vi "Missing System Controls Installer.vi"() -> ()   [LabVIEW 2009]
uses:
  <vilib>/registry/registry.llb/Registry RtKey.ctl
  <vilib>/registry/registry.llb/Registry SAM.ctl
  <vilib>/Palette API/Palette Menu/Public Type Define/Item.ctl
  <vilib>/registry/registry.llb/Read Registry Value Simple STR.vi
  <vilib>/Palette API/Palette Menu/Public Type Define/Palette type.ctl
  <vilib>/Palette API/Palette Menu/Palette Menu.lvlib
panel:
  in  "Install Button":bool
  in  "Vertical Cancel Button":bool
  in  "Select version(s) to install into:":i32[](listbox)
  # "Missing System \nControls"
  # "This VI will install the Missing System Control palette set into the version of LabVIEW you choose.\n\nAll of the necessary files have been stored in the form of block diagram data for ease of portability.\n\nNote: run this VI at your own risk - it will modify your palettes.  I can't guarantee it won't do something you don't want it to."
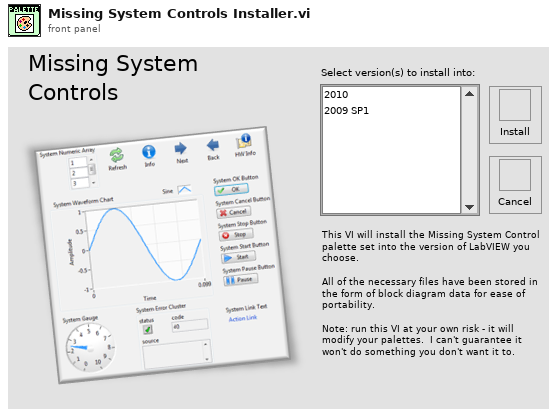
[diagram p1: front panel]
types:
  T1 = typedef "Palette Menu.lvlib/Item.ctl" = cluster{"item path":path, "library path (.lvlib)":path, "use default lvlib palette":bool, "short name":string, "place VI contents":bool, "hide synchronized item":bool, "reserve spot for synch item":bool}
  T2 = typedef "Registry SAM.ctl" = enum32{"KEY_QUERY_VALUE", "KEY_SET_VALUE", "KEY_CREATE_SUB_KEY", "KEY_ENUMERATE_SUB_KEYS", "KEY_NOTIFY", "KEY_CREATE_LINK", "KEY_READ", "KEY_WRITE", "KEY_ALL_ACCESS", "KEY_READ | KEY_WRITE"}
  T3 = typedef "Registry RtKey.ctl" = enum32{"HKEY_CLASSES_ROOT", "HKEY_CURRENT_USER", "HKEY_LOCAL_MACHINE", "HKEY_USERS", "HKEY_PERFORMANCE_DATA", "HKEY_CURRENT_CONFIG", "HKEY_DYN_DATA"}
  T4 = typedef "Registry refnum.ctl" = refnum<k1>
  T5 = cluster{"numSubKeys":i32, "maxSubKeyLen":i32, "maxSubKeyClassLen":i32}
  T6 = typedef "Palette Menu.lvlib/Palette type.ctl" = i32
  T7 = typedef "Palette Menu.lvlib/Palette Data.ctl" = cluster{"display name":string, "view format":T8, "palette width":i16, "items":T9, "256 color icon":picture, "B&W color icon":picture, "help information":T10, "palette description":string, "synchronize information":T11}
  T8 = typedef "Palette Menu.lvlib/View Format.ctl" = u16
  T9 = typedef "Palette Menu.lvlib/Items.ctl" = T1[]
  T10 = typedef "Palette Menu.lvlib/Help Info.ctl" = cluster{"help tag":string, "help file path ":path}
  T11 = typedef "Palette Menu.lvlib/Synchronize Info.ctl" = cluster{"synchronize with directory":bool, "synchronize directory path":path}
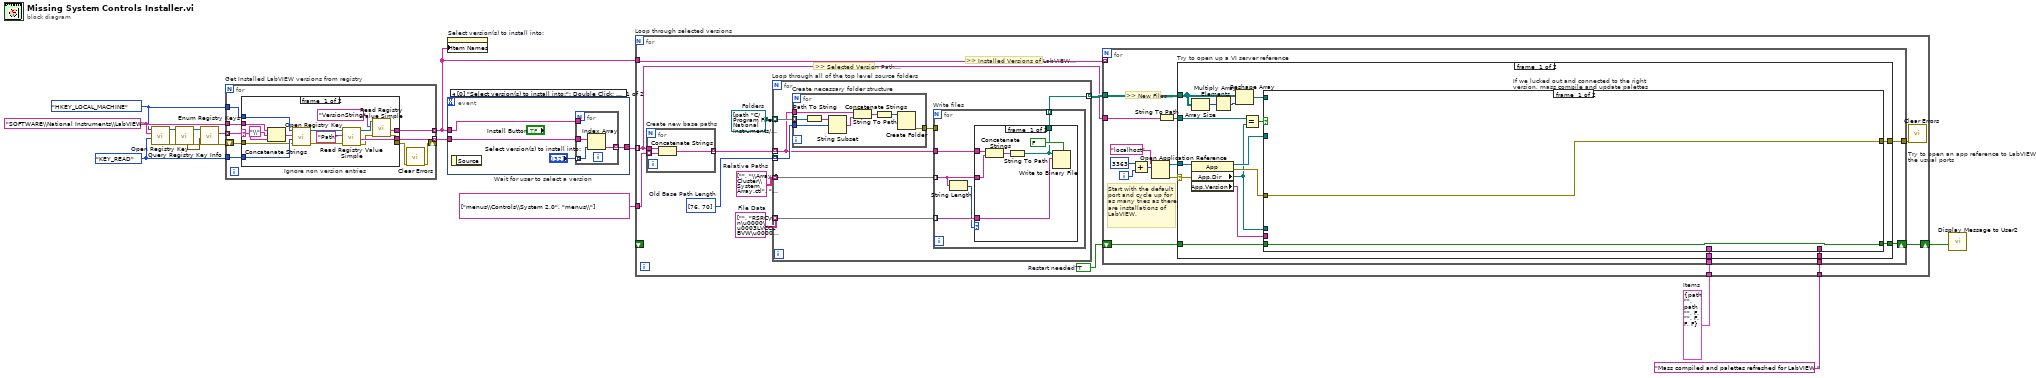
[diagram p0: block diagram]
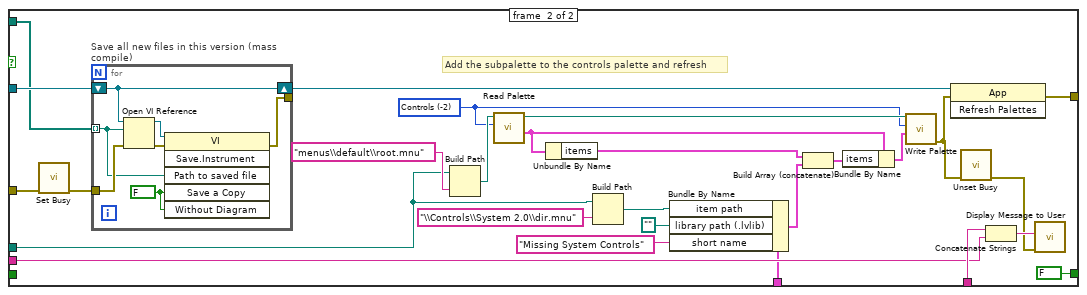
[diagram p2: hidden frame]
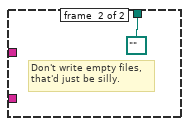
[diagram p4: hidden frame]
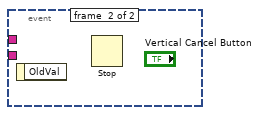
[diagram p5: hidden frame]
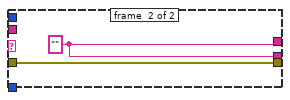
[diagram p6: hidden frame]
diagram:
  w2 = T1 {"item path"=path "", "library path (.lvlib)"=path "", "use default lvlib palette"=FALSE, "short name"="", "place VI contents"=FALSE, "hide synchronized item"=FALSE, "reserve spot for synch item"=FALSE}  # Items
  w11 = Registry_SAM."KEY_READ" ("security access mask (KEY_READ | KEY_WRITE)")
  w12 = Registry_RtKey."HKEY_LOCAL_MACHINE" ("root key (HKEY_LOCAL_MACHINE)")
  w13 = "SOFTWARE\\National Instruments\\LabVIEW" ("subkey")
  n1 = call <vilib>:"Open Registry Key.vi"("security access mask (KEY_READ | KEY_WRITE)"=w11, "subkey"=w13, "root key (HKEY_LOCAL_MACHINE)"=w12) -> ("error out"=w7:errorcluster, "refnum out"=w16:T4)  [unwired: 7 in]
  n2 = call <vilib>:"Query Registry Key Info.vi"("error in (no error)"=w7, "refnum"=w16) -> ("error out"=w6:errorcluster, "refnum out"=w15:T4, "subkey info"=w14:T5)  [unwired: 5 in, 2 out]
  n3 = call <vilib>:"Enum Registry Keys.vi"("error in (no error)"=w6, "subkey info"=w14, "refnum"=w15) -> ("error out"=w5:errorcluster, "subkeys"=w17:string[])  [unwired: 6 in, 1 out]
  n4 = for "Get Installed LabVIEW versions from registry" {
    tunnel: w17 -> [w26] mode=indexing
    tunnel: w13 -> [w25]
    tunnel: w12 -> [w24]
    tunnel: w11 -> [w23]
    tunnel: [w22] -> w8 mode=indexing
    tunnel: [w21] -> w4 mode=indexing
    shift-right: [w18] -> _
    shift-left: w5 -> [w20]
    n5 = case "Ignore non version entries" shown="Default" w26 {
      selector: w26 -> [w32 _]
      tunnel: w25 -> [w42 _]
      tunnel: w24 -> [w40 _]
      tunnel: w23 -> [w39 _]
      tunnel: [w36 w44] -> w22
      tunnel: [w33 w44] -> w21
      tunnel: w20 -> [w30 w43]
      tunnel: [w27 w43] -> w19
      frame #0 {
        n6 = Concatenate Strings(w42, "\\" ("string"), w32) -> (w41:string)
        n7 = call <vilib>:"Open Registry Key.vi"("error in (no error)"=w30, "security access mask (KEY_READ | KEY_WRITE)"=w39, "subkey"=w41, "root key (HKEY_LOCAL_MACHINE)"=w40) -> ("error out"=w29:errorcluster, "refnum out"=w38:T4)  [unwired: 6 in]
        n8 = call-poly <vilib>:"Read Registry Value Simple.vi"("error in (no error)"=w29, "value"="Path" ("subkey"), "refnum"=w38) -> ("error out"=w28:errorcluster, "String/Binary data"=w36:string, "refnum out"=w35:T4)  [unwired: 3 in, 1 out]
        n9 = call-poly <vilib>:"Read Registry Value Simple.vi"("error in (no error)"=w28, "value"="VersionString" ("subkey"), "refnum"=w35) -> ("error out"=w27:errorcluster, "String/Binary data"=w33:string)  [unwired: 3 in, 2 out]
      }
      frame #1 {
        w44 = "" ("String/Binary data")
      }
    }
    n10 = call <vilib>:"Clear Errors.vi"("error in (no error)"=w19) -> ("error out"=w18:errorcluster)  [unwired: 6 in]
  }
  n11 = event "Wait for user to select a version" shown="[0] \"Select version(s) to install into:\": Double Click;  \"Install Button\": Value Change" {
    selector: _ -> [_ _]
    dyn-events: _ -> [_ _]
    timeout: _ -> [_ _]
    tunnel: [w48 _] -> w10
    tunnel: w8 -> [w47 _]
    tunnel: w4 -> [w46 _]
    event #0 {
      n12 = event-data() -> ()  [unwired: 1 in, 1 out]
      n13 = for {
        tunnel: [w51] -> w48 mode=indexing
        tunnel: w47 -> [w50]
        tunnel: w46 -> [_]
        tunnel: "Select version(s) to install into:" -> [w49] mode=indexing
        n14 = Index Array(array=w50, index=w49) -> (element=w51:string)
      }
    }
    event #1 {
      n15 = event-data() -> ()  [unwired: 1 in, 1 out]
      n16 = Stop() -> ()  [unwired: 1 in]
    }
  }
  n17 = property on="Select version(s) to install into:" class="LstBox (strict)"("Item Names"=w4) -> ()  [unwired: 2 in, 2 out]
  n18 = for "Loop through selected versions" {
    tunnel: w10 -> [w57] mode=indexing
    tunnel: string[] ["menus\\Controls\\System 2.0", "menus\\"] -> [w60]
    tunnel: w4 -> [w56]
    tunnel: "Mass compiled and palettes refreshed for LabVIEW " -> [w55]
    tunnel: w2 -> [w54]
    shift-right: [w53] -> w1
    shift-left: _ -> [_]
    w52 = TRUE  # Restart needed?
    w65 = string[][] [["", "\\Array & Cluster\\System Array.ctl", "\\Array & Cluster\\System Cluster.ctl", "\\Array & Cluster\\System Error In.ctl", "\\Array & Cluster\\System Error Out.ctl", "\\Array & Cluster\\System Numeric Array.ctl", "\\Array & Cluster\\System String Array.ctl", "\\Boolean\\System Link Text.ctl", "\\Boolean\\System Buttons\\System Back Button.ctl", "\\Boolean\\System Buttons\\System Cancel Button.ctl", "\\Boolean\\System Buttons\\System Email Button.ctl", "\\Boolean\\System Buttons\\System Info Button.ctl", "\\Boolean\\System Buttons\\System Load Button.ctl", "\\Boolean\\System Buttons\\System Next Button.ctl", "\\Boolean\\System Buttons\\System OK Button.ctl", "\\Boolean\\System Buttons\\System Open Button.ctl", "\\Boolean\\System Buttons\\System Pause Button.ctl", "\\Boolean\\System Buttons\\System Print Button.ctl", "\\Boolean\\System Buttons\\System Refresh Button.ctl", "\\Boolean\\System Buttons\\System Save Button.ctl", "\\Boolean\\System Buttons\\System Save Data Button.ctl", "\\Boolean\\System Buttons\\System Settings Button.ctl", "\\Boolean\\System Buttons\\System Start Button.ctl", "\\Boolean\\System Buttons\\System Stop Button.ctl", "\\Boolean\\Vertical Buttons\\Vertical Add Button.ctl", "\\Boolean\\Vertical Buttons\\Vertical Back Button.ctl", "\\Boolean\\Vertical Buttons\\Vertical Cancel Button.ctl", "\\Boolean\\Vertical Buttons\\Vertical Filter Button.ctl", "\\Boolean\\Vertical Buttons\\Vertical HW Info Button.ctl", "\\Boolean\\Vertical Buttons\\Vertical Info Button.ctl", "\\Boolean\\Vertical Buttons\\Vertical Load Button.ctl", "\\Boolean\\Vertical Buttons\\Vertical Mail Button.ctl", "\\Boolean\\Vertical Buttons\\Vertical Next Button.ctl", "\\Boolean\\Vertical Buttons\\Vertical OK Button.ctl", "\\Boolean\\Vertical Buttons\\Vertical Open Button.ctl", "\\Boolean\\Vertical Buttons\\Vertical Pause Button.ctl", "\\Boolean\\Vertical Buttons\\Vertical Print Button.ctl", "\\Boolean\\Vertical Buttons\\Vertical Record Button.ctl", "\\Boolean\\Vertical Buttons\\Vertical Refresh Button.ctl", "\\Boolean\\Vertical Buttons\\Vertical Remove Button.ctl", "\\Boolean\\Vertical Buttons\\Vertical Save Button.ctl", "\\Boolean\\Vertical Buttons\\Vertical Settings Button.ctl", "\\Boolean\\Vertical Buttons\\Vertical Start Button.ctl", "\\Boolean\\Vertical Buttons\\Vertical Stop Button.ctl", "\\Graphs & Charts\\System Intensity Chart.ctl", "\\Graphs & Charts\\System Waveform Chart.ctl", "\\Graphs & Charts\\System Waveform Graph.ctl", "\\Graphs & Charts\\System XY Graph.ctl", "\\Numeric\\System Dial.ctl", "\\Numeric\\System Gauge.ctl", "\\Numeric\\System Meter.ctl", "\\String & Path\\System String (Transparent).ctl"], ["\\Controls\\System 2.0\\dir.mnu", "\\Controls\\System 2.0\\Array & Cluster\\dir.mnu", "\\Controls\\System 2.0\\Boolean\\dir.mnu", "\\Controls\\System 2.0\\Boolean\\System Buttons\\dir.mnu", "\\Controls\\System 2.0\\Boolean\\Vertical Buttons\\dir.mnu", "\\Controls\\System 2.0\\Graphs & Charts\\dir.mnu", "\\Controls\\System 2.0\\Numeric\\dir.mnu", "\\Controls\\System 2.0\\String & Path\\dir.mnu", "", "", "", "", "", "", "", "", "", "", "", "", "", "", "", "", "", "", "", "", "", "", "", "", "", "", "", "", "", "", "", "", "", "", "", "", "", "", "", "", "", "", "", ""]]  # Relative Paths
    w64 = string[][] [["", "RSRC\r\n\u0000\u0003LVCCLBVW\u0000\u0000'\u0000\u0000\u0003©\u0000\u0000\u0000 \u0000\u0000'd\u0000\u0000\u0000x\t\u0000\u0000\u0000\u0000\u0000\u0000 \u0000\u0000\u0000\u0000\u0000\u0000\u0004\u0000\u0003\u0000<\u0000¼\u0000\u001f@\u0000\u0002\u0000\u0000\u0000\u0000\u0001\u0000\u0001\u0000\u0006ÿÿÿÿ\u0000\u0000\u0000\u0000\u0000\u0000\u0000\u0000\u0000\u0000\u0000\u0000íNñw\u000e)rD.ÆRHÞÌ\u0000\u0000\u0000\n\u0000\u0000\u0000\u0010\u0000\u0000\u0000\u00007Nk½=¢©HÉÝ½#×YÔ\u001dÙ\u0000²\u0004é\tìøB~\u0000\u0000@\u0000\u0000\u0000\u0000\u0000\u0000\u0000\u0000\u0010\u0000\u0000\u0000\u0000\u0000\u0000\u0000\u0000\u0000\u0000\u0000\u0000\u0000\u0000\u0000\u0000\u0000\u0000\u0000 \u0000\u0001LVCC\u0010System Array.ctl\u0000\u0000\u0000\u0000\u0000\u0000\u0000\u0000\u0003\u0000\u0000\u0000\u0002\u0000\u0001\u0000\u0000\u0000\u0000\u0000\u0014\u0000\b\u0000\u0002\u0010\u0000\u0010\u0001 \u0000\u0010\u0000\u0000\u0004\u0010\u00000\u0000\u0010\u0000\u0000\u0000\u0000F\u0000\u0000\u0001,xc`À\u0004ÿ\u0000H12007\u0000i6tñÿPE+Å\u0000Ù\\lv\u0010a/#\u000e\u001an\u0004\u0003\u0003Ó\u0013 Í\u0002Á i¦\u000f@ü\u0003¡\u0013Á\u0000³> [\u0000\u0000\u0000\u0000\u0000 \u0000\u0001VIDS\u0010System Array.ctl\u0000\u0000\u0000\u0000\u0000\u0000\u0000\u0000\u0003\u0000\u0000\u0000x\u0000\u0000\u0000´xsd``È4¶0«`@äüT\u0010½\u0000_3ÄÇEEFÇ\u001e\u0010Ú£Â\u0011\u001c\u0018\u0014\u0016¾\u0011()Ü]Ê°C\u000b(Óé¦±C\tL;ìp\u0004Ó.¡/@æõ¦¨°À´e\u0000ù\u0007æú\u000f\u0004 yF\u0006f\u0006px$·8û»¸\"qÁn\u0002\u00004A'Y\u0000\u0000\u0000\r\t\u0001\u0011\u0000\u0000\u00059.0.1\u0000\u0000\u0000\u0000\u0000\u0000\u0000\u0000\u0000\u0000\u0000\u0000\u0000\u0000\u0000\u0000\u0000\u0000\u0000\u001f÷ÿÿ\u0010\u0014\u0000\u0000\u0011\u0014Fx\u0010\u0014É\u0010\u0011\u0014B0\u0011\u0014D\b\u0011\u0014ïp\u0010\u0014\u0000\u0000\u001fô\u0000\u0000\u0010\u0017ÿÿ\u0011\u0010\u0000\u0000\u0010\u0010\u0000\u0000\u0011\u0010\u0000\u0000\u0011\u0010\u0000\u0000\u0013\u0010\u0000\u0000\u0010\u0010\u0000\u0000\u001fð\u0000\u0000\u0010\u0010\u0000\u0000\u0012\u0010\u0000\u0000\u0012\u0010\u0000\u0000\u0012\u0000\u0000...", "RSRC\r\n\u0000\u0003LVCCLBVW\u0000\u00007\f\u0000\u0000\u0003«\u0000\u0000\u0000 \u0000\u00006ì\u0000\u0000\u0000x\t\u0000\u0000\u0000\u0000\u0000\u0000 \u0000\u0000\u0000\u0000\u0000\u0000\u0004\u0000\u0003\u0000<\u0000¼\u0000\u001f@\u0000\u0002\u0000\u0000\u0000\u0000\u0001\u0000\u0001\u0000\u0006ÿÿÿÿ\u0000\u0000\u0000\u0000\u0000\u0000\u0000\u0000\u0000\u0000\u0000\u0000\u0006D\u0007ÿÅLí\u0003rÈ\rÞ\u0000\u0000\u0000\n\u0000\u0000\u0000\u0010\u0000\u0000\u0000\u0000ÿ\n.íüN\u0013\u001aõÇä?Ô\u001dÙ\u0000²\u0004é\tìøB~\u0000\u0000@\u0000\u0000\u0000\u0000\u0000\u0000\u0000\u0000\u0010\u0000\u0000\u0000\u0000\u0000\u0000\u0000\u0000\u0000\u0000\u0000\u0000\u0000\u0000\u0000\u0000\u0000\u0000\u0000\"\u0000\u0001LVCC\u0012System Cluster.ctl\u0000\u0000\u0000\u0000\u0000\u0000\u0000\u0000\u0003\u0000\u0000\u0000\u0000\u0000\u0002\u0000\u0001\u0000\u0000\u0000\u0000\u0000\u0010\u0000\u0006\u0000\u0002\u0010\u0000\u0010\u0001\u0010\u0000\u0010\u00040\u0000\u0010\u0000\u0000\u0000\u0000<\u0000\u0000\u0001\u0010xc`À\u0004ÿ\u0000H1200¸,èâÿ¡\u0000V\u0001²¹Øì Î^F \u001a¦/\fP\u000f@\u00003*\u0017\bØ°è\u0004\u0000Úç\u001dó\u0000\u0000\u0000\"\u0000\u0001VIDS\u0012System Cluster.ctl\u0000\u0000\u0000\u0000\u0000\u0000\u0000\u0000\u0003\u0000\u0000\u0000\u0000\u0000x\u0000\u0000\u0000´xsd``È4¶0«`@äüT\u0010½\u0000_3ÄÇEEFÇ\u001e\u0010Ú£Â\u0011\u001c\u0018\u0014\u0016¾\u0011()Ü]Ê°C\u000b(Óé¦±C\tL;ìp\u0004Ó.¡/@æõ¦¨°À´e\u0000ù\u0007æú\u000f\u0004 yF\u0006f\u0006px$·8û»¸\"qÁn\u0002\u00004A'Y\u0000\u0000\u0000\u000b\t\u0000$\u0000\u0000\u00039.0\u0000\u0000\u0000\u0000\u0000\u0000\u0000\u0000\u0000\u0000\u0000\u0000\u0000\u0000\u0000\u0000\u0000\u0000\u0000\u0000\u0000?ÿÿþ \u0000\u0000\u0002 \u0000\u0000\u0002 \u0000\u0000\u0002#ÿâ\"\u0000\"\"\u0000\"#ÿâ \u0000\u0000\u0002 \u0000\u0000\u0002 ?ð\u0002  \u0010\u0002  \u0010\u0002 ?ð\u0002 \u0000\u0000\u0002 \u0000\u0000\u0002 \u0000\u0000\u0002 \u0000â!ðâ!ðâ!ðâ!ð\u0000\u0002 \u0000\u0000\u0002...", "RSRC\r\n\u0000\u0003LVCCLBVW\u0000\u0000p\u0000\u0000\u0003à\u0000\u0000\u0000 \u0000\u0000P\u0000\u0000\u0000x\t\u0000\u0000\u0000\u0000\u0000\u0000 \u0000\u0000\u0000\u0000\u0000\u0000\u0004\u0000\u0003\u0000<\u0000¼\u0000\u001f@\u0000\u0002\u0000\u0000\u0000\u0000\u0001\u0000\u0001\u0000\u0006ÿÿÿÿ\u0000\u0000\u0000\u0000\u0000\u0000\u0000\u0000\u0000\u0000\u0000\u0000~ýë¥\u0007\u000bNW\u0007í÷\u001cÜÞ\u0000\u0000\u0000\n\u0000\u0000\u0000\u0010\u0000\u0000\u0000\u0000S\u0017×ûE¶Ö¯tµ.RqÔ\u001dÙ\u0000²\u0004é\tìøB~\u0000\u0000@\u0000\u0000\u0000\u0000\u0000\u0000\u0000\u0000\u0010\u0000\u0000\u0000\u0000\u0000\u0000\u0000\u0000\u0000\u0000\u0000\u0000\u0000\u0000\u0000\u0000\u0000\u0000\u0000\"\u0000\u0001LVCC\u0013System Error In.ctl\u0000\u0000\u0000\u0000\u0000\u0000\u0000\u0003\u0000\u0000\u0000\u0000\u0000\u0002\u0000\u0001\u0000\u0000\u0000\u0000\u0000\u0014\u0000\b\u0000\u0002\u0010\u0000\u0010\u0001\u0010\u0000\u0000\u0004\u0010\u00000\u0000\u0000\b\u0010\u0000\u0000\u0000\u0000@\u0000\u0000\u0001\u0019xc`À\u0004ÿ\u0000H12007\u0000iVtñÿPE+Å\u0000Ù\\lvj/P1Ó\u0005 Í\fÄ\u0010!¦;@ü\u000eY\u0011\u000f\u0016\u0000ê &\u0000\u0000\u0000\"\u0000\u0001VIDS\u0013System Error In.ctl\u0000\u0000\u0000\u0000\u0000\u0000\u0000\u0003\u0000\u0000\u0000\u0000\u0000ê\u0000\u0000\u0001pxûÄÀÀila¦ÉÈ\u0000\u0007Éù)© :\u0006(ö!>.*2:öðÐî\u001c\u0015àÀ °ðî\u0012\u0015î\u001a\u0015óNp00@D]9:]ÿt»òtºþè.ýÓ]û\u001f\u001bÿ>y\u001b;@f°î\u0000Y\næ1ºþÒPµÝöÝfÿPTZï`ªdAVùßü¿Ù\u000bÞ\u0014\u0015\u000e[\u0010\u0003E\u0017+\u0007vôÉÃ\u0013ÂÃ^Dÿÿÿ\u001f¤\u0014?J\u0019vh\u0001\u0015wºiìP\u0002Ó\u000e;>iP\r,0mÛ|\u0013&\u0006\u0006I ñ\u0007\u0018d\u000bÐäÿ u\fÌ@Q\u0000)\u0010ÀÙßÅ\u0015\u000f\nO\u0000ø@cC\u0000\u0000\u0000\u0000\u0000\u000b...", "RSRC\r\n\u0000\u0003LVCCLBVW\u0000\u0000Ô\u0000\u0000\u0003á\u0000\u0000\u0000 \u0000\u0000´\u0000\u0000\u0000x\t\u0000\u0000\u0000\u0000\u0000\u0000 \u0000\u0000\u0000\u0000\u0000\u0000\u0004\u0000\u0003\u0000<\u0000¼\u0000\u001f@\u0000\u0002\u0000\u0000\u0000\u0000\u0001\u0000\u0001\u0000\u0006ÿÿÿÿ\u0000\u0000\u0000\u0000\u0000\u0000\u0000\u0000\u0000\u0000\u0000\u0000³>Í¶\u0010KÙ@Ì\u0001\u0017\u001d\u0000\u0000\u0000\u0000\n\u0000\u0000\u0000\u0010\u0000\u0000\u0000\u0000:\u0007ðvÝ<éF°YÖ~ÂÈÔ\u001dÙ\u0000²\u0004é\tìøB~\u0000\u0000@\u0000\u0000\u0000\u0000\u0000\u0000\u0000\u0000\u0010\u0000\u0000\u0000\u0000\u0000\u0000\u0000\u0000\u0000\u0000\u0000\u0000\u0000\u0000\u0000\u0000\u0000\u0000\u0000$\u0000\u0001LVCC\u0014System Error Out.ctl\u0000\u0000\u0000\u0000\u0000\u0000\u0000\u0000\u0003\u0000\u0000\u0000\u0002\u0000\u0001\u0000\u0000\u0000\u0000\u0000\u0014\u0000\b\u0000\u0002\u0010\u0000\u0010\u0001\u0010\u0000\u0000\u0004\u0010\u00000\u0000\u0000\b\u0010\u0000\u0000\u0000\u0000B\u0000\u0000\u0001\u0019xc`À\u0004ÿ\u0000H12007\u0000iVtñÿPE+Å\u0000Ù\\lvj/P1Ó\u0005 Í\fÄ`?10Ý\u0001âwÈx°h\u0004\u0000\u0014 '\u0000\u0000\u0000\u0000\u0000$\u0000\u0001VIDS\u0014System Error Out.ctl\u0000\u0000\u0000\u0000\u0000\u0000\u0000\u0000\u0003\u0000\u0000\u0000ê\u0000\u0000\u0001pxûÄÀÀila¦ÉÈ\u0000\u0007Éù)© :\u0006(ö!>.*2:öðÐî\u001c\u0015àÀ °ðî\u0012\u0015î\u001a\u0015óNp00@D]9:]ÿt»òtºþè.ýÓ]û\u001f\u001bÿ>y\u001b;@f°î\u0000Y\næ1ºþÒPµÝöÝfÿPTZï`ªdAVùßü¿Ù\u000bÞ\u0014\u0015\u000e[\u0010\u0003E\u0017+\u0007vôÉÃ\u0013ÂÃ^Dÿÿÿ\u001f¤\u0014?J\u0019vh\u0001\u0015wºiìP\u0002Ó\u000e;>iP\r,0mÛ|\u0013&\u0006\u0006I ñ\u0007\u0018d\u000bÐäÿ u\fÌ@Q\u0000)\u0010ÀÙßÅ\u0015\u000f\nO\u0000ø@cC\u0000\u0000...", "RSRC\r\n\u0000\u0003LVCCLBVW\u0000\u0000I\u0000\u0000\u0003±\u0000\u0000\u0000 \u0000\u0000I`\u0000\u0000\u0000x\t\u0000\u0000\u0000\u0000\u0000\u0000 \u0000\u0000\u0000\u0000\u0000\u0000\u0004\u0000\u0003\u0000<\u0000¼\u0000\u001f@\u0000\u0002\u0000\u0000\u0000\u0000\u0001\u0000\u0001\u0000\u0006ÿÿÿÿ\u0000\u0000\u0000\u0000\u0000\u0000\u0000\u0000\u0000\u0000\u0000\u0000ÑµÎ§íy\u0019Lªc},Ó:+T\u0000\u0000\u0000\n\u0000\u0000\u0000\u0010\u0000\u0000\u0000\u0000\"¡à,\u001b&K¥-\u000fcÝsÔ\u001dÙ\u0000²\u0004é\tìøB~\u0000\u0000@\u0000\u0000\u0000\u0000\u0000\u0000\u0000\u0000\u0010\u0000\u0000\u0000\u0000\u0000\u0000\u0000\u0000\u0000\u0000\u0000\u0000\u0000\u0000\u0000\u0000\u0000\u0000\u0000(\u0000\u0001LVCC\u0018System Numeric Array.ctl\u0000\u0000\u0000\u0000\u0000\u0000\u0000\u0000\u0003\u0000\u0000\u0000\u0002\u0000\u0001\u0000\u0000\u0000\u0000\u0000\"\u0000\u000f\u0000\u0002\u0010\u0000\u0010\u0001 \u0000\u0010\u0000\u0000\u0004\u0010\u00000\u0000\u0000\b\u0010\u0000\u0010\b\u0010\u0000\u0010\u0000\u0010\u0000\u0010\u0000\u0010\u0000\u0000\u0000\u0000\u0000\u0000H\u0000\u0000\u00014xc`À\u0004ÿ\u0000H12007\u0000i6tñÿPE+Å\u0000Ù\\lv\u0010a/#\u000e\u001aÃ(\u0006\u0006¦'@\u0005é\u0003\u0010ÿÊs\u0000\u00199±h\u0004\u0000 b\u0000\u0000\u0000(\u0000\u0001VIDS\u0018System Numeric Array.ctl\u0000\u0000\u0000\u0000\u0000\u0000\u0000\u0000\u0003\u0000\u0000\u0001\u000b\u0000\u0000\u0001Ìx\u000bcd`È4¶0ë\u0005Ò0\n¢w\u0000Å^3ÄÇEEFÇ\u001e\u0010Ú£Â\u0011\u001c\u0018\u0014\u0016Þ]¢¢Ò]£¢ÑÍf\u000bRV*}¼õ\u00043Dë>\u0010q¼õ\u0000ûZ´¡óXó1nÎ¹ ÁÎ¹ Ýì`%ò@ÙãÍÇ²Ö`ÙZ6*M°ª×\\\bºÁâ/ËÌ\tT\u0005wÙî²ß<yïfÀý\u0007ó\"ªÙ\f\u000f´¼}Í±\u0003d%ÿ\u0003Uú¥ºÍÇ8sx7ÿf¨¿Ü¼\u0017ìOP¸0°UAJYÁXÂªa\u0016P¦ÓMc...", "RSRC\r\n\u0000\u0003LVCCLBVW\u0000\u0000B\b\u0000\u0000\u0003°\u0000\u0000\u0000 \u0000\u0000Aè\u0000\u0000\u0000x\t\u0000\u0000\u0000\u0000\u0000\u0000 \u0000\u0000\u0000\u0000\u0000\u0000\u0004\u0000\u0003\u0000<\u0000¼\u0000\u001f@\u0000\u0002\u0000\u0000\u0000\u0000\u0001\u0000\u0001\u0000\u0006ÿÿÿÿ\u0000\u0000\u0000\u0000\u0000\u0000\u0000\u0000\u0000\u0000\u0000\u0000üi\u001e¶\u0003\rQB\u0004va\u0010Éá\u0000\u0000\u0000\n\u0000\u0000\u0000\u0010\u0000\u0000\u0000\u0000àÉ½þ^P{KÒz;ù\u0012__Ô\u001dÙ\u0000²\u0004é\tìøB~\u0000\u0000@\u0000\u0000\u0000\u0000\u0000\u0000\u0000\u0000\u0010\u0000\u0000\u0000\u0000\u0000\u0000\u0000\u0000\u0000\u0000\u0000\u0000\u0000\u0000\u0000\u0000\u0000\u0000\u0000&\u0000\u0001LVCC\u0017System String Array.ctl\u0000\u0000\u0000\u0000\u0000\u0000\u0000\u0003\u0000\u0000\u0000\u0000\u0000\u0002\u0000\u0001\u0000\u0000\u0000\u0000\u0000\u0016\u0000\t\u0000\u0002\u0010\u0000\u0010\u0001 \u0000\u0010\u0000\u0000\u0004\u0010\u00000\u0000\u0000\b\u0010\u0000\u0000\u0000\u0000\u0000\u0000H\u0000\u0000\u00010xc`À\u0004ÿ\u0000H12007\u0000i6tñÿPE+Å\u0000Ù\\lv\u0010a/#\u000e\u001aÅ\u0018\u0006\u0006¦'@\u0005é\u0003\u0010ÿÊ\u0003ÅX\u0018ù°h\u0004\u0000%· c\u0000\u0000\u0000&\u0000\u0001VIDS\u0017System String Array.ctl\u0000\u0000\u0000\u0000\u0000\u0000\u0000\u0003\u0000\u0000\u0000\u0000\u0001\u0015\u0000\u0000\u0001àxKbd`È4¶0\t¤a 9?%\u0015D\u0001½f=<!´;G#80(,¼»DE¥»FEã%\u001fPÁ\t\u0011\u0006\u0006¨+G7-H_©èq×/ Æ>\u0010qÜõ\u000fzÍßÍÐy¬ù\u0018K·EgíÎÚ/Ý®<Põ%b@©ÃÍRÖµjòµ_^³Cuv×þyY\u0003¤'Ð\u0002ü7þoö\u0002dKo\n\u0007Ø5;@!QÂº\u0003ì\u0013u \u000eóoþÏP¥¹ö\u000b,_Ê\n\u0016\u0001\u0007ÒÉÃ\u0013ÂÃ^¼þ÷ÿ?È0,áVÊ°C\u000b¨¸ÓMc\u0012v...", "RSRC\r\n\u0000\u0003LVCCLBVW\u0000\u0000Q\u0018\u0000\u0000\u0003­\u0000\u0000\u0000 \u0000\u0000Pø\u0000\u0000\u0000x\t\u0000\u0000\u0000\u0000\u0000\u0000 \u0000\u0000\u0000\u0000\u0000\u0000\u0004\u0000\u0003\u0000<\u0000¼\u0000\u001f@\u0000\u0002\u0000\u0000\u0000\u0000\u0001\u0000\u0001\u0000\u0006ÿÿÿÿ\u0000\u0000\u0000\u0000\u0000\u0000\u0000\u0000\u0000\u0000\u0000\u0000íè´C÷%C¸ÑÝX\u0011<l\u001a\u0000\u0000\u0000\n\u0000\u0000\u0000\u0010\u0000\u0000\u0000\u0000\u001a\u0013ºNÎ{àH¨W\u0012Æs¡{óÔ\u001dÙ\u0000²\u0004é\tìøB~\u0000\u0000@\u0000\u0000\u0000\u0000\u0000\u0000\u0000\u0000\u0010\u0000\u0000\u0000\u0000\u0000\u0000\u0000\u0000\u0000\u0000\u0000\u0000\u0000\u0000\u0000\u0000\u0000\u0000\u0000$\u0000\u0001LVCC\u0014System Link Text.ctl\u0000\u0000\u0000\u0000\u0000\u0000\u0000\u0000\u0003\u0000\u0000\u0000\u0002\u0000\u0001\u0000\u0000\u0000\u0000\u0000\u0014\u0000\b\u0000\u0002\u0010\u0000\u0010\u0001\u0010\u0000\u0010\u0004\u0010\u00000\u0000\u0010\b\u0010\u0000\u0000\u0000\u0000A\u0000\u0000\u0001\u0011xc`À\u0004ÿ\u0000H12007\u0000iVtñÿPE+Å\u0000Ù\\lv\u0010i/#P\u0011Ó\u0007 \u0001ì\u0011\u0010fú\u0003ÄÿPTaÑ\t\u0000´Ò e\u0000\u0000\u0000\u0000\u0000\u0000$\u0000\u0001VIDS\u0014System Link Text.ctl\u0000\u0000\u0000\u0000\u0000\u0000\u0000\u0000\u0003\u0000\u0000\u0000\u0000\u0000\u0000Ôxg``È4¶0Æ\u0000Éù)© ú\u0000\u0010¿f=<!´;G#80(,¼»DE¥»FE\u001f\u001bÿ>y\u001b;\u0018\nKXwô²yX42ìÐ\u0002ÊtºiìP\u0002Ó\u000e;âÁ´Kè\u000bÎÞ\u0014\u0015\u0016¶6 ÿ Ð\u001cQÿ\u0000$ÏÈÀÌËPÊPË\fý]\\ù 7\u0003\u0000Â\u000308\u0000\u0000\u0000\u0000\u0000\u0000\r\t\u0001\u0011\u0000\u0000\u00059.0.1\u0000\u0000\u0000\u0000\u0000\u0000\u0000\u0000\u0000\u0000\u0000\u0000\u0000\u0000\u0000\u0000\u0000\u0000\u0000\u0000\u0000\u0000\u0000\u0000\u0000\u0000\u0000\u0000\u0000\u0000\u0000\u0000\u0000\u0000\u0000\u0000\u0000\u0000\u0000\u0000@\u0000\u0000À\b\u0000\u0000 \b\u0000\u0001!Þ\u0001#\b\u0001\u0012\b\u0003ò\b\u0002\u0013\b...", "RSRC\r\n\u0000\u0003LVCCLBVW\u0000\u00002¨\u0000\u0000\u0003Ï\u0000\u0000\u0000 \u0000\u00002\u0000\u0000\u0000x\t\u0000\u0000\u0000\u0000\u0000\u0000 \u0000\u0000\u0000\u0000\u0000\u0000\u0004\u0000\u0003\u0000<\u0000¼\u0000\u001f@\u0000\u0002\u0000\u0000\u0000\u0000\u0001\u0000\u0001\u0000\u0006ÿÿÿÿ\u0000\u0000\u0000\u0000\u0000\u0000\u0000\u0000\u0000\u0000\u0000\u0000ñM|\u0011è(I·\u001b\u001a'«ýÑ\u0000\u0000\u0000\n\u0000\u0000\u0000\u0010\u0000\u0000\u0000\u0000yL_FÈ\nm@´\u001a\u0012Fv)SÔ\u001dÙ\u0000²\u0004é\tìøB~\u0000\u0000@\u0000\u0000\u0000\u0000\u0000\u0000\u0000\u0000\u0010\u0000\u0000\u0000\u0000\u0000\u0000\u0000\u0000\u0000\u0000\u0000\u0000\u0000\u0000\u0000\u0000\u0000\u0000\u0000&\u0000\u0001LVCC\u0016System Back Button.ctl\u0000\u0000\u0000\u0000\u0000\u0000\u0000\u0000\u0003\u0000\u0000\u0000\u0000\u0000\u0002\u0000\u0001\u0000\u0000\u0000\u0000\u0000\u0014\u0000\b\u0000\u0002\u0010\u0000\u0010\u0001\u0010\u0000\u0010\u0004\u0010\u00000\u0000\u0010\b\u0010\u0000\u0000\u0000\u0000A\u0000\u0000\u0001\u0011xc`À\u0004ÿ\u0000H12007\u0000iVtñÿPE+Å\u0000Ù\\lv\u0010i/#P\u0011Ó\u0007 \u0001ì\u0011\u0010fú\u0003ÄÿPTaÑ\t\u0000´Ò e\u0000\u0000\u0000\u0000\u0000\u0000&\u0000\u0001VIDS\u0016System Back Button.ctl\u0000\u0000\u0000\u0000\u0000\u0000\u0000\u0000\u0003\u0000\u0000\u0000\u0000\u0000\u0000\u0000\u0000Ôxg``È4¶0Æ\u0000Éù)© ú\u0000\u0010¿f=<!´;G#80(,¼»DE¥»FE\u001f\u001bÿ>y\u001b;\u0018\nKXwô²yX42ìÐ\u0002ÊtºiìP\u0002Ó\u000e;âÁ´Kè\u000bÎÞ\u0014\u0015\u0016¶6 ÿ Ð\u001cQÿ\u0000$ÏÈÀÌËPÊPË\fý]\\ù 7\u0003\u0000Â\u000308\u0000\u0000\u0000\u0000\u0000\u0000\r\t\u0001\u0011\u0000\u0000\u00059.0.1\u0000\u0000\u0000\u0000\u0000\u0000\u0000\u0000\u0000\u0000\u0000\u0000\u0000\u0000\u0000\u000fÿÿÿ\u0000\u0000\u0000\u0000 \u0000\u0000\u0000 \u0000\u0000 \u0001\u0000 \u0006\u0000 \fþ\u0000 \u001b\u0002\u0000 7ú\u0000 ú\u0000 ?þ\u0000 \u001fþ\u0000...", "RSRC\r\n\u0000\u0003LVCCLBVW\u0000\u0000. \u0000\u0000\u0003Ñ\u0000\u0000\u0000 \u0000\u0000.\u0000\u0000\u0000x\t\u0000\u0000\u0000\u0000\u0000\u0000 \u0000\u0000\u0000\u0000\u0000\u0000\u0004\u0000\u0003\u0000<\u0000¼\u0000\u001f@\u0000\u0002\u0000\u0000\u0000\u0000\u0001\u0000\u0001\u0000\u0006ÿÿÿÿ\u0000\u0000\u0000\u0000\u0000\u0000\u0000\u0000\u0000\u0000\u0000\u0000z\u001a3ëÊsI­Ïkov\u0000\u0000\u0000\n\u0000\u0000\u0000\u0010\u0000\u0000\u0000\u0000\u001dÊ·«4J¸'EtXXZÔ\u001dÙ\u0000²\u0004é\tìøB~\u0000\u0000@\u0000\u0000\u0000\u0000\u0000\u0000\u0000\u0000\u0010\u0000\u0000\u0000\u0000\u0000\u0000\u0000\u0000\u0000\u0000\u0000\u0000\u0000\u0000\u0000\u0000\u0000\u0000\u0000(\u0000\u0001LVCC\u0018System Cancel Button.ctl\u0000\u0000\u0000\u0000\u0000\u0000\u0000\u0000\u0003\u0000\u0000\u0000\u0002\u0000\u0001\u0000\u0000\u0000\u0000\u0000\u0014\u0000\b\u0000\u0002\u0010\u0000\u0010\u0001\u0010\u0000\u0010\u0004\u0010\u00000\u0000\u0010\b\u0010\u0000\u0000\u0000\u0000A\u0000\u0000\u0001\u0011xc`À\u0004ÿ\u0000H12007\u0000iVtñÿPE+Å\u0000Ù\\lv\u0010i/#P\u0011Ó\u0007 \u0001ì\u0011\u0010fú\u0003ÄÿPTaÑ\t\u0000´Ò e\u0000\u0000\u0000\u0000\u0000\u0000(\u0000\u0001VIDS\u0018System Cancel Button.ctl\u0000\u0000\u0000\u0000\u0000\u0000\u0000\u0000\u0003\u0000\u0000\u0000\u0000\u0000\u0000Ôxg``È4¶0Æ\u0000Éù)© ú\u0000\u0010¿f=<!´;G#80(,¼»DE¥»FE\u001f\u001bÿ>y\u001b;\u0018\nKXwô²yX42ìÐ\u0002ÊtºiìP\u0002Ó\u000e;âÁ´Kè\u000bÎÞ\u0014\u0015\u0016¶6 ÿ Ð\u001cQÿ\u0000$ÏÈÀÌËPÊPË\fý]\\ù 7\u0003\u0000Â\u000308\u0000\u0000\u0000\u0000\u0000\u0000\r\t\u0001\u0011\u0000\u0000\u00059.0.1\u0000\u0000\u0000\u0000\u0000\u0000\u0000\u0000\u0000\u0000\u0000\u0000\u0000\u0000\u0000\u000fÿÿÿ\u0000\u0000\u0000\u0000 \u0000\u0000\u0000 \u0000\u0000\u0000 \u0000\u0000\u0000 $$\u0000 \"D\u0000 \u0011\u0001 \b\u0010\u0002 \u0004 \u0002 \f0\u0002 \u0018\u0018\u0002...", "RSRC\r\n\u0000\u0003LVCCLBVW\u0000\u0000,h\u0000\u0000\u0003Ð\u0000\u0000\u0000 \u0000\u0000,H\u0000\u0000\u0000x\t\u0000\u0000\u0000\u0000\u0000\u0000 \u0000\u0000\u0000\u0000\u0000\u0000\u0004\u0000\u0003\u0000<\u0000¼\u0000\u001f@\u0000\u0002\u0000\u0000\u0000\u0000\u0001\u0000\u0001\u0000\u0006ÿÿÿÿ\u0000\u0000\u0000\u0000\u0000\u0000\u0000\u0000\u0000\u0000\u0000\u0000Éø|\u001fqá\u0019L©\rË2\u0016úo\u0000\u0000\u0000\n\u0000\u0000\u0000\u0010\u0000\u0000\u0000\u0000·ì@FOq7C¡\u001f°Ô\u001dÙ\u0000²\u0004é\tìøB~\u0000\u0000@\u0000\u0000\u0000\u0000\u0000\u0000\u0000\u0000\u0010\u0000\u0000\u0000\u0000\u0000\u0000\u0000\u0000\u0000\u0000\u0000\u0000\u0000\u0000\u0000\u0000\u0000\u0000\u0000&\u0000\u0001LVCC\u0017System Email Button.ctl\u0000\u0000\u0000\u0000\u0000\u0000\u0000\u0003\u0000\u0000\u0000\u0000\u0000\u0002\u0000\u0001\u0000\u0000\u0000\u0000\u0000\u0014\u0000\b\u0000\u0002\u0010\u0000\u0010\u0001\u0010\u0000\u0010\u0004\u0010\u00000\u0000\u0010\b\u0010\u0000\u0000\u0000\u0000A\u0000\u0000\u0001\u0011xc`À\u0004ÿ\u0000H12007\u0000iVtñÿPE+Å\u0000Ù\\lv\u0010i/#P\u0011Ó\u0007 \u0001ì\u0011\u0010fú\u0003ÄÿPTaÑ\t\u0000´Ò e\u0000\u0000\u0000\u0000\u0000\u0000&\u0000\u0001VIDS\u0017System Email Button.ctl\u0000\u0000\u0000\u0000\u0000\u0000\u0000\u0003\u0000\u0000\u0000\u0000\u0000\u0000\u0000\u0000Ôxg``È4¶0Æ\u0000Éù)© ú\u0000\u0010¿f=<!´;G#80(,¼»DE¥»FE\u001f\u001bÿ>y\u001b;\u0018\nKXwô²yX42ìÐ\u0002ÊtºiìP\u0002Ó\u000e;âÁ´Kè\u000bÎÞ\u0014\u0015\u0016¶6 ÿ Ð\u001cQÿ\u0000$ÏÈÀÌËPÊPË\fý]\\ù 7\u0003\u0000Â\u000308\u0000\u0000\u0000\u0000\u0000\u0000\r\t\u0001\u0011\u0000\u0000\u00059.0.1\u0000\u0000\u0000\u0000\u0000\u0000\u0000\u0000\u0000\u0000\u0000\u0000\u0000\u0000\u0000\u000fÿÿÿ\u0000\u0000\u0000\u0000 \u0000\u0000\u0000 \u0000\u0000\u0000 \u0000\u0000 \u0000\u0001\u0000 \u0000\u0001\u0000 \u0000\u0001\u0000 \u0000\u0001\u0000 \u0011\u0000 \t\u0000 Å\u0000...", "RSRC\r\n\u0000\u0003LVCCLBVW\u0000\u0000+Ì\u0000\u0000\u0003Ï\u0000\u0000\u0000 \u0000\u0000+¬\u0000\u0000\u0000x\t\u0000\u0000\u0000\u0000\u0000\u0000 \u0000\u0000\u0000\u0000\u0000\u0000\u0004\u0000\u0003\u0000<\u0000¼\u0000\u001f@\u0000\u0002\u0000\u0000\u0000\u0000\u0001\u0000\u0001\u0000\u0006ÿÿÿÿ\u0000\u0000\u0000\u0000\u0000\u0000\u0000\u0000\u0000\u0000\u0000\u0000ør·MÙþ@´²ç)×ÜY\u0000\u0000\u0000\n\u0000\u0000\u0000\u0010\u0000\u0000\u0000\u0000Hð[dÙE¶yÊy¢½Ô\u001dÙ\u0000²\u0004é\tìøB~\u0000\u0000@\u0000\u0000\u0000\u0000\u0000\u0000\u0000\u0000\u0010\u0000\u0000\u0000\u0000\u0000\u0000\u0000\u0000\u0000\u0000\u0000\u0000\u0000\u0000\u0000\u0000\u0000\u0000\u0000&\u0000\u0001LVCC\u0016System Info Button.ctl\u0000\u0000\u0000\u0000\u0000\u0000\u0000\u0000\u0003\u0000\u0000\u0000\u0000\u0000\u0002\u0000\u0001\u0000\u0000\u0000\u0000\u0000\u0014\u0000\b\u0000\u0002\u0010\u0000\u0010\u0001\u0010\u0000\u0010\u0004\u0010\u00000\u0000\u0010\b\u0010\u0000\u0000\u0000\u0000A\u0000\u0000\u0001\u0011xc`À\u0004ÿ\u0000H12007\u0000iVtñÿPE+Å\u0000Ù\\lv\u0010i/#P\u0011Ó\u0007 \u0001ì\u0011\u0010fú\u0003ÄÿPTaÑ\t\u0000´Ò e\u0000\u0000\u0000\u0000\u0000\u0000&\u0000\u0001VIDS\u0016System Info Button.ctl\u0000\u0000\u0000\u0000\u0000\u0000\u0000\u0000\u0003\u0000\u0000\u0000\u0000\u0000\u0000\u0000\u0000Ôxg``È4¶0Æ\u0000Éù)© ú\u0000\u0010¿f=<!´;G#80(,¼»DE¥»FE\u001f\u001bÿ>y\u001b;\u0018\nKXwô²yX42ìÐ\u0002ÊtºiìP\u0002Ó\u000e;âÁ´Kè\u000bÎÞ\u0014\u0015\u0016¶6 ÿ Ð\u001cQÿ\u0000$ÏÈÀÌËPÊPË\fý]\\ù 7\u0003\u0000Â\u000308\u0000\u0000\u0000\u0000\u0000\u0000\r\t\u0001\u0011\u0000\u0000\u00059.0.1\u0000\u0000\u0000\u0000\u0000\u0000\u0000\u0000\u0000\u0000\u0000\u0000\u0000\u0000\u0000\u000fÿÿÿ\u0000\u0000\u0000\u0000 \u0000\u0000\u0000 \u0003À\u0000 \b\u0010\u0000 \u0010\b\u0000  \u0004\u0000 2D\u0000 þ\u0000 |~\u0000 ~~\u0000 ~~\u0000...", "RSRC\r\n\u0000\u0003LVCCLBVW\u0000\u00008Ô\u0000\u0000\u0003Ï\u0000\u0000\u0000 \u0000\u00008´\u0000\u0000\u0000x\t\u0000\u0000\u0000\u0000\u0000\u0000 \u0000\u0000\u0000\u0000\u0000\u0000\u0004\u0000\u0003\u0000<\u0000¼\u0000\u001f@\u0000\u0002\u0000\u0000\u0000\u0000\u0001\u0000\u0001\u0000\u0006ÿÿÿÿ\u0000\u0000\u0000\u0000\u0000\u0000\u0000\u0000\u0000\u0000\u0000\u0000õæî¯ÄÔºMÚ\u0003\u001e\u001fY.á\u0000\u0000\u0000\n\u0000\u0000\u0000\u0010\u0000\u0000\u0000\u0000<dºômÂH\u0011|Ø-P\t*Ô\u001dÙ\u0000²\u0004é\tìøB~\u0000\u0000@\u0000\u0000\u0000\u0000\u0000\u0000\u0000\u0000\u0010\u0000\u0000\u0000\u0000\u0000\u0000\u0000\u0000\u0000\u0000\u0000\u0000\u0000\u0000\u0000\u0000\u0000\u0000\u0000&\u0000\u0001LVCC\u0016System Load Button.ctl\u0000\u0000\u0000\u0000\u0000\u0000\u0000\u0000\u0003\u0000\u0000\u0000\u0000\u0000\u0002\u0000\u0001\u0000\u0000\u0000\u0000\u0000\u0014\u0000\b\u0000\u0002\u0010\u0000\u0010\u0001\u0010\u0000\u0010\u0004\u0010\u00000\u0000\u0010\b\u0010\u0000\u0000\u0000\u0000A\u0000\u0000\u0001\u0011xc`À\u0004ÿ\u0000H12007\u0000iVtñÿPE+Å\u0000Ù\\lv\u0010i/#P\u0011Ó\u0007 \u0001ì\u0011\u0010fú\u0003ÄÿPTaÑ\t\u0000´Ò e\u0000\u0000\u0000\u0000\u0000\u0000&\u0000\u0001VIDS\u0016System Load Button.ctl\u0000\u0000\u0000\u0000\u0000\u0000\u0000\u0000\u0003\u0000\u0000\u0000\u0000\u0000\u0000\u0000\u0000Ôxg``È4¶0Æ\u0000Éù)© ú\u0000\u0010¿f=<!´;G#80(,¼»DE¥»FE\u001f\u001bÿ>y\u001b;\u0018\nKXwô²yX42ìÐ\u0002ÊtºiìP\u0002Ó\u000e;âÁ´Kè\u000bÎÞ\u0014\u0015\u0016¶6 ÿ Ð\u001cQÿ\u0000$ÏÈÀÌËPÊPË\fý]\\ù 7\u0003\u0000Â\u000308\u0000\u0000\u0000\u0000\u0000\u0000\r\t\u0001\u0011\u0000\u0000\u00059.0.1\u0000\u0000\u0000\u0000\u0000\u0000\u0000\u0000\u0000\u0000\u0000\u0000\u0000\u0000\u0000\u000fÿÿÿ\u0000\u0000\u0000\u0000 \u0000\u0000\u0000 \u0000\u0000\u0000 \u0000\u0000\u0000 \u0000\u0000\u0000 \u0004\u0000\u0000 \u0004\u0000\u0000 \u0004\u0000\u0000 \u0004\u0000\u0000 8\u0012\u0000  \u0002\u0000...", "RSRC\r\n\u0000\u0003LVCCLBVW\u0000\u0000+x\u0000\u0000\u0003Ï\u0000\u0000\u0000 \u0000\u0000+X\u0000\u0000\u0000x\t\u0000\u0000\u0000\u0000\u0000\u0000 \u0000\u0000\u0000\u0000\u0000\u0000\u0004\u0000\u0003\u0000<\u0000¼\u0000\u001f@\u0000\u0002\u0000\u0000\u0000\u0000\u0001\u0000\u0001\u0000\u0006ÿÿÿÿ\u0000\u0000\u0000\u0000\u0000\u0000\u0000\u0000\u0000\u0000\u0000\u0000=âúÑð0Aá\u0007übRÚ\u0000\u0000\u0000\n\u0000\u0000\u0000\u0010\u0000\u0000\u0000\u0000b\u0005\u000bß\nwL6ÙØD?Ô\u001dÙ\u0000²\u0004é\tìøB~\u0000\u0000@\u0000\u0000\u0000\u0000\u0000\u0000\u0000\u0000\u0010\u0000\u0000\u0000\u0000\u0000\u0000\u0000\u0000\u0000\u0000\u0000\u0000\u0000\u0000\u0000\u0000\u0000\u0000\u0000&\u0000\u0001LVCC\u0016System Next Button.ctl\u0000\u0000\u0000\u0000\u0000\u0000\u0000\u0000\u0003\u0000\u0000\u0000\u0000\u0000\u0002\u0000\u0001\u0000\u0000\u0000\u0000\u0000\u0014\u0000\b\u0000\u0002\u0010\u0000\u0010\u0001\u0010\u0000\u0010\u0004\u0010\u00000\u0000\u0010\b\u0010\u0000\u0000\u0000\u0000A\u0000\u0000\u0001\u0011xc`À\u0004ÿ\u0000H12007\u0000iVtñÿPE+Å\u0000Ù\\lv\u0010i/#P\u0011Ó\u0007 \u0001ì\u0011\u0010fú\u0003ÄÿPTaÑ\t\u0000´Ò e\u0000\u0000\u0000\u0000\u0000\u0000&\u0000\u0001VIDS\u0016System Next Button.ctl\u0000\u0000\u0000\u0000\u0000\u0000\u0000\u0000\u0003\u0000\u0000\u0000\u0000\u0000\u0000\u0000\u0000Ôxg``È4¶0Æ\u0000Éù)© ú\u0000\u0010¿f=<!´;G#80(,¼»DE¥»FE\u001f\u001bÿ>y\u001b;\u0018\nKXwô²yX42ìÐ\u0002ÊtºiìP\u0002Ó\u000e;âÁ´Kè\u000bÎÞ\u0014\u0015\u0016¶6 ÿ Ð\u001cQÿ\u0000$ÏÈÀÌËPÊPË\fý]\\ù 7\u0003\u0000Â\u000308\u0000\u0000\u0000\u0000\u0000\u0000\r\t\u0001\u0011\u0000\u0000\u00059.0.1\u0000\u0000\u0000\u0000\u0000\u0000\u0000\u0000\u0000\u0000\u0000\u0000\u0000\u0000\u0000\u000fÿÿÿ\u0000\u0000\u0000\u0000 \u0000\u0000\u0000 \u0001\u0000\u0000 \u0001À\u0000 \u0001`\u0000 0\u0000 @Ø\u0000 _ì\u0000 _þ\u0000 ü\u0000 ø\u0000...", "RSRC\r\n\u0000\u0003LVCCLBVW\u0000\u00000\u0018\u0000\u0000\u0003Í\u0000\u0000\u0000 \u0000\u0000/ø\u0000\u0000\u0000x\t\u0000\u0000\u0000\u0000\u0000\u0000 \u0000\u0000\u0000\u0000\u0000\u0000\u0004\u0000\u0003\u0000<\u0000¼\u0000\u001f@\u0000\u0002\u0000\u0000\u0000\u0000\u0001\u0000\u0001\u0000\u0006ÿÿÿÿ\u0000\u0000\u0000\u0000\u0000\u0000\u0000\u0000\u0000\u0000\u0000\u0000\u000e#5»ã}L\"ÒÿÊ\u0000\u0000\u0000\n\u0000\u0000\u0000\u0010\u0000\u0000\u0000\u0000®\u001e\nÜ\u0006ºÔN¥Â]»ÎuÏóÔ\u001dÙ\u0000²\u0004é\tìøB~\u0000\u0000@\u0000\u0000\u0000\u0000\u0000\u0000\u0000\u0000\u0010\u0000\u0000\u0000\u0000\u0000\u0000\u0000\u0000\u0000\u0000\u0000\u0000\u0000\u0000\u0000\u0000\u0000\u0000\u0000$\u0000\u0001LVCC\u0014System OK Button.ctl\u0000\u0000\u0000\u0000\u0000\u0000\u0000\u0000\u0003\u0000\u0000\u0000\u0002\u0000\u0001\u0000\u0000\u0000\u0000\u0000\u0014\u0000\b\u0000\u0002\u0010\u0000\u0010\u0001\u0010\u0000\u0010\u0004\u0010\u00000\u0000\u0010\b\u0010\u0000\u0000\u0000\u0000A\u0000\u0000\u0001\u0011xc`À\u0004ÿ\u0000H12007\u0000iVtñÿPE+Å\u0000Ù\\lv\u0010i/#P\u0011Ó\u0007 \u0001ì\u0011\u0010fú\u0003ÄÿPTaÑ\t\u0000´Ò e\u0000\u0000\u0000\u0000\u0000\u0000$\u0000\u0001VIDS\u0014System OK Button.ctl\u0000\u0000\u0000\u0000\u0000\u0000\u0000\u0000\u0003\u0000\u0000\u0000\u0000\u0000\u0000Ôxg``È4¶0Æ\u0000Éù)© ú\u0000\u0010¿f=<!´;G#80(,¼»DE¥»FE\u001f\u001bÿ>y\u001b;\u0018\nKXwô²yX42ìÐ\u0002ÊtºiìP\u0002Ó\u000e;âÁ´Kè\u000bÎÞ\u0014\u0015\u0016¶6 ÿ Ð\u001cQÿ\u0000$ÏÈÀÌËPÊPË\fý]\\ù 7\u0003\u0000Â\u000308\u0000\u0000\u0000\u0000\u0000\u0000\r\t\u0001\u0011\u0000\u0000\u00059.0.1\u0000\u0000\u0000\u0000\u0000\u0000\u0000\u0000\u0000\u0000\u0000\u0000\u0000\u0000\u0000\u000fÿÿÿ\u0000\u0000\u0000\u0000 \u0000\u0000\u0000 \u0000\u0000\u0000 \u0000\u0000\u0000 \u0000\u0000\u0000 \u0000\u000e\u0000 \u0000\u000e\u0000 \u0000\u001c\u0000 \u00008\u0000 \u00000\u0000   \u0000 \u0010\u0000\u0000 \u0000\u0000\u0000...", "RSRC\r\n\u0000\u0003LVCCLBVW\u0000\u00005\u0000\u0000\u0003Ï\u0000\u0000\u0000 \u0000\u00005l\u0000\u0000\u0000x\t\u0000\u0000\u0000\u0000\u0000\u0000 \u0000\u0000\u0000\u0000\u0000\u0000\u0004\u0000\u0003\u0000<\u0000¼\u0000\u001f@\u0000\u0002\u0000\u0000\u0000\u0000\u0001\u0000\u0001\u0000\u0006ÿÿÿÿ\u0000\u0000\u0000\u0000\u0000\u0000\u0000\u0000\u0000\u0000\u0000\u0000¬\u0018\u0004$.@®ÃÈ\u0011\u000b_\fÒ\u0000\u0000\u0000\n\u0000\u0000\u0000\u0010\u0000\u0000\u0000\u0000)óá0C»¦ãKÔ\u001dÙ\u0000²\u0004é\tìøB~\u0000\u0000@\u0000\u0000\u0000\u0000\u0000\u0000\u0000\u0000\u0010\u0000\u0000\u0000\u0000\u0000\u0000\u0000\u0000\u0000\u0000\u0000\u0000\u0000\u0000\u0000\u0000\u0000\u0000\u0000&\u0000\u0001LVCC\u0016System Open Button.ctl\u0000\u0000\u0000\u0000\u0000\u0000\u0000\u0000\u0003\u0000\u0000\u0000\u0000\u0000\u0002\u0000\u0001\u0000\u0000\u0000\u0000\u0000\u0014\u0000\b\u0000\u0002\u0010\u0000\u0010\u0001\u0010\u0000\u0010\u0004\u0010\u00000\u0000\u0010\b\u0010\u0000\u0000\u0000\u0000A\u0000\u0000\u0001\u0011xc`À\u0004ÿ\u0000H12007\u0000iVtñÿPE+Å\u0000Ù\\lv\u0010i/#P\u0011Ó\u0007 \u0001ì\u0011\u0010fú\u0003ÄÿPTaÑ\t\u0000´Ò e\u0000\u0000\u0000\u0000\u0000\u0000&\u0000\u0001VIDS\u0016System Open Button.ctl\u0000\u0000\u0000\u0000\u0000\u0000\u0000\u0000\u0003\u0000\u0000\u0000\u0000\u0000\u0000\u0000\u0000Ôxg``È4¶0Æ\u0000Éù)© ú\u0000\u0010¿f=<!´;G#80(,¼»DE¥»FE\u001f\u001bÿ>y\u001b;\u0018\nKXwô²yX42ìÐ\u0002ÊtºiìP\u0002Ó\u000e;âÁ´Kè\u000bÎÞ\u0014\u0015\u0016¶6 ÿ Ð\u001cQÿ\u0000$ÏÈÀÌËPÊPË\fý]\\ù 7\u0003\u0000Â\u000308\u0000\u0000\u0000\u0000\u0000\u0000\r\t\u0001\u0011\u0000\u0000\u00059.0.1\u0000\u0000\u0000\u0000\u0000\u0000\u0000\u0000\u0000\u0000\u0000\u0000\u0000\u0000\u0000\u000fÿÿÿ\u0000\u0000\u0000\u0000 \u0000\u0000\u0000 \u0000\u0000\u0000 \u0000\u0000\u0000 \u0000\u0000\u0000 \u0000\u0000\u0000 \u0000\u0000\u0000 \u0000\u0000\u0000 \u0000\u0000\u0000 \u0000\u0000\u0000 \u0000\u0000\u0000...", "RSRC\r\n\u0000\u0003LVCCLBVW\u0000\u0000($\u0000\u0000\u0003Ð\u0000\u0000\u0000 \u0000\u0000(\u0004\u0000\u0000\u0000x\t\u0000\u0000\u0000\u0000\u0000\u0000 \u0000\u0000\u0000\u0000\u0000\u0000\u0004\u0000\u0003\u0000<\u0000¼\u0000\u001f@\u0000\u0002\u0000\u0000\u0000\u0000\u0001\u0000\u0001\u0000\u0006ÿÿÿÿ\u0000\u0000\u0000\u0000\u0000\u0000\u0000\u0000\u0000\u0000\u0000\u0000|-oÑYTJ ásúX¤h\u0001\u0000\u0000\u0000\n\u0000\u0000\u0000\u0010\u0000\u0000\u0000\u0000H\u0015ªá4óTN¯Rá¨÷¯b4Ô\u001dÙ\u0000²\u0004é\tìøB~\u0000\u0000@\u0000\u0000\u0000\u0000\u0000\u0000\u0000\u0000\u0010\u0000\u0000\u0000\u0000\u0000\u0000\u0000\u0000\u0000\u0000\u0000\u0000\u0000\u0000\u0000\u0000\u0000\u0000\u0000&\u0000\u0001LVCC\u0017System Pause Button.ctl\u0000\u0000\u0000\u0000\u0000\u0000\u0000\u0003\u0000\u0000\u0000\u0000\u0000\u0002\u0000\u0001\u0000\u0000\u0000\u0000\u0000\u0014\u0000\b\u0000\u0002\u0010\u0000\u0010\u0001\u0010\u0000\u0010\u0004\u0010\u00000\u0000\u0010\b\u0010\u0000\u0000\u0000\u0000A\u0000\u0000\u0001\u0011xc`À\u0004ÿ\u0000H12007\u0000iVtñÿPE+Å\u0000Ù\\lv\u0010i/#P\u0011Ó\u0007 \u0001ì\u0011\u0010fú\u0003ÄÿPTaÑ\t\u0000´Ò e\u0000\u0000\u0000\u0000\u0000\u0000&\u0000\u0001VIDS\u0017System Pause Button.ctl\u0000\u0000\u0000\u0000\u0000\u0000\u0000\u0003\u0000\u0000\u0000\u0000\u0000\u0000\u0000\u0000Ôxg``È4¶0Æ\u0000Éù)© ú\u0000\u0010¿f=<!´;G#80(,¼»DE¥»FE\u001f\u001bÿ>y\u001b;\u0018\nKXwô²yX42ìÐ\u0002ÊtºiìP\u0002Ó\u000e;âÁ´Kè\u000bÎÞ\u0014\u0015\u0016¶6 ÿ Ð\u001cQÿ\u0000$ÏÈÀÌËPÊPË\fý]\\ù 7\u0003\u0000Â\u000308\u0000\u0000\u0000\u0000\u0000\u0000\r\t\u0001\u0011\u0000\u0000\u00059.0.1\u0000\u0000\u0000\u0000\u0000\u0000\u0000\u0000\u0000\u0000\u0000\u0000\u0000\u0000\u0000\u0000\u0000\u0000\u0000\u0007ÿÿÿ\u0000\u0000\u0000\u0000\u0010~\u000f\u0010B\u0010\u0010B\u0010\u0010B\u0010\u0010B\u0018\u0010F\u0018\u0010V\u001a\u0010F\u0018\u0010F\u0018...", "RSRC\r\n\u0000\u0003LVCCLBVW\u0000\u0000,\u0000\u0000\u0003Ð\u0000\u0000\u0000 \u0000\u0000,x\u0000\u0000\u0000x\t\u0000\u0000\u0000\u0000\u0000\u0000 \u0000\u0000\u0000\u0000\u0000\u0000\u0004\u0000\u0003\u0000<\u0000¼\u0000\u001f@\u0000\u0002\u0000\u0000\u0000\u0000\u0001\u0000\u0001\u0000\u0006ÿÿÿÿ\u0000\u0000\u0000\u0000\u0000\u0000\u0000\u0000\u0000\u0000\u0000\u0000ë¼M\u0003ÓgK³U\u0017¹\u000e0Ì{\u0000\u0000\u0000\n\u0000\u0000\u0000\u0010\u0000\u0000\u0000\u0000\u0004\u0005jÇV\u0005FE¸ÇTñºäÔ\u001dÙ\u0000²\u0004é\tìøB~\u0000\u0000@\u0000\u0000\u0000\u0000\u0000\u0000\u0000\u0000\u0010\u0000\u0000\u0000\u0000\u0000\u0000\u0000\u0000\u0000\u0000\u0000\u0000\u0000\u0000\u0000\u0000\u0000\u0000\u0000&\u0000\u0001LVCC\u0017System Print Button.ctl\u0000\u0000\u0000\u0000\u0000\u0000\u0000\u0003\u0000\u0000\u0000\u0000\u0000\u0002\u0000\u0001\u0000\u0000\u0000\u0000\u0000\u0014\u0000\b\u0000\u0002\u0010\u0000\u0010\u0001\u0010\u0000\u0010\u0004\u0010\u00000\u0000\u0010\b\u0010\u0000\u0000\u0000\u0000A\u0000\u0000\u0001\u0011xc`À\u0004ÿ\u0000H12007\u0000iVtñÿPE+Å\u0000Ù\\lv\u0010i/#P\u0011Ó\u0007 \u0001ì\u0011\u0010fú\u0003ÄÿPTaÑ\t\u0000´Ò e\u0000\u0000\u0000\u0000\u0000\u0000&\u0000\u0001VIDS\u0017System Print Button.ctl\u0000\u0000\u0000\u0000\u0000\u0000\u0000\u0003\u0000\u0000\u0000\u0000\u0000\u0000\u0000\u0000Ôxg``È4¶0Æ\u0000Éù)© ú\u0000\u0010¿f=<!´;G#80(,¼»DE¥»FE\u001f\u001bÿ>y\u001b;\u0018\nKXwô²yX42ìÐ\u0002ÊtºiìP\u0002Ó\u000e;âÁ´Kè\u000bÎÞ\u0014\u0015\u0016¶6 ÿ Ð\u001cQÿ\u0000$ÏÈÀÌËPÊPË\fý]\\ù 7\u0003\u0000Â\u000308\u0000\u0000\u0000\u0000\u0000\u0000\r\t\u0001\u0011\u0000\u0000\u00059.0.1\u0000\u0000\u0000\u0000\u0000\u0000\u0000\u0000\u0000\u0000\u0000\u0000\u0000\u0000\u0000\u000fÿÿÿ\u0000\u0000\u0000\u0000 \u0000\u0000\u0000 \u0000\u0000\u0000 \u0000\u0000\u0000 \u0000\u0000\u0000 \u0000\u0000\u0000 \u0010\u0000\u0000 \u0000\u0000\u0000 \u0010\b\u0000 \u0010\b\u0000 ù\u0000...", "RSRC\r\n\u0000\u0003LVCCLBVW\u0000\u00007Ü\u0000\u0000\u0003Ò\u0000\u0000\u0000 \u0000\u00007¼\u0000\u0000\u0000x\t\u0000\u0000\u0000\u0000\u0000\u0000 \u0000\u0000\u0000\u0000\u0000\u0000\u0004\u0000\u0003\u0000<\u0000¼\u0000\u001f@\u0000\u0002\u0000\u0000\u0000\u0000\u0001\u0000\u0001\u0000\u0006ÿÿÿÿ\u0000\u0000\u0000\u0000\u0000\u0000\u0000\u0000\u0000\u0000\u0000\u0000.&®ä¡¸ÅH« ±×Çí×\u0000\u0000\u0000\n\u0000\u0000\u0000\u0010\u0000\u0000\u0000\u00002\bR»EBº?$jZÑ 'Ô\u001dÙ\u0000²\u0004é\tìøB~\u0000\u0000@\u0000\u0000\u0000\u0000\u0000\u0000\u0000\u0000\u0010\u0000\u0000\u0000\u0000\u0000\u0000\u0000\u0000\u0000\u0000\u0000\u0000\u0000\u0000\u0000\u0000\u0000\u0000\u0000(\u0000\u0001LVCC\u0019System Refresh Button.ctl\u0000\u0000\u0000\u0000\u0000\u0000\u0000\u0003\u0000\u0000\u0000\u0002\u0000\u0001\u0000\u0000\u0000\u0000\u0000\u0014\u0000\b\u0000\u0002\u0010\u0000\u0010\u0001\u0010\u0000\u0010\u0004\u0010\u00000\u0000\u0010\b\u0010\u0000\u0000\u0000\u0000A\u0000\u0000\u0001\u0011xc`À\u0004ÿ\u0000H12007\u0000iVtñÿPE+Å\u0000Ù\\lv\u0010i/#P\u0011Ó\u0007 \u0001ì\u0011\u0010fú\u0003ÄÿPTaÑ\t\u0000´Ò e\u0000\u0000\u0000\u0000\u0000\u0000(\u0000\u0001VIDS\u0019System Refresh Button.ctl\u0000\u0000\u0000\u0000\u0000\u0000\u0000\u0003\u0000\u0000\u0000\u0000\u0000\u0000Ôxg``È4¶0Æ\u0000Éù)© ú\u0000\u0010¿f=<!´;G#80(,¼»DE¥»FE\u001f\u001bÿ>y\u001b;\u0018\nKXwô²yX42ìÐ\u0002ÊtºiìP\u0002Ó\u000e;âÁ´Kè\u000bÎÞ\u0014\u0015\u0016¶6 ÿ Ð\u001cQÿ\u0000$ÏÈÀÌËPÊPË\fý]\\ù 7\u0003\u0000Â\u000308\u0000\u0000\u0000\u0000\u0000\u0000\r\t\u0001\u0011\u0000\u0000\u00059.0.1\u0000\u0000\u0000\u0000\u0000\u0000\u0000\u0000\u0000\u0000\u0000\u0000\u0000\u0000\u0000\u000fÿÿÿ\u0000\u0000\u0000\u0000 \u0000\u0000\u0000 \u0000\u0000\u0000 \u0003\u0000 \u0000\u0010\u0000 \u0000\u0010\u000f \u0003à\b \b@\b p\u0000\b \u0000\u000f\u000f \u0000\u0011\t...", "RSRC\r\n\u0000\u0003LVCCLBVW\u0000\u00003¤\u0000\u0000\u0003Ï\u0000\u0000\u0000 \u0000\u00003\u0000\u0000\u0000x\t\u0000\u0000\u0000\u0000\u0000\u0000 \u0000\u0000\u0000\u0000\u0000\u0000\u0004\u0000\u0003\u0000<\u0000¼\u0000\u001f@\u0000\u0002\u0000\u0000\u0000\u0000\u0001\u0000\u0001\u0000\u0006ÿÿÿÿ\u0000\u0000\u0000\u0000\u0000\u0000\u0000\u0000\u0000\u0000\u0000\u0000\u001e%\bVà3Jë²\u0001÷bÕ°\u0000\u0000\u0000\n\u0000\u0000\u0000\u0010\u0000\u0000\u0000\u0000.í#\u0003qK\"¤Ï\u001dtzÔ\u001dÙ\u0000²\u0004é\tìøB~\u0000\u0000@\u0000\u0000\u0000\u0000\u0000\u0000\u0000\u0000\u0010\u0000\u0000\u0000\u0000\u0000\u0000\u0000\u0000\u0000\u0000\u0000\u0000\u0000\u0000\u0000\u0000\u0000\u0000\u0000&\u0000\u0001LVCC\u0016System Save Button.ctl\u0000\u0000\u0000\u0000\u0000\u0000\u0000\u0000\u0003\u0000\u0000\u0000\u0000\u0000\u0002\u0000\u0001\u0000\u0000\u0000\u0000\u0000\u0014\u0000\b\u0000\u0002\u0010\u0000\u0010\u0001\u0010\u0000\u0010\u0004\u0010\u00000\u0000\u0010\b\u0010\u0000\u0000\u0000\u0000A\u0000\u0000\u0001\u0011xc`À\u0004ÿ\u0000H12007\u0000iVtñÿPE+Å\u0000Ù\\lv\u0010i/#P\u0011Ó\u0007 \u0001ì\u0011\u0010fú\u0003ÄÿPTaÑ\t\u0000´Ò e\u0000\u0000\u0000\u0000\u0000\u0000&\u0000\u0001VIDS\u0016System Save Button.ctl\u0000\u0000\u0000\u0000\u0000\u0000\u0000\u0000\u0003\u0000\u0000\u0000\u0000\u0000\u0000\u0000\u0000Ôxg``È4¶0Æ\u0000Éù)© ú\u0000\u0010¿f=<!´;G#80(,¼»DE¥»FE\u001f\u001bÿ>y\u001b;\u0018\nKXwô²yX42ìÐ\u0002ÊtºiìP\u0002Ó\u000e;âÁ´Kè\u000bÎÞ\u0014\u0015\u0016¶6 ÿ Ð\u001cQÿ\u0000$ÏÈÀÌËPÊPË\fý]\\ù 7\u0003\u0000Â\u000308\u0000\u0000\u0000\u0000\u0000\u0000\r\t\u0001\u0011\u0000\u0000\u00059.0.1\u0000\u0000\u0000\u0000\u0000\u0000\u0000\u0000\u0000\u0000\u0000\u0000\u0000\u0000\u0000\u000fÿÿÿ\u0000\u0000\u0000\u0000 \u0000\u0000\u0000 `\u0006\u0000 `\u0006\u0000 `\u0006\u0000 `\u0006\u0000 `\u0006\u0000 `\u0006\u0000 `\u0006\u0000 þ\u0000 þ\u0000...", "RSRC\r\n\u0000\u0003LVCCLBVW\u0000\u00008\u0000\u0000\u0003Ô\u0000\u0000\u0000 \u0000\u00008p\u0000\u0000\u0000x\t\u0000\u0000\u0000\u0000\u0000\u0000 \u0000\u0000\u0000\u0000\u0000\u0000\u0004\u0000\u0003\u0000<\u0000¼\u0000\u001f@\u0000\u0002\u0000\u0000\u0000\u0000\u0001\u0000\u0001\u0000\u0006ÿÿÿÿ\u0000\u0000\u0000\u0000\u0000\u0000\u0000\u0000\u0000\u0000\u0000\u0000Û¢ÐôXÐéDÑß_pº\u0000\u0000\u0000\n\u0000\u0000\u0000\u0010\u0000\u0000\u0000\u0000ýæ;ÙÜoH|TvÚÌB½Ô\u001dÙ\u0000²\u0004é\tìøB~\u0000\u0000@\u0000\u0000\u0000\u0000\u0000\u0000\u0000\u0000\u0010\u0000\u0000\u0000\u0000\u0000\u0000\u0000\u0000\u0000\u0000\u0000\u0000\u0000\u0000\u0000\u0000\u0000\u0000\u0000*\u0000\u0001LVCC\u001bSystem Save Data Button.ctl\u0000\u0000\u0000\u0000\u0000\u0000\u0000\u0003\u0000\u0000\u0000\u0000\u0000\u0002\u0000\u0001\u0000\u0000\u0000\u0000\u0000\u0014\u0000\b\u0000\u0002\u0010\u0000\u0010\u0001\u0010\u0000\u0010\u0004\u0010\u00000\u0000\u0010\b\u0010\u0000\u0000\u0000\u0000A\u0000\u0000\u0001\u0011xc`À\u0004ÿ\u0000H12007\u0000iVtñÿPE+Å\u0000Ù\\lv\u0010i/#P\u0011Ó\u0007 \u0001ì\u0011\u0010fú\u0003ÄÿPTaÑ\t\u0000´Ò e\u0000\u0000\u0000\u0000\u0000\u0000*\u0000\u0001VIDS\u001bSystem Save Data Button.ctl\u0000\u0000\u0000\u0000\u0000\u0000\u0000\u0003\u0000\u0000\u0000\u0000\u0000\u0000\u0000\u0000Ôxg``È4¶0Æ\u0000Éù)© ú\u0000\u0010¿f=<!´;G#80(,¼»DE¥»FE\u001f\u001bÿ>y\u001b;\u0018\nKXwô²yX42ìÐ\u0002ÊtºiìP\u0002Ó\u000e;âÁ´Kè\u000bÎÞ\u0014\u0015\u0016¶6 ÿ Ð\u001cQÿ\u0000$ÏÈÀÌËPÊPË\fý]\\ù 7\u0003\u0000Â\u000308\u0000\u0000\u0000\u0000\u0000\u0000\r\t\u0001\u0011\u0000\u0000\u00059.0.1\u0000\u0000\u0000\u0000\u0000\u0000\u0000\u0000\u0000\u0000\u0000\u0000\u0000\u0000\u0000\u000fÿÿÿ\u0000\u0000\u0000\u0000 \u0000\u0000\u0000 \u0000\u0000\u0000 \u0000\u0000\u0000 \u0000\u0000\u0000 \u0000\u0000\u0000 \u0000\u0000\u0000 \u0000\u0000\u0000 \u0000\u0000\u0000...", "RSRC\r\n\u0000\u0003LVCCLBVW\u0000\u00007<\u0000\u0000\u0003Ó\u0000\u0000\u0000 \u0000\u00007\u001c\u0000\u0000\u0000x\t\u0000\u0000\u0000\u0000\u0000\u0000 \u0000\u0000\u0000\u0000\u0000\u0000\u0004\u0000\u0003\u0000<\u0000¼\u0000\u001f@\u0000\u0002\u0000\u0000\u0000\u0000\u0001\u0000\u0001\u0000\u0006ÿÿÿÿ\u0000\u0000\u0000\u0000\u0000\u0000\u0000\u0000\u0000\u0000\u0000\u0000¹r¢ÝaK¡{f@~\u001c¿\u0000\u0000\u0000\n\u0000\u0000\u0000\u0010\u0000\u0000\u0000\u0000cë/Ôä\bÄC¾·A-ïU»ÜÔ\u001dÙ\u0000²\u0004é\tìøB~\u0000\u0000@\u0000\u0000\u0000\u0000\u0000\u0000\u0000\u0000\u0010\u0000\u0000\u0000\u0000\u0000\u0000\u0000\u0000\u0000\u0000\u0000\u0000\u0000\u0000\u0000\u0000\u0000\u0000\u0000*\u0000\u0001LVCC\u001aSystem Settings Button.ctl\u0000\u0000\u0000\u0000\u0000\u0000\u0000\u0000\u0003\u0000\u0000\u0000\u0000\u0000\u0002\u0000\u0001\u0000\u0000\u0000\u0000\u0000\u0014\u0000\b\u0000\u0002\u0010\u0000\u0010\u0001\u0010\u0000\u0010\u0004\u0010\u00000\u0000\u0010\b\u0010\u0000\u0000\u0000\u0000A\u0000\u0000\u0001\u0011xc`À\u0004ÿ\u0000H12007\u0000iVtñÿPE+Å\u0000Ù\\lv\u0010i/#P\u0011Ó\u0007 \u0001ì\u0011\u0010fú\u0003ÄÿPTaÑ\t\u0000´Ò e\u0000\u0000\u0000\u0000\u0000\u0000*\u0000\u0001VIDS\u001aSystem Settings Button.ctl\u0000\u0000\u0000\u0000\u0000\u0000\u0000\u0000\u0003\u0000\u0000\u0000\u0000\u0000\u0000\u0000\u0000Ôxg``È4¶0Æ\u0000Éù)© ú\u0000\u0010¿f=<!´;G#80(,¼»DE¥»FE\u001f\u001bÿ>y\u001b;\u0018\nKXwô²yX42ìÐ\u0002ÊtºiìP\u0002Ó\u000e;âÁ´Kè\u000bÎÞ\u0014\u0015\u0016¶6 ÿ Ð\u001cQÿ\u0000$ÏÈÀÌËPÊPË\fý]\\ù 7\u0003\u0000Â\u000308\u0000\u0000\u0000\u0000\u0000\u0000\r\t\u0001\u0011\u0000\u0000\u00059.0.1\u0000\u0000\u0000\u0000\u0000\u0000\u0000\u0000\u0000\u0000\u0000\u0000\u0000\u0000\u0000\u000fÿÿÿ\u0000\u0000\u0000\u0000 \u0000\u0000\u0000 \u0000\u0000\u0000 \u0000\u0000\u0000 \u0000\u0000\u0000 \u0000\u0000\u000e @\u0000\u0010 \u0000\u0000\u0010 \u0000@\u0018...", "RSRC\r\n\u0000\u0003LVCCLBVW\u0000\u00004H\u0000\u0000\u0003Ð\u0000\u0000\u0000 \u0000\u00004(\u0000\u0000\u0000x\t\u0000\u0000\u0000\u0000\u0000\u0000 \u0000\u0000\u0000\u0000\u0000\u0000\u0004\u0000\u0003\u0000<\u0000¼\u0000\u001f@\u0000\u0002\u0000\u0000\u0000\u0000\u0001\u0000\u0001\u0000\u0006ÿÿÿÿ\u0000\u0000\u0000\u0000\u0000\u0000\u0000\u0000\u0000\u0000\u0000\u0000«¹pFÔIß|ã\u001a´\u0000\u0000\u0000\n\u0000\u0000\u0000\u0010\u0000\u0000\u0000\u0000x¶Ný\u0015F¹>}ÏÐ\u000bÔ\u001dÙ\u0000²\u0004é\tìøB~\u0000\u0000@\u0000\u0000\u0000\u0000\u0000\u0000\u0000\u0000\u0010\u0000\u0000\u0000\u0000\u0000\u0000\u0000\u0000\u0000\u0000\u0000\u0000\u0000\u0000\u0000\u0000\u0000\u0000\u0000&\u0000\u0001LVCC\u0017System Start Button.ctl\u0000\u0000\u0000\u0000\u0000\u0000\u0000\u0003\u0000\u0000\u0000\u0000\u0000\u0002\u0000\u0001\u0000\u0000\u0000\u0000\u0000\u0014\u0000\b\u0000\u0002\u0010\u0000\u0010\u0001\u0010\u0000\u0010\u0004\u0010\u00000\u0000\u0010\b\u0010\u0000\u0000\u0000\u0000A\u0000\u0000\u0001\u0011xc`À\u0004ÿ\u0000H12007\u0000iVtñÿPE+Å\u0000Ù\\lv\u0010i/#P\u0011Ó\u0007 \u0001ì\u0011\u0010fú\u0003ÄÿPTaÑ\t\u0000´Ò e\u0000\u0000\u0000\u0000\u0000\u0000&\u0000\u0001VIDS\u0017System Start Button.ctl\u0000\u0000\u0000\u0000\u0000\u0000\u0000\u0003\u0000\u0000\u0000\u0000\u0000\u0000\u0000\u0000Ôxg``È4¶0Æ\u0000Éù)© ú\u0000\u0010¿f=<!´;G#80(,¼»DE¥»FE\u001f\u001bÿ>y\u001b;\u0018\nKXwô²yX42ìÐ\u0002ÊtºiìP\u0002Ó\u000e;âÁ´Kè\u000bÎÞ\u0014\u0015\u0016¶6 ÿ Ð\u001cQÿ\u0000$ÏÈÀÌËPÊPË\fý]\\ù 7\u0003\u0000Â\u000308\u0000\u0000\u0000\u0000\u0000\u0000\r\t\u0001\u0011\u0000\u0000\u00059.0.1\u0000\u0000\u0000\u0000\u0000\u0000\u0000\u0000\u0000\u0000\u0000\u0000\u0000\u0000\u0000\u000fÿÿÿ\u0000\u0000\u0000\u0000 À\u0000\u0000 \u0000\u0000 \u0000\u0000 \u0000\u0000 À\u0000 0\u0000 \f\u0000 ¿ç\u0000 ¿ç\u0000 \u001c\u0000...", "RSRC\r\n\u0000\u0003LVCCLBVW\u0000\u00000\u001c\u0000\u0000\u0003Ï\u0000\u0000\u0000 \u0000\u0000/ü\u0000\u0000\u0000x\t\u0000\u0000\u0000\u0000\u0000\u0000 \u0000\u0000\u0000\u0000\u0000\u0000\u0004\u0000\u0003\u0000<\u0000¼\u0000\u001f@\u0000\u0002\u0000\u0000\u0000\u0000\u0001\u0000\u0001\u0000\u0006ÿÿÿÿ\u0000\u0000\u0000\u0000\u0000\u0000\u0000\u0000\u0000\u0000\u0000\u00000×\u0006aáJ° 5Y «\u0000\u0000\u0000\n\u0000\u0000\u0000\u0010\u0000\u0000\u0000\u0000ÐÏ×;¶æ\u0018E\u0015ý\u001añ\r:|Ô\u001dÙ\u0000²\u0004é\tìøB~\u0000\u0000@\u0000\u0000\u0000\u0000\u0000\u0000\u0000\u0000\u0010\u0000\u0000\u0000\u0000\u0000\u0000\u0000\u0000\u0000\u0000\u0000\u0000\u0000\u0000\u0000\u0000\u0000\u0000\u0000&\u0000\u0001LVCC\u0016System Stop Button.ctl\u0000\u0000\u0000\u0000\u0000\u0000\u0000\u0000\u0003\u0000\u0000\u0000\u0000\u0000\u0002\u0000\u0001\u0000\u0000\u0000\u0000\u0000\u0014\u0000\b\u0000\u0002\u0010\u0000\u0010\u0001\u0010\u0000\u0010\u0004\u0010\u00000\u0000\u0010\b\u0010\u0000\u0000\u0000\u0000A\u0000\u0000\u0001\u0011xc`À\u0004ÿ\u0000H12007\u0000iVtñÿPE+Å\u0000Ù\\lv\u0010i/#P\u0011Ó\u0007 \u0001ì\u0011\u0010fú\u0003ÄÿPTaÑ\t\u0000´Ò e\u0000\u0000\u0000\u0000\u0000\u0000&\u0000\u0001VIDS\u0016System Stop Button.ctl\u0000\u0000\u0000\u0000\u0000\u0000\u0000\u0000\u0003\u0000\u0000\u0000\u0000\u0000\u0000\u0000\u0000Ôxg``È4¶0Æ\u0000Éù)© ú\u0000\u0010¿f=<!´;G#80(,¼»DE¥»FE\u001f\u001bÿ>y\u001b;\u0018\nKXwô²yX42ìÐ\u0002ÊtºiìP\u0002Ó\u000e;âÁ´Kè\u000bÎÞ\u0014\u0015\u0016¶6 ÿ Ð\u001cQÿ\u0000$ÏÈÀÌËPÊPË\fý]\\ù 7\u0003\u0000Â\u000308\u0000\u0000\u0000\u0000\u0000\u0000\r\t\u0001\u0011\u0000\u0000\u00059.0.1\u0000\u0000\u0000\u0000\u0000\u0000\u0000\u0000\u0000\u0000\u0000\u0000\u0000\u0000\u0000\u000fÿÿÿ\u0000\u0000\u0000\u0000 \u0000\u0000\u0000 \u0006 \u0000 \b\u0010\u0000 \u0010\b\u0000  \u0004\u0000 @\u0002\u0000 @\u0002\u0000 @\u0002\u0000 x>\u0000 x\u001e\u0000...", "RSRC\r\n\u0000\u0003LVCCLBVW\u0000\u0000Nä\u0000\u0000\u0003ä\u0000\u0000\u0000 \u0000\u0000NÄ\u0000\u0000\u0000x\t\u0000\u0000\u0000\u0000\u0000\u0000 \u0000\u0000\u0000\u0000\u0000\u0000\u0004\u0000\u0003\u0000<\u0000¼\u0000\u001f@\u0000\u0002\u0000\u0000\u0000\u0000\u0001\u0000\u0001\u0000\u0006ÿÿÿÿ\u0000\u0000\u0000\u0000\u0000\u0000\u0000\u0000\u0000\u0000\u0000\u00001\r\u001aÅÍQ\u000bC¥ÅÓ^9\u0000\u0000\u0000\n\u0000\u0000\u0000\u0010\u0000\u0000\u0000\u0000é°DªrÚG£. xíMNÔ\u001dÙ\u0000²\u0004é\tìøB~\u0000\u0000@\u0000\u0000\u0000\u0000\u0000\u0000\u0000\u0000\u0010\u0000\u0000\u0000\u0000\u0000\u0000\u0000\u0000\u0000\u0000\u0000\u0000\u0000\u0000\u0000\u0000\u0000\u0000\u0000&\u0000\u0001LVCC\u0017Vertical Add Button.ctl\u0000\u0000\u0000\u0000\u0000\u0000\u0000\u0003\u0000\u0000\u0000\u0000\u0000\u0002\u0000\u0001\u0000\u0000\u0000\u0000\u0000\u0014\u0000\b\u0000\u0002\u0010\u0000\u0010\u0001\u0010\u0000\u0010\u0004\u0010\u00000\u0000\u0010\b\u0010\u0000\u0000\u0000\u0000A\u0000\u0000\u0001\u0011xc`À\u0004ÿ\u0000H12007\u0000iVtñÿPE+Å\u0000Ù\\lv\u0010i/#P\u0011Ó\u0007 \u0001ì\u0011\u0010fú\u0003ÄÿPTaÑ\t\u0000´Ò e\u0000\u0000\u0000\u0000\u0000\u0000&\u0000\u0001VIDS\u0017Vertical Add Button.ctl\u0000\u0000\u0000\u0000\u0000\u0000\u0000\u0003\u0000\u0000\u0000\u0000\u0000\u0000\u0000\u0000Ôxg``È4¶0Æ\u0000Éù)© ú\u0000\u0010¿f=<!´;G#80(,¼»DE¥»FE\u001f\u001bÿ>y\u001b;\u0018\nKXwô²yX42ìÐ\u0002ÊtºiìP\u0002Ó\u000e;âÁ´Kè\u000bÎÞ\u0014\u0015\u0016¶6 ÿ Ð\u001cQÿ\u0000$ÏÈÀÌËPÊPË\fý]\\ù 7\u0003\u0000Â\u000308\u0000\u0000\u0000\u0000\u0000\u0000\r\t\u0001\u0011\u0000\u0000\u00059.0.1\u0000\u0000\u0000\u0000\u0000\u0000\u0000\u0000\u0000\u0000\u0000\u0000\u0000\u0000\u0000\u0000\u0000\u0000\u0000\u0000\u0007à\u0000\u0000\b\u0010\u0000\u0000\b\u0010\u0000\u0000\b\u0010\u0000\u0000\b\u0010\u0000\u0000\b\u0010\u0000\u0000\b\u0010\u0000\u0000\b\u0010\u0000\u0000\b\u0010\u0000\u001fø\u001fø\u0010\u0000\u0000\b...", "RSRC\r\n\u0000\u0003LVCCLBVW\u0000\u00001X\u0000\u0000\u0003å\u0000\u0000\u0000 \u0000\u000018\u0000\u0000\u0000x\t\u0000\u0000\u0000\u0000\u0000\u0000 \u0000\u0000\u0000\u0000\u0000\u0000\u0004\u0000\u0003\u0000<\u0000¼\u0000\u001f@\u0000\u0002\u0000\u0000\u0000\u0000\u0001\u0000\u0001\u0000\u0006ÿÿÿÿ\u0000\u0000\u0000\u0000\u0000\u0000\u0000\u0000\u0000\u0000\u0000\u0000©»(´\u0012\u000eB²\\d\u0014À¾\u0000\u0000\u0000\n\u0000\u0000\u0000\u0010\u0000\u0000\u0000\u0000òuÞBEPÔ ç\u001ag=Ô\u001dÙ\u0000²\u0004é\tìøB~\u0000\u0000@\u0000\u0000\u0000\u0000\u0000\u0000\u0000\u0000\u0010\u0000\u0000\u0000\u0000\u0000\u0000\u0000\u0000\u0000\u0000\u0000\u0000\u0000\u0000\u0000\u0000\u0000\u0000\u0000(\u0000\u0001LVCC\u0018Vertical Back Button.ctl\u0000\u0000\u0000\u0000\u0000\u0000\u0000\u0000\u0003\u0000\u0000\u0000\u0002\u0000\u0001\u0000\u0000\u0000\u0000\u0000\u0014\u0000\b\u0000\u0002\u0010\u0000\u0010\u0001\u0010\u0000\u0010\u0004\u0010\u00000\u0000\u0010\b\u0010\u0000\u0000\u0000\u0000A\u0000\u0000\u0001\u0011xc`À\u0004ÿ\u0000H12007\u0000iVtñÿPE+Å\u0000Ù\\lv\u0010i/#P\u0011Ó\u0007 \u0001ì\u0011\u0010fú\u0003ÄÿPTaÑ\t\u0000´Ò e\u0000\u0000\u0000\u0000\u0000\u0000(\u0000\u0001VIDS\u0018Vertical Back Button.ctl\u0000\u0000\u0000\u0000\u0000\u0000\u0000\u0000\u0003\u0000\u0000\u0000\u0000\u0000\u0000Ôxg``È4¶0Æ\u0000Éù)© ú\u0000\u0010¿f=<!´;G#80(,¼»DE¥»FE\u001f\u001bÿ>y\u001b;\u0018\nKXwô²yX42ìÐ\u0002ÊtºiìP\u0002Ó\u000e;âÁ´Kè\u000bÎÞ\u0014\u0015\u0016¶6 ÿ Ð\u001cQÿ\u0000$ÏÈÀÌËPÊPË\fý]\\ù 7\u0003\u0000Â\u000308\u0000\u0000\u0000\u0000\u0000\u0000\r\t\u0001\u0011\u0000\u0000\u00059.0.1\u0000\u0000\u0000\u0000\u0000\u0000\u0000\u0000\u0000\u0000\u0000\u0000\u0000\u0000\u0000\u0000\u0000\u0000\u0000\u0000\u0001\u0000\u0000\u0000\u0003\u0000\u0000\u0000\u0005\u0000\u0000\u0000\t\u0000\u0000\u0000\u0011\u0000\u0000\u0000-\u0000\u0000\u0000]ÿà\u0000¼\u0000 \u0003ÿ \u0006ÿÿ \rÿÿ ...", "RSRC\r\n\u0000\u0003LVCCLBVW\u0000\u0000G\u001c\u0000\u0000\u0003ç\u0000\u0000\u0000 \u0000\u0000Fü\u0000\u0000\u0000x\t\u0000\u0000\u0000\u0000\u0000\u0000 \u0000\u0000\u0000\u0000\u0000\u0000\u0004\u0000\u0003\u0000<\u0000¼\u0000\u001f@\u0000\u0002\u0000\u0000\u0000\u0000\u0001\u0000\u0001\u0000\u0006ÿÿÿÿ\u0000\u0000\u0000\u0000\u0000\u0000\u0000\u0000\u0000\u0000\u0000\u0000¹\u0016$µZM£t;ï\u001c*v\u0000\u0000\u0000\n\u0000\u0000\u0000\u0010\u0000\u0000\u0000\u0000ä4\u000e¢?\u0006E¸aq«\u0014B\u0006Ô\u001dÙ\u0000²\u0004é\tìøB~\u0000\u0000@\u0000\u0000\u0000\u0000\u0000\u0000\u0000\u0000\u0010\u0000\u0000\u0000\u0000\u0000\u0000\u0000\u0000\u0000\u0000\u0000\u0000\u0000\u0000\u0000\u0000\u0000\u0000\u0000*\u0000\u0001LVCC\u001aVertical Cancel Button.ctl\u0000\u0000\u0000\u0000\u0000\u0000\u0000\u0000\u0003\u0000\u0000\u0000\u0000\u0000\u0002\u0000\u0001\u0000\u0000\u0000\u0000\u0000\u0014\u0000\b\u0000\u0002\u0010\u0000\u0010\u0001\u0010\u0000\u0010\u0004\u0010\u00000\u0000\u0010\b\u0010\u0000\u0000\u0000\u0000A\u0000\u0000\u0001\u0011xc`À\u0004ÿ\u0000H12007\u0000iVtñÿPE+Å\u0000Ù\\lv\u0010i/#P\u0011Ó\u0007 \u0001ì\u0011\u0010fú\u0003ÄÿPTaÑ\t\u0000´Ò e\u0000\u0000\u0000\u0000\u0000\u0000*\u0000\u0001VIDS\u001aVertical Cancel Button.ctl\u0000\u0000\u0000\u0000\u0000\u0000\u0000\u0000\u0003\u0000\u0000\u0000\u0000\u0000\u0000\u0000\u0000Ôxg``È4¶0Æ\u0000Éù)© ú\u0000\u0010¿f=<!´;G#80(,¼»DE¥»FE\u001f\u001bÿ>y\u001b;\u0018\nKXwô²yX42ìÐ\u0002ÊtºiìP\u0002Ó\u000e;âÁ´Kè\u000bÎÞ\u0014\u0015\u0016¶6 ÿ Ð\u001cQÿ\u0000$ÏÈÀÌËPÊPË\fý]\\ù 7\u0003\u0000Â\u000308\u0000\u0000\u0000\u0000\u0000\u0000\r\t\u0001\u0011\u0000\u0000\u00059.0.1\u0000\u0000\u0000\u0000\u0000\u0000\u0000\u0000\u0000\u0000\u0000\u0000\u0000\u0000\u0000\u0000\u0000\u0000\u0000\u0000H\u0000H\u0000Ì\u0000Ì\u0001\u0001\u0003\u0003\u0003\u0003\u0006\u0001\u0001\büÌü\u0006ÿký\u0003Ïÿ\u0001ÿÏþ...", "RSRC\r\n\u0000\u0003LVCCLBVW\u0000\u00005\\\u0000\u0000\u0003ç\u0000\u0000\u0000 \u0000\u00005<\u0000\u0000\u0000x\t\u0000\u0000\u0000\u0000\u0000\u0000 \u0000\u0000\u0000\u0000\u0000\u0000\u0004\u0000\u0003\u0000<\u0000¼\u0000\u001f@\u0000\u0002\u0000\u0000\u0000\u0000\u0001\u0000\u0001\u0000\u0006ÿÿÿÿ\u0000\u0000\u0000\u0000\u0000\u0000\u0000\u0000\u0000\u0000\u0000\u0000`F7£b³ÉKü©Tog\rÅ\u0000\u0000\u0000\n\u0000\u0000\u0000\u0010\u0000\u0000\u0000\u0000ÀæÃ B\u001aI½^£y\u001b$sÔ\u001dÙ\u0000²\u0004é\tìøB~\u0000\u0000@\u0000\u0000\u0000\u0000\u0000\u0000\u0000\u0000\u0010\u0000\u0000\u0000\u0000\u0000\u0000\u0000\u0000\u0000\u0000\u0000\u0000\u0000\u0000\u0000\u0000\u0000\u0000\u0000*\u0000\u0001LVCC\u001aVertical Filter Button.ctl\u0000\u0000\u0000\u0000\u0000\u0000\u0000\u0000\u0003\u0000\u0000\u0000\u0000\u0000\u0002\u0000\u0001\u0000\u0000\u0000\u0000\u0000\u0014\u0000\b\u0000\u0002\u0010\u0000\u0010\u0001\u0010\u0000\u0010\u0004\u0010\u00000\u0000\u0010\b\u0010\u0000\u0000\u0000\u0000A\u0000\u0000\u0001\u0011xc`À\u0004ÿ\u0000H12007\u0000iVtñÿPE+Å\u0000Ù\\lv\u0010i/#P\u0011Ó\u0007 \u0001ì\u0011\u0010fú\u0003ÄÿPTaÑ\t\u0000´Ò e\u0000\u0000\u0000\u0000\u0000\u0000*\u0000\u0001VIDS\u001aVertical Filter Button.ctl\u0000\u0000\u0000\u0000\u0000\u0000\u0000\u0000\u0003\u0000\u0000\u0000\u0000\u0000\u0000\u0000\u0000Ôxg``È4¶0Æ\u0000Éù)© ú\u0000\u0010¿f=<!´;G#80(,¼»DE¥»FE\u001f\u001bÿ>y\u001b;\u0018\nKXwô²yX42ìÐ\u0002ÊtºiìP\u0002Ó\u000e;âÁ´Kè\u000bÎÞ\u0014\u0015\u0016¶6 ÿ Ð\u001cQÿ\u0000$ÏÈÀÌËPÊPË\fý]\\ù 7\u0003\u0000Â\u000308\u0000\u0000\u0000\u0000\u0000\u0000\r\t\u0001\u0011\u0000\u0000\u00059.0.1\u0000\u0000\u0000\u0000\u0000\u0000\u0000\u0000\u0000\u0000\u0000\u0000\u0000\u0000\u0000\u0000\u0000\u0000\u0000\u0000\u0000\u0000\u0000\u0000\u0000\u0000\u0000\u0001\u0000\u00008\u0000\u0000\u0000\u0000\u0000\u0000\u0000\u001a\u0000\u0000\u0000<\u0002\u0000\u0000<\u0001\u0000\u00008\u0001\u0000\u0000x...", "RSRC\r\n\u0000\u0003LVCCLBVW\u0000\u00008Ð\u0000\u0000\u0003è\u0000\u0000\u0000 \u0000\u00008°\u0000\u0000\u0000x\t\u0000\u0000\u0000\u0000\u0000\u0000 \u0000\u0000\u0000\u0000\u0000\u0000\u0004\u0000\u0003\u0000<\u0000¼\u0000\u001f@\u0000\u0002\u0000\u0000\u0000\u0000\u0001\u0000\u0001\u0000\u0006ÿÿÿÿ\u0000\u0000\u0000\u0000\u0000\u0000\u0000\u0000\u0000\u0000\u0000\u0000\u001crÇd.²F´úÐL>\n\u001fr\u0000\u0000\u0000\n\u0000\u0000\u0000\u0010\u0000\u0000\u0000\u0000F->Ô7^CWIq¼àrÔ\u001dÙ\u0000²\u0004é\tìøB~\u0000\u0000@\u0000\u0000\u0000\u0000\u0000\u0000\u0000\u0000\u0010\u0000\u0000\u0000\u0000\u0000\u0000\u0000\u0000\u0000\u0000\u0000\u0000\u0000\u0000\u0000\u0000\u0000\u0000\u0000*\u0000\u0001LVCC\u001bVertical HW Info Button.ctl\u0000\u0000\u0000\u0000\u0000\u0000\u0000\u0003\u0000\u0000\u0000\u0000\u0000\u0002\u0000\u0001\u0000\u0000\u0000\u0000\u0000\u0014\u0000\b\u0000\u0002\u0010\u0000\u0010\u0001\u0010\u0000\u0010\u0004\u0010\u00000\u0000\u0010\b\u0010\u0000\u0000\u0000\u0000A\u0000\u0000\u0001\u0011xc`À\u0004ÿ\u0000H12007\u0000iVtñÿPE+Å\u0000Ù\\lv\u0010i/#P\u0011Ó\u0007 \u0001ì\u0011\u0010fú\u0003ÄÿPTaÑ\t\u0000´Ò e\u0000\u0000\u0000\u0000\u0000\u0000*\u0000\u0001VIDS\u001bVertical HW Info Button.ctl\u0000\u0000\u0000\u0000\u0000\u0000\u0000\u0003\u0000\u0000\u0000\u0000\u0000\u0000\u0000\u0000Ôxg``È4¶0Æ\u0000Éù)© ú\u0000\u0010¿f=<!´;G#80(,¼»DE¥»FE\u001f\u001bÿ>y\u001b;\u0018\nKXwô²yX42ìÐ\u0002ÊtºiìP\u0002Ó\u000e;âÁ´Kè\u000bÎÞ\u0014\u0015\u0016¶6 ÿ Ð\u001cQÿ\u0000$ÏÈÀÌËPÊPË\fý]\\ù 7\u0003\u0000Â\u000308\u0000\u0000\u0000\u0000\u0000\u0000\r\t\u0001\u0011\u0000\u0000\u00059.0.1\u0000\u0000\u0000\u0000\u0000\u0000\u0000\u0000\u0000\u000f\u0000\u0000\u0000 \u0000\u0000\u0018\u0000\u0001\u0000\f\u0000\u0000\u0000\u0004\u0000\u0002\u0000¶\u0000\u0000÷þ\u0000\u0005ðÿ\u0000\u0007øÿ@\u0007øÿ@\u000føÿ\u0004\u0007øÿ...", "RSRC\r\n\u0000\u0003LVCCLBVW\u0000\u0000Eä\u0000\u0000\u0003å\u0000\u0000\u0000 \u0000\u0000EÄ\u0000\u0000\u0000x\t\u0000\u0000\u0000\u0000\u0000\u0000 \u0000\u0000\u0000\u0000\u0000\u0000\u0004\u0000\u0003\u0000<\u0000¼\u0000\u001f@\u0000\u0002\u0000\u0000\u0000\u0000\u0001\u0000\u0001\u0000\u0006ÿÿÿÿ\u0000\u0000\u0000\u0000\u0000\u0000\u0000\u0000\u0000\u0000\u0000\u0000`ô3íy ÞD²ºT$Ù\u0004\u0000\u0000\u0000\n\u0000\u0000\u0000\u0010\u0000\u0000\u0000\u0000äx\u001d*4\u001bÀI¥q\u0002ÕYÔ\u001dÙ\u0000²\u0004é\tìøB~\u0000\u0000@\u0000\u0000\u0000\u0000\u0000\u0000\u0000\u0000\u0010\u0000\u0000\u0000\u0000\u0000\u0000\u0000\u0000\u0000\u0000\u0000\u0000\u0000\u0000\u0000\u0000\u0000\u0000\u0000(\u0000\u0001LVCC\u0018Vertical Info Button.ctl\u0000\u0000\u0000\u0000\u0000\u0000\u0000\u0000\u0003\u0000\u0000\u0000\u0002\u0000\u0001\u0000\u0000\u0000\u0000\u0000\u0014\u0000\b\u0000\u0002\u0010\u0000\u0010\u0001\u0010\u0000\u0010\u0004\u0010\u00000\u0000\u0010\b\u0010\u0000\u0000\u0000\u0000A\u0000\u0000\u0001\u0011xc`À\u0004ÿ\u0000H12007\u0000iVtñÿPE+Å\u0000Ù\\lv\u0010i/#P\u0011Ó\u0007 \u0001ì\u0011\u0010fú\u0003ÄÿPTaÑ\t\u0000´Ò e\u0000\u0000\u0000\u0000\u0000\u0000(\u0000\u0001VIDS\u0018Vertical Info Button.ctl\u0000\u0000\u0000\u0000\u0000\u0000\u0000\u0000\u0003\u0000\u0000\u0000\u0000\u0000\u0000Ôxg``È4¶0Æ\u0000Éù)© ú\u0000\u0010¿f=<!´;G#80(,¼»DE¥»FE\u001f\u001bÿ>y\u001b;\u0018\nKXwô²yX42ìÐ\u0002ÊtºiìP\u0002Ó\u000e;âÁ´Kè\u000bÎÞ\u0014\u0015\u0016¶6 ÿ Ð\u001cQÿ\u0000$ÏÈÀÌËPÊPË\fý]\\ù 7\u0003\u0000Â\u000308\u0000\u0000\u0000\u0000\u0000\u0000\r\t\u0001\u0011\u0000\u0000\u00059.0.1\u0000\u0000\u0000\u0000\u0000\u0000\u0000\u0000\u0000\u0000\u0000\u0000\u0000\u0000\u0000\u0000\u0007à\u0000\u0000?ü\u0000\u0000à\u0007\u0000\u0001À\u0001\u0003\u0000\u0000À\u0006\u0000\u0000`\f\u0000\u0000 \f\u0000\u00000\u0018\u0000\u0000\u0018\u001fü?\u0018\u001fÿÿø\u001fÿÿø...", "RSRC\r\n\u0000\u0003LVCCLBVW\u0000\u0000;¸\u0000\u0000\u0003å\u0000\u0000\u0000 \u0000\u0000;\u0000\u0000\u0000x\t\u0000\u0000\u0000\u0000\u0000\u0000 \u0000\u0000\u0000\u0000\u0000\u0000\u0004\u0000\u0003\u0000<\u0000¼\u0000\u001f@\u0000\u0002\u0000\u0000\u0000\u0000\u0001\u0000\u0001\u0000\u0006ÿÿÿÿ\u0000\u0000\u0000\u0000\u0000\u0000\u0000\u0000\u0000\u0000\u0000\u0000E¶ì\u0013<W\bJI³Hª¢@\u0000\u0000\u0000\n\u0000\u0000\u0000\u0010\u0000\u0000\u0000\u0000W\t5m¬\u0019IÇ\u001cBC|*dÔ\u001dÙ\u0000²\u0004é\tìøB~\u0000\u0000@\u0000\u0000\u0000\u0000\u0000\u0000\u0000\u0000\u0010\u0000\u0000\u0000\u0000\u0000\u0000\u0000\u0000\u0000\u0000\u0000\u0000\u0000\u0000\u0000\u0000\u0000\u0000\u0000(\u0000\u0001LVCC\u0018Vertical Load Button.ctl\u0000\u0000\u0000\u0000\u0000\u0000\u0000\u0000\u0003\u0000\u0000\u0000\u0002\u0000\u0001\u0000\u0000\u0000\u0000\u0000\u0014\u0000\b\u0000\u0002\u0010\u0000\u0010\u0001\u0010\u0000\u0010\u0004\u0010\u00000\u0000\u0010\b\u0010\u0000\u0000\u0000\u0000A\u0000\u0000\u0001\u0011xc`À\u0004ÿ\u0000H12007\u0000iVtñÿPE+Å\u0000Ù\\lv\u0010i/#P\u0011Ó\u0007 \u0001ì\u0011\u0010fú\u0003ÄÿPTaÑ\t\u0000´Ò e\u0000\u0000\u0000\u0000\u0000\u0000(\u0000\u0001VIDS\u0018Vertical Load Button.ctl\u0000\u0000\u0000\u0000\u0000\u0000\u0000\u0000\u0003\u0000\u0000\u0000\u0000\u0000\u0000Ôxg``È4¶0Æ\u0000Éù)© ú\u0000\u0010¿f=<!´;G#80(,¼»DE¥»FE\u001f\u001bÿ>y\u001b;\u0018\nKXwô²yX42ìÐ\u0002ÊtºiìP\u0002Ó\u000e;âÁ´Kè\u000bÎÞ\u0014\u0015\u0016¶6 ÿ Ð\u001cQÿ\u0000$ÏÈÀÌËPÊPË\fý]\\ù 7\u0003\u0000Â\u000308\u0000\u0000\u0000\u0000\u0000\u0000\r\t\u0001\u0011\u0000\u0000\u00059.0.1\u0000\u0000\u0000\u0000\u0000\u0000\u0000\u0000\u0000\u0000\u0000\u0000\u0000\u0000\u0000\u0000\u0000\u0000\u0000\u0000\u0000 \u0000\u0000\u0000 \u0000\u0000\u0000 \u0000\u0000\u0000 \u0000\u0000\u0000 \u0000\u0000\u0000 \u0000\u0000@ \u0000\u0000@ \u0000\u0000@ \u0000\u0000@ \u0000\u0000@ \u0000...", "RSRC\r\n\u0000\u0003LVCCLBVW\u0000\u000074\u0000\u0000\u0003å\u0000\u0000\u0000 \u0000\u00007\u0014\u0000\u0000\u0000x\t\u0000\u0000\u0000\u0000\u0000\u0000 \u0000\u0000\u0000\u0000\u0000\u0000\u0004\u0000\u0003\u0000<\u0000¼\u0000\u001f@\u0000\u0002\u0000\u0000\u0000\u0000\u0001\u0000\u0001\u0000\u0006ÿÿÿÿ\u0000\u0000\u0000\u0000\u0000\u0000\u0000\u0000\u0000\u0000\u0000\u0000üÍ úå@¶ÆB^LTO\u0000\u0000\u0000\n\u0000\u0000\u0000\u0010\u0000\u0000\u0000\u0000ø®j\u0001\u001aDAö§ÒmÔ\u001dÙ\u0000²\u0004é\tìøB~\u0000\u0000@\u0000\u0000\u0000\u0000\u0000\u0000\u0000\u0000\u0010\u0000\u0000\u0000\u0000\u0000\u0000\u0000\u0000\u0000\u0000\u0000\u0000\u0000\u0000\u0000\u0000\u0000\u0000\u0000(\u0000\u0001LVCC\u0018Vertical Mail Button.ctl\u0000\u0000\u0000\u0000\u0000\u0000\u0000\u0000\u0003\u0000\u0000\u0000\u0002\u0000\u0001\u0000\u0000\u0000\u0000\u0000\u0014\u0000\b\u0000\u0002\u0010\u0000\u0010\u0001\u0010\u0000\u0010\u0004\u0010\u00000\u0000\u0010\b\u0010\u0000\u0000\u0000\u0000A\u0000\u0000\u0001\u0011xc`À\u0004ÿ\u0000H12007\u0000iVtñÿPE+Å\u0000Ù\\lv\u0010i/#P\u0011Ó\u0007 \u0001ì\u0011\u0010fú\u0003ÄÿPTaÑ\t\u0000´Ò e\u0000\u0000\u0000\u0000\u0000\u0000(\u0000\u0001VIDS\u0018Vertical Mail Button.ctl\u0000\u0000\u0000\u0000\u0000\u0000\u0000\u0000\u0003\u0000\u0000\u0000\u0000\u0000\u0000Ôxg``È4¶0Æ\u0000Éù)© ú\u0000\u0010¿f=<!´;G#80(,¼»DE¥»FE\u001f\u001bÿ>y\u001b;\u0018\nKXwô²yX42ìÐ\u0002ÊtºiìP\u0002Ó\u000e;âÁ´Kè\u000bÎÞ\u0014\u0015\u0016¶6 ÿ Ð\u001cQÿ\u0000$ÏÈÀÌËPÊPË\fý]\\ù 7\u0003\u0000Â\u000308\u0000\u0000\u0000\u0000\u0000\u0000\r\t\u0001\u0011\u0000\u0000\u00059.0.1\u0000\u0000\u0000\u0000\u0000\u0000\u0000\u0000\u0000\u0000\u0000\u0000\u0000\u0000\u0000\u0000\u0000\u0000\u0000\u0000\u0000\u0000\u0000\u0000\u0000\u0000\u0000\u0000\u0000\u0000\u0000\u0000\u0000\u0000\u0000\u0000\u0000\u0000\u0000\u0000\u0000\u0000\u0000\u0000\u0000\u0000\u0000\u0000\u0000\u0000\u0000\u0000\u0000\u0000\u0000\u0000\u0000\u0000\u0000\u0000\u0000\u0000\u0000...", "RSRC\r\n\u0000\u0003LVCCLBVW\u0000\u00005ì\u0000\u0000\u0003å\u0000\u0000\u0000 \u0000\u00005Ì\u0000\u0000\u0000x\t\u0000\u0000\u0000\u0000\u0000\u0000 \u0000\u0000\u0000\u0000\u0000\u0000\u0004\u0000\u0003\u0000<\u0000¼\u0000\u001f@\u0000\u0002\u0000\u0000\u0000\u0000\u0001\u0000\u0001\u0000\u0006ÿÿÿÿ\u0000\u0000\u0000\u0000\u0000\u0000\u0000\u0000\u0000\u0000\u0000\u0000ÄD&äwþLO¢4jUë[\u0016h\u0000\u0000\u0000\n\u0000\u0000\u0000\u0010\u0000\u0000\u0000\u0000úâ£\u0011ímÉI³¶]C¶ñ­SÔ\u001dÙ\u0000²\u0004é\tìøB~\u0000\u0000@\u0000\u0000\u0000\u0000\u0000\u0000\u0000\u0000\u0010\u0000\u0000\u0000\u0000\u0000\u0000\u0000\u0000\u0000\u0000\u0000\u0000\u0000\u0000\u0000\u0000\u0000\u0000\u0000(\u0000\u0001LVCC\u0018Vertical Next Button.ctl\u0000\u0000\u0000\u0000\u0000\u0000\u0000\u0000\u0003\u0000\u0000\u0000\u0002\u0000\u0001\u0000\u0000\u0000\u0000\u0000\u0014\u0000\b\u0000\u0002\u0010\u0000\u0010\u0001\u0010\u0000\u0010\u0004\u0010\u00000\u0000\u0010\b\u0010\u0000\u0000\u0000\u0000A\u0000\u0000\u0001\u0011xc`À\u0004ÿ\u0000H12007\u0000iVtñÿPE+Å\u0000Ù\\lv\u0010i/#P\u0011Ó\u0007 \u0001ì\u0011\u0010fú\u0003ÄÿPTaÑ\t\u0000´Ò e\u0000\u0000\u0000\u0000\u0000\u0000(\u0000\u0001VIDS\u0018Vertical Next Button.ctl\u0000\u0000\u0000\u0000\u0000\u0000\u0000\u0000\u0003\u0000\u0000\u0000\u0000\u0000\u0000Ôxg``È4¶0Æ\u0000Éù)© ú\u0000\u0010¿f=<!´;G#80(,¼»DE¥»FE\u001f\u001bÿ>y\u001b;\u0018\nKXwô²yX42ìÐ\u0002ÊtºiìP\u0002Ó\u000e;âÁ´Kè\u000bÎÞ\u0014\u0015\u0016¶6 ÿ Ð\u001cQÿ\u0000$ÏÈÀÌËPÊPË\fý]\\ù 7\u0003\u0000Â\u000308\u0000\u0000\u0000\u0000\u0000\u0000\r\t\u0001\u0011\u0000\u0000\u00059.0.1\u0000\u0000\u0000\u0000\u0000\u0000\u0000\u0000\u0000\u0000\u0000\u0000\b\u0000\u0000\u0000\f\u0000\u0000\u0000\n\u0000\u0000\u0000\t\u0000\u0000\u0000\n\u0000\u0000\u000b@\u0000û \u0000@\u0003Ð\u0000_ÿè\u0000_ÿö\u0000_ÿÿ\u0000_ÿÿ_ÿÿÀ...", "RSRC\r\n\u0000\u0003LVCCLBVW\u0000\u00002P\u0000\u0000\u0003ã\u0000\u0000\u0000 \u0000\u000020\u0000\u0000\u0000x\t\u0000\u0000\u0000\u0000\u0000\u0000 \u0000\u0000\u0000\u0000\u0000\u0000\u0004\u0000\u0003\u0000<\u0000¼\u0000\u001f@\u0000\u0002\u0000\u0000\u0000\u0000\u0001\u0000\u0001\u0000\u0006ÿÿÿÿ\u0000\u0000\u0000\u0000\u0000\u0000\u0000\u0000\u0000\u0000\u0000\u0000cï¨ÍúÎ@·¨¥Î01C¹\u0000\u0000\u0000\n\u0000\u0000\u0000\u0010\u0000\u0000\u0000\u0000wñ^±\u000eøENÊÉ¥\u001f_ÁÔ\u001dÙ\u0000²\u0004é\tìøB~\u0000\u0000@\u0000\u0000\u0000\u0000\u0000\u0000\u0000\u0000\u0010\u0000\u0000\u0000\u0000\u0000\u0000\u0000\u0000\u0000\u0000\u0000\u0000\u0000\u0000\u0000\u0000\u0000\u0000\u0000&\u0000\u0001LVCC\u0016Vertical OK Button.ctl\u0000\u0000\u0000\u0000\u0000\u0000\u0000\u0000\u0003\u0000\u0000\u0000\u0000\u0000\u0002\u0000\u0001\u0000\u0000\u0000\u0000\u0000\u0014\u0000\b\u0000\u0002\u0010\u0000\u0010\u0001\u0010\u0000\u0010\u0004\u0010\u00000\u0000\u0010\b\u0010\u0000\u0000\u0000\u0000A\u0000\u0000\u0001\u0011xc`À\u0004ÿ\u0000H12007\u0000iVtñÿPE+Å\u0000Ù\\lv\u0010i/#P\u0011Ó\u0007 \u0001ì\u0011\u0010fú\u0003ÄÿPTaÑ\t\u0000´Ò e\u0000\u0000\u0000\u0000\u0000\u0000&\u0000\u0001VIDS\u0016Vertical OK Button.ctl\u0000\u0000\u0000\u0000\u0000\u0000\u0000\u0000\u0003\u0000\u0000\u0000\u0000\u0000\u0000\u0000\u0000Ôxg``È4¶0Æ\u0000Éù)© ú\u0000\u0010¿f=<!´;G#80(,¼»DE¥»FE\u001f\u001bÿ>y\u001b;\u0018\nKXwô²yX42ìÐ\u0002ÊtºiìP\u0002Ó\u000e;âÁ´Kè\u000bÎÞ\u0014\u0015\u0016¶6 ÿ Ð\u001cQÿ\u0000$ÏÈÀÌËPÊPË\fý]\\ù 7\u0003\u0000Â\u000308\u0000\u0000\u0000\u0000\u0000\u0000\r\t\u0001\u0011\u0000\u0000\u00059.0.1\u0000\u0000\u0000\u0000\u0000\u0000\u0000\u0000\u0000\u0000\u0000\u0000\u0000\u0000\u0000\u0000\u0000\u0000\u0000\u0000\u0000\u0001\u0000\u0000\u0000\u0002@\u0000\u0000\u0004`\u0000\u0000\b0\u0000\u0000\u0010\u0010\u0004\u0000  \t\u0000@@\u00180A\u0001 \"\u0003\u0000\u0018\u0014\u0006\u0000...", "RSRC\r\n\u0000\u0003LVCCLBVW\u0000\u00002\b\u0000\u0000\u0003å\u0000\u0000\u0000 \u0000\u00001è\u0000\u0000\u0000x\t\u0000\u0000\u0000\u0000\u0000\u0000 \u0000\u0000\u0000\u0000\u0000\u0000\u0004\u0000\u0003\u0000<\u0000¼\u0000\u001f@\u0000\u0002\u0000\u0000\u0000\u0000\u0001\u0000\u0001\u0000\u0006ÿÿÿÿ\u0000\u0000\u0000\u0000\u0000\u0000\u0000\u0000\u0000\u0000\u0000\u0000\u0016f\bWâ\u000eèLG?ý¸\u000e\u00037\u0000\u0000\u0000\n\u0000\u0000\u0000\u0010\u0000\u0000\u0000\u0000uæ\u001dß\u001b\u000b8GU\fÙ8xJÔ\u001dÙ\u0000²\u0004é\tìøB~\u0000\u0000@\u0000\u0000\u0000\u0000\u0000\u0000\u0000\u0000\u0010\u0000\u0000\u0000\u0000\u0000\u0000\u0000\u0000\u0000\u0000\u0000\u0000\u0000\u0000\u0000\u0000\u0000\u0000\u0000(\u0000\u0001LVCC\u0018Vertical Open Button.ctl\u0000\u0000\u0000\u0000\u0000\u0000\u0000\u0000\u0003\u0000\u0000\u0000\u0002\u0000\u0001\u0000\u0000\u0000\u0000\u0000\u0014\u0000\b\u0000\u0002\u0010\u0000\u0010\u0001\u0010\u0000\u0010\u0004\u0010\u00000\u0000\u0010\b\u0010\u0000\u0000\u0000\u0000A\u0000\u0000\u0001\u0011xc`À\u0004ÿ\u0000H12007\u0000iVtñÿPE+Å\u0000Ù\\lv\u0010i/#P\u0011Ó\u0007 \u0001ì\u0011\u0010fú\u0003ÄÿPTaÑ\t\u0000´Ò e\u0000\u0000\u0000\u0000\u0000\u0000(\u0000\u0001VIDS\u0018Vertical Open Button.ctl\u0000\u0000\u0000\u0000\u0000\u0000\u0000\u0000\u0003\u0000\u0000\u0000\u0000\u0000\u0000Ôxg``È4¶0Æ\u0000Éù)© ú\u0000\u0010¿f=<!´;G#80(,¼»DE¥»FE\u001f\u001bÿ>y\u001b;\u0018\nKXwô²yX42ìÐ\u0002ÊtºiìP\u0002Ó\u000e;âÁ´Kè\u000bÎÞ\u0014\u0015\u0016¶6 ÿ Ð\u001cQÿ\u0000$ÏÈÀÌËPÊPË\fý]\\ù 7\u0003\u0000Â\u000308\u0000\u0000\u0000\u0000\u0000\u0000\r\t\u0001\u0011\u0000\u0000\u00059.0.1\u0000\u0000\u0000\u0000\u0000\u0000\u0000\u0000\u0000\u0000\u0000\u0000\u0000\u0000\u0000\u0000\u001fþ\u0000\u0000\u0010\u0000\u0000\u0010\u0000@\u0000\u0010\u0000\u0000\u0007ð\u0000\u0000\u0000\u0010\u0000\u0000\u0000\u0010\u0000\b\b\u0010\u0000\b\b\u0010\u0000\b\b\u0010\u0000\b\b\u0010\u0000\b\bÿÿþ...", "RSRC\r\n\u0000\u0003LVCCLBVW\u0000\u0000@ô\u0000\u0000\u0003æ\u0000\u0000\u0000 \u0000\u0000@Ô\u0000\u0000\u0000x\t\u0000\u0000\u0000\u0000\u0000\u0000 \u0000\u0000\u0000\u0000\u0000\u0000\u0004\u0000\u0003\u0000<\u0000¼\u0000\u001f@\u0000\u0002\u0000\u0000\u0000\u0000\u0001\u0000\u0001\u0000\u0006ÿÿÿÿ\u0000\u0000\u0000\u0000\u0000\u0000\u0000\u0000\u0000\u0000\u0000\u0000·ÄTopØAÅ'\u001b-Óõ\u0000\u0000\u0000\n\u0000\u0000\u0000\u0010\u0000\u0000\u0000\u0000g¡±v´ÛD«M^Ór¸µÔ\u001dÙ\u0000²\u0004é\tìøB~\u0000\u0000@\u0000\u0000\u0000\u0000\u0000\u0000\u0000\u0000\u0010\u0000\u0000\u0000\u0000\u0000\u0000\u0000\u0000\u0000\u0000\u0000\u0000\u0000\u0000\u0000\u0000\u0000\u0000\u0000(\u0000\u0001LVCC\u0019Vertical Pause Button.ctl\u0000\u0000\u0000\u0000\u0000\u0000\u0000\u0003\u0000\u0000\u0000\u0002\u0000\u0001\u0000\u0000\u0000\u0000\u0000\u0014\u0000\b\u0000\u0002\u0010\u0000\u0010\u0001\u0010\u0000\u0010\u0004\u0010\u00000\u0000\u0010\b\u0010\u0000\u0000\u0000\u0000A\u0000\u0000\u0001\u0011xc`À\u0004ÿ\u0000H12007\u0000iVtñÿPE+Å\u0000Ù\\lv\u0010i/#P\u0011Ó\u0007 \u0001ì\u0011\u0010fú\u0003ÄÿPTaÑ\t\u0000´Ò e\u0000\u0000\u0000\u0000\u0000\u0000(\u0000\u0001VIDS\u0019Vertical Pause Button.ctl\u0000\u0000\u0000\u0000\u0000\u0000\u0000\u0003\u0000\u0000\u0000\u0000\u0000\u0000Ôxg``È4¶0Æ\u0000Éù)© ú\u0000\u0010¿f=<!´;G#80(,¼»DE¥»FE\u001f\u001bÿ>y\u001b;\u0018\nKXwô²yX42ìÐ\u0002ÊtºiìP\u0002Ó\u000e;âÁ´Kè\u000bÎÞ\u0014\u0015\u0016¶6 ÿ Ð\u001cQÿ\u0000$ÏÈÀÌËPÊPË\fý]\\ù 7\u0003\u0000Â\u000308\u0000\u0000\u0000\u0000\u0000\u0000\r\t\u0001\u0011\u0000\u0000\u00059.0.1\u0000\u0000\u0000\u0000\u0000\u0000\u0000\u0000\u0000\u0000\u0000\u0000\u0000\u0000\u0000\u001fà\u0007ü00\f\u0004 \u0010\f\u0004 \u0010\f\u0004 \u0010\f\u0004 0\f\u0004 0\f\u000400\f\u000400\f\f00\f\f00\f\f7°\rì...", "RSRC\r\n\u0000\u0003LVCCLBVW\u0000\u0000<´\u0000\u0000\u0003æ\u0000\u0000\u0000 \u0000\u0000<\u0000\u0000\u0000x\t\u0000\u0000\u0000\u0000\u0000\u0000 \u0000\u0000\u0000\u0000\u0000\u0000\u0004\u0000\u0003\u0000<\u0000¼\u0000\u001f@\u0000\u0002\u0000\u0000\u0000\u0000\u0001\u0000\u0001\u0000\u0006ÿÿÿÿ\u0000\u0000\u0000\u0000\u0000\u0000\u0000\u0000\u0000\u0000\u0000\u0000GS\u0012à\\ÆBAS\u000b\u0018\nøåR\u0000\u0000\u0000\n\u0000\u0000\u0000\u0010\u0000\u0000\u0000\u0000=iæ\u001a÷bL³p\u0004ö#µÔ\u001dÙ\u0000²\u0004é\tìøB~\u0000\u0000@\u0000\u0000\u0000\u0000\u0000\u0000\u0000\u0000\u0010\u0000\u0000\u0000\u0000\u0000\u0000\u0000\u0000\u0000\u0000\u0000\u0000\u0000\u0000\u0000\u0000\u0000\u0000\u0000(\u0000\u0001LVCC\u0019Vertical Print Button.ctl\u0000\u0000\u0000\u0000\u0000\u0000\u0000\u0003\u0000\u0000\u0000\u0002\u0000\u0001\u0000\u0000\u0000\u0000\u0000\u0014\u0000\b\u0000\u0002\u0010\u0000\u0010\u0001\u0010\u0000\u0010\u0004\u0010\u00000\u0000\u0010\b\u0010\u0000\u0000\u0000\u0000A\u0000\u0000\u0001\u0011xc`À\u0004ÿ\u0000H12007\u0000iVtñÿPE+Å\u0000Ù\\lv\u0010i/#P\u0011Ó\u0007 \u0001ì\u0011\u0010fú\u0003ÄÿPTaÑ\t\u0000´Ò e\u0000\u0000\u0000\u0000\u0000\u0000(\u0000\u0001VIDS\u0019Vertical Print Button.ctl\u0000\u0000\u0000\u0000\u0000\u0000\u0000\u0003\u0000\u0000\u0000\u0000\u0000\u0000Ôxg``È4¶0Æ\u0000Éù)© ú\u0000\u0010¿f=<!´;G#80(,¼»DE¥»FE\u001f\u001bÿ>y\u001b;\u0018\nKXwô²yX42ìÐ\u0002ÊtºiìP\u0002Ó\u000e;âÁ´Kè\u000bÎÞ\u0014\u0015\u0016¶6 ÿ Ð\u001cQÿ\u0000$ÏÈÀÌËPÊPË\fý]\\ù 7\u0003\u0000Â\u000308\u0000\u0000\u0000\u0000\u0000\u0000\r\t\u0001\u0011\u0000\u0000\u00059.0.1\u0000\u0000\u0000\u0000\u0000\u0000\u0000\u0000\u0000\u0000\u0000\u0000\u0000\u0000\u0000\u0000\u0000\u0000\u0000\u0000\u0000\u0000\u0000\u0000\u0000\u0000\u0000\u0000\u0000\u0000\u0000\u0000\u0000\u0000\u0000\u0000\u0000\u0000\u0000\u0000\u0000\u0000\u0000\u0000\u0000\u0000\u0000\u0000\u0000\u0000\u0000\u0000\u0000\u0000\u0000\u0000\u0000\u0000\u0000\u0000\u0000\u0000\u0000...", "RSRC\r\n\u0000\u0003LVCCLBVW\u0000\u0000T\u0000\u0000\u0003ç\u0000\u0000\u0000 \u0000\u0000T`\u0000\u0000\u0000x\t\u0000\u0000\u0000\u0000\u0000\u0000 \u0000\u0000\u0000\u0000\u0000\u0000\u0004\u0000\u0003\u0000<\u0000¼\u0000\u001f@\u0000\u0002\u0000\u0000\u0000\u0000\u0001\u0000\u0001\u0000\u0006ÿÿÿÿ\u0000\u0000\u0000\u0000\u0000\u0000\u0000\u0000\u0000\u0000\u0000\u0000î\u001b·\"J\"O¼\u0010ÒS\u0003vô\u0000\u0000\u0000\n\u0000\u0000\u0000\u0010\u0000\u0000\u0000\u0000\n\u00186ú%×ÄB´LÉá\u001cþa*Ô\u001dÙ\u0000²\u0004é\tìøB~\u0000\u0000@\u0000\u0000\u0000\u0000\u0000\u0000\u0000\u0000\u0010\u0000\u0000\u0000\u0000\u0000\u0000\u0000\u0000\u0000\u0000\u0000\u0000\u0000\u0000\u0000\u0000\u0000\u0000\u0000*\u0000\u0001LVCC\u001aVertical Record Button.ctl\u0000\u0000\u0000\u0000\u0000\u0000\u0000\u0000\u0003\u0000\u0000\u0000\u0000\u0000\u0002\u0000\u0001\u0000\u0000\u0000\u0000\u0000\u0014\u0000\b\u0000\u0002\u0010\u0000\u0010\u0001\u0010\u0000\u0010\u0004\u0010\u00000\u0000\u0010\b\u0010\u0000\u0000\u0000\u0000A\u0000\u0000\u0001\u0011xc`À\u0004ÿ\u0000H12007\u0000iVtñÿPE+Å\u0000Ù\\lv\u0010i/#P\u0011Ó\u0007 \u0001ì\u0011\u0010fú\u0003ÄÿPTaÑ\t\u0000´Ò e\u0000\u0000\u0000\u0000\u0000\u0000*\u0000\u0001VIDS\u001aVertical Record Button.ctl\u0000\u0000\u0000\u0000\u0000\u0000\u0000\u0000\u0003\u0000\u0000\u0000\u0000\u0000\u0000\u0000\u0000Ôxg``È4¶0Æ\u0000Éù)© ú\u0000\u0010¿f=<!´;G#80(,¼»DE¥»FE\u001f\u001bÿ>y\u001b;\u0018\nKXwô²yX42ìÐ\u0002ÊtºiìP\u0002Ó\u000e;âÁ´Kè\u000bÎÞ\u0014\u0015\u0016¶6 ÿ Ð\u001cQÿ\u0000$ÏÈÀÌËPÊPË\fý]\\ù 7\u0003\u0000Â\u000308\u0000\u0000\u0000\u0000\u0000\u0000\r\t\u0001\u0011\u0000\u0000\u00059.0.1\u0000\u0000\u0000\u0000\u0000\u0000\u0000\u0000\u0000\u0000\u0000\u0000\u0000\u0000\u0000\u0000\u0000\u0000\u0000\u0000\u0000\u0000\u0000\u0000\u0000\u0000\u0000\u0000\u0000\u0000\u0000\u0000\u0000\u0000\u0000\u0000\u0003À\u0000\u0000\b\u0010\u0000\u0000 \u0004\u0000\u0000@\u0002\u0000\u0000\u0000\u0000\u0000...", "RSRC\r\n\u0000\u0003LVCCLBVW\u0000\u0000?è\u0000\u0000\u0003è\u0000\u0000\u0000 \u0000\u0000?È\u0000\u0000\u0000x\t\u0000\u0000\u0000\u0000\u0000\u0000 \u0000\u0000\u0000\u0000\u0000\u0000\u0004\u0000\u0003\u0000<\u0000¼\u0000\u001f@\u0000\u0002\u0000\u0000\u0000\u0000\u0001\u0000\u0001\u0000\u0006ÿÿÿÿ\u0000\u0000\u0000\u0000\u0000\u0000\u0000\u0000\u0000\u0000\u0000\u0000|@\"ð`\u0015ìLªÒ~}ÑE2æ\u0000\u0000\u0000\n\u0000\u0000\u0000\u0010\u0000\u0000\u0000\u0000\u0018ÏCÝW\u0000kK¯õ\u0002¨tðºÔ\u001dÙ\u0000²\u0004é\tìøB~\u0000\u0000@\u0000\u0000\u0000\u0000\u0000\u0000\u0000\u0000\u0010\u0000\u0000\u0000\u0000\u0000\u0000\u0000\u0000\u0000\u0000\u0000\u0000\u0000\u0000\u0000\u0000\u0000\u0000\u0000*\u0000\u0001LVCC\u001bVertical Refresh Button.ctl\u0000\u0000\u0000\u0000\u0000\u0000\u0000\u0003\u0000\u0000\u0000\u0000\u0000\u0002\u0000\u0001\u0000\u0000\u0000\u0000\u0000\u0014\u0000\b\u0000\u0002\u0010\u0000\u0010\u0001\u0010\u0000\u0010\u0004\u0010\u00000\u0000\u0010\b\u0010\u0000\u0000\u0000\u0000A\u0000\u0000\u0001\u0011xc`À\u0004ÿ\u0000H12007\u0000iVtñÿPE+Å\u0000Ù\\lv\u0010i/#P\u0011Ó\u0007 \u0001ì\u0011\u0010fú\u0003ÄÿPTaÑ\t\u0000´Ò e\u0000\u0000\u0000\u0000\u0000\u0000*\u0000\u0001VIDS\u001bVertical Refresh Button.ctl\u0000\u0000\u0000\u0000\u0000\u0000\u0000\u0003\u0000\u0000\u0000\u0000\u0000\u0000\u0000\u0000Ôxg``È4¶0Æ\u0000Éù)© ú\u0000\u0010¿f=<!´;G#80(,¼»DE¥»FE\u001f\u001bÿ>y\u001b;\u0018\nKXwô²yX42ìÐ\u0002ÊtºiìP\u0002Ó\u000e;âÁ´Kè\u000bÎÞ\u0014\u0015\u0016¶6 ÿ Ð\u001cQÿ\u0000$ÏÈÀÌËPÊPË\fý]\\ù 7\u0003\u0000Â\u000308\u0000\u0000\u0000\u0000\u0000\u0000\r\t\u0001\u0011\u0000\u0000\u00059.0.1\u0000\u0000\u0000\u0000\u0000\u0000\u0000\u0000\u0000\u0000\u0000\u0000\u0000\u0000\u0000\u0000\u0000p\u0000\u0000\u0000x\u0000\u0000\u0000D\u0000\u0000\u0000C\u0000\u0000ÿÁ\u0003\u0000\u0000À\f\u0000\u0000@\u0018\u0000\u0000`\u0010\u0000\u0000@\"\u0000\u0000...", "RSRC\r\n\u0000\u0003LVCCLBVW\u0000\u00006X\u0000\u0000\u0003ç\u0000\u0000\u0000 \u0000\u000068\u0000\u0000\u0000x\t\u0000\u0000\u0000\u0000\u0000\u0000 \u0000\u0000\u0000\u0000\u0000\u0000\u0004\u0000\u0003\u0000<\u0000¼\u0000\u001f@\u0000\u0002\u0000\u0000\u0000\u0000\u0001\u0000\u0001\u0000\u0006ÿÿÿÿ\u0000\u0000\u0000\u0000\u0000\u0000\u0000\u0000\u0000\u0000\u0000\u0000\u0014_Ñ !P'H\u0010Ó\u0001ZÃÒ\u0000\u0000\u0000\n\u0000\u0000\u0000\u0010\u0000\u0000\u0000\u0000ú5À2_í GKMýÜ¿Ô\u001dÙ\u0000²\u0004é\tìøB~\u0000\u0000@\u0000\u0000\u0000\u0000\u0000\u0000\u0000\u0000\u0010\u0000\u0000\u0000\u0000\u0000\u0000\u0000\u0000\u0000\u0000\u0000\u0000\u0000\u0000\u0000\u0000\u0000\u0000\u0000*\u0000\u0001LVCC\u001aVertical Remove Button.ctl\u0000\u0000\u0000\u0000\u0000\u0000\u0000\u0000\u0003\u0000\u0000\u0000\u0000\u0000\u0002\u0000\u0001\u0000\u0000\u0000\u0000\u0000\u0014\u0000\b\u0000\u0002\u0010\u0000\u0010\u0001\u0010\u0000\u0010\u0004\u0010\u00000\u0000\u0010\b\u0010\u0000\u0000\u0000\u0000A\u0000\u0000\u0001\u0011xc`À\u0004ÿ\u0000H12007\u0000iVtñÿPE+Å\u0000Ù\\lv\u0010i/#P\u0011Ó\u0007 \u0001ì\u0011\u0010fú\u0003ÄÿPTaÑ\t\u0000´Ò e\u0000\u0000\u0000\u0000\u0000\u0000*\u0000\u0001VIDS\u001aVertical Remove Button.ctl\u0000\u0000\u0000\u0000\u0000\u0000\u0000\u0000\u0003\u0000\u0000\u0000\u0000\u0000\u0000\u0000\u0000Ôxg``È4¶0Æ\u0000Éù)© ú\u0000\u0010¿f=<!´;G#80(,¼»DE¥»FE\u001f\u001bÿ>y\u001b;\u0018\nKXwô²yX42ìÐ\u0002ÊtºiìP\u0002Ó\u000e;âÁ´Kè\u000bÎÞ\u0014\u0015\u0016¶6 ÿ Ð\u001cQÿ\u0000$ÏÈÀÌËPÊPË\fý]\\ù 7\u0003\u0000Â\u000308\u0000\u0000\u0000\u0000\u0000\u0000\r\t\u0001\u0011\u0000\u0000\u00059.0.1\u0000\u0000\u0000\u0000\u0000\u0000\u0000\u0000\u0000\u0000\u0000\u0000\u0000\u0000\u0000\u0000\u0000\u0000\u0000\u0000\u0000\u0000\u0000\u0000\u0000\u0000\u0000\u0000\u0000\u0000\u0000?ÿÿð \u0000\u0000\u0010 \u0000\u0000\u0010 \u0000\u0000\u0010.\u0000\u0000Ð/ÿÿÐ...", "RSRC\r\n\u0000\u0003LVCCLBVW\u0000\u0000D\u0000\u0000\u0003å\u0000\u0000\u0000 \u0000\u0000Dh\u0000\u0000\u0000x\t\u0000\u0000\u0000\u0000\u0000\u0000 \u0000\u0000\u0000\u0000\u0000\u0000\u0004\u0000\u0003\u0000<\u0000¼\u0000\u001f@\u0000\u0002\u0000\u0000\u0000\u0000\u0001\u0000\u0001\u0000\u0006ÿÿÿÿ\u0000\u0000\u0000\u0000\u0000\u0000\u0000\u0000\u0000\u0000\u0000\u0000\u0007Þ¯ß¢éÀ@¢r#¾$c\u0000\u0000\u0000\n\u0000\u0000\u0000\u0010\u0000\u0000\u0000\u0000Ç ¼ßT\u0003@yq\\m¦´\u000bÔ\u001dÙ\u0000²\u0004é\tìøB~\u0000\u0000@\u0000\u0000\u0000\u0000\u0000\u0000\u0000\u0000\u0010\u0000\u0000\u0000\u0000\u0000\u0000\u0000\u0000\u0000\u0000\u0000\u0000\u0000\u0000\u0000\u0000\u0000\u0000\u0000(\u0000\u0001LVCC\u0018Vertical Save Button.ctl\u0000\u0000\u0000\u0000\u0000\u0000\u0000\u0000\u0003\u0000\u0000\u0000\u0002\u0000\u0001\u0000\u0000\u0000\u0000\u0000\u0014\u0000\b\u0000\u0002\u0010\u0000\u0010\u0001\u0010\u0000\u0010\u0004\u0010\u00000\u0000\u0010\b\u0010\u0000\u0000\u0000\u0000A\u0000\u0000\u0001\u0011xc`À\u0004ÿ\u0000H12007\u0000iVtñÿPE+Å\u0000Ù\\lv\u0010i/#P\u0011Ó\u0007 \u0001ì\u0011\u0010fú\u0003ÄÿPTaÑ\t\u0000´Ò e\u0000\u0000\u0000\u0000\u0000\u0000(\u0000\u0001VIDS\u0018Vertical Save Button.ctl\u0000\u0000\u0000\u0000\u0000\u0000\u0000\u0000\u0003\u0000\u0000\u0000\u0000\u0000\u0000Ôxg``È4¶0Æ\u0000Éù)© ú\u0000\u0010¿f=<!´;G#80(,¼»DE¥»FE\u001f\u001bÿ>y\u001b;\u0018\nKXwô²yX42ìÐ\u0002ÊtºiìP\u0002Ó\u000e;âÁ´Kè\u000bÎÞ\u0014\u0015\u0016¶6 ÿ Ð\u001cQÿ\u0000$ÏÈÀÌËPÊPË\fý]\\ù 7\u0003\u0000Â\u000308\u0000\u0000\u0000\u0000\u0000\u0000\r\t\u0001\u0011\u0000\u0000\u00059.0.1\u0000\u0000\u0000\u0000\u0000\u0000\u0000\u0000\u0000\u0000\u0000\u0000\u0000\u0000\u0000\u001c\u0000\u00008<\u0000\u0000<<\u0000\u0000<<\u0000\u0000<<\u0000\u0000<<\u0000\u0000<<\u0000\u0000<<\u0000\u0000<<\u0000\u0000<<\u0000\u0000<<\u0000\u0000<<\u0000\u0000<...", "RSRC\r\n\u0000\u0003LVCCLBVW\u0000\u0000B@\u0000\u0000\u0003é\u0000\u0000\u0000 \u0000\u0000B \u0000\u0000\u0000x\t\u0000\u0000\u0000\u0000\u0000\u0000 \u0000\u0000\u0000\u0000\u0000\u0000\u0004\u0000\u0003\u0000<\u0000¼\u0000\u001f@\u0000\u0002\u0000\u0000\u0000\u0000\u0001\u0000\u0001\u0000\u0006ÿÿÿÿ\u0000\u0000\u0000\u0000\u0000\u0000\u0000\u0000\u0000\u0000\u0000\u0000Öxâ®p;NÏbU\t4¯¹\u0000\u0000\u0000\n\u0000\u0000\u0000\u0010\u0000\u0000\u0000\u0000îÅ\tFÁJ¾SÓ\n\u0007qkÔ\u001dÙ\u0000²\u0004é\tìøB~\u0000\u0000@\u0000\u0000\u0000\u0000\u0000\u0000\u0000\u0000\u0010\u0000\u0000\u0000\u0000\u0000\u0000\u0000\u0000\u0000\u0000\u0000\u0000\u0000\u0000\u0000\u0000\u0000\u0000\u0000,\u0000\u0001LVCC\u001cVertical Settings Button.ctl\u0000\u0000\u0000\u0000\u0000\u0000\u0000\u0000\u0003\u0000\u0000\u0000\u0002\u0000\u0001\u0000\u0000\u0000\u0000\u0000\u0014\u0000\b\u0000\u0002\u0010\u0000\u0010\u0001\u0010\u0000\u0010\u0004\u0010\u00000\u0000\u0010\b\u0010\u0000\u0000\u0000\u0000A\u0000\u0000\u0001\u0011xc`À\u0004ÿ\u0000H12007\u0000iVtñÿPE+Å\u0000Ù\\lv\u0010i/#P\u0011Ó\u0007 \u0001ì\u0011\u0010fú\u0003ÄÿPTaÑ\t\u0000´Ò e\u0000\u0000\u0000\u0000\u0000\u0000,\u0000\u0001VIDS\u001cVertical Settings Button.ctl\u0000\u0000\u0000\u0000\u0000\u0000\u0000\u0000\u0003\u0000\u0000\u0000\u0000\u0000\u0000Ôxg``È4¶0Æ\u0000Éù)© ú\u0000\u0010¿f=<!´;G#80(,¼»DE¥»FE\u001f\u001bÿ>y\u001b;\u0018\nKXwô²yX42ìÐ\u0002ÊtºiìP\u0002Ó\u000e;âÁ´Kè\u000bÎÞ\u0014\u0015\u0016¶6 ÿ Ð\u001cQÿ\u0000$ÏÈÀÌËPÊPË\fý]\\ù 7\u0003\u0000Â\u000308\u0000\u0000\u0000\u0000\u0000\u0000\r\t\u0001\u0011\u0000\u0000\u00059.0.1\u0000\u0000\u0000\u0000\u0000\u0000\u0000\u0000\u0000\u0000\u0000\u0000\u0000\u0000\u0000\u0000\u0000\u0000\u0000\u0000\u0000\u0000\u0000\u0000\u0000\u0000\u0000\u0000\u0000\u0000\u0002\u0000\u0000\u0000\u0003\u0000\u0000\u0000\u0002\u0000\u0004\u0000\b\u001f\u0004\u0000\u0000!\u0000\u0018\u0000\u0000...", "RSRC\r\n\u0000\u0003LVCCLBVW\u0000\u00008Ì\u0000\u0000\u0003æ\u0000\u0000\u0000 \u0000\u00008¬\u0000\u0000\u0000x\t\u0000\u0000\u0000\u0000\u0000\u0000 \u0000\u0000\u0000\u0000\u0000\u0000\u0004\u0000\u0003\u0000<\u0000¼\u0000\u001f@\u0000\u0002\u0000\u0000\u0000\u0000\u0001\u0000\u0001\u0000\u0006ÿÿÿÿ\u0000\u0000\u0000\u0000\u0000\u0000\u0000\u0000\u0000\u0000\u0000\u0000ðíÆéA§\u001cþ\u001aÈKì\u0000\u0000\u0000\n\u0000\u0000\u0000\u0010\u0000\u0000\u0000\u0000@'hÍ³ä\rIYÃ|P]\rÔ\u001dÙ\u0000²\u0004é\tìøB~\u0000\u0000@\u0000\u0000\u0000\u0000\u0000\u0000\u0000\u0000\u0010\u0000\u0000\u0000\u0000\u0000\u0000\u0000\u0000\u0000\u0000\u0000\u0000\u0000\u0000\u0000\u0000\u0000\u0000\u0000(\u0000\u0001LVCC\u0019Vertical Start Button.ctl\u0000\u0000\u0000\u0000\u0000\u0000\u0000\u0003\u0000\u0000\u0000\u0002\u0000\u0001\u0000\u0000\u0000\u0000\u0000\u0014\u0000\b\u0000\u0002\u0010\u0000\u0010\u0001\u0010\u0000\u0010\u0004\u0010\u00000\u0000\u0010\b\u0010\u0000\u0000\u0000\u0000A\u0000\u0000\u0001\u0011xc`À\u0004ÿ\u0000H12007\u0000iVtñÿPE+Å\u0000Ù\\lv\u0010i/#P\u0011Ó\u0007 \u0001ì\u0011\u0010fú\u0003ÄÿPTaÑ\t\u0000´Ò e\u0000\u0000\u0000\u0000\u0000\u0000(\u0000\u0001VIDS\u0019Vertical Start Button.ctl\u0000\u0000\u0000\u0000\u0000\u0000\u0000\u0003\u0000\u0000\u0000\u0000\u0000\u0000Ôxg``È4¶0Æ\u0000Éù)© ú\u0000\u0010¿f=<!´;G#80(,¼»DE¥»FE\u001f\u001bÿ>y\u001b;\u0018\nKXwô²yX42ìÐ\u0002ÊtºiìP\u0002Ó\u000e;âÁ´Kè\u000bÎÞ\u0014\u0015\u0016¶6 ÿ Ð\u001cQÿ\u0000$ÏÈÀÌËPÊPË\fý]\\ù 7\u0003\u0000Â\u000308\u0000\u0000\u0000\u0000\u0000\u0000\r\t\u0001\u0011\u0000\u0000\u00059.0.1\u0000\u0000\u0000\u0000\u0000\u0000\u0000\u0000\u0000\u0000\u0000\u0010\u0000\u0000\u0000<\u0000\u0000\u0000'\u0000\u0000\u0000!\u0000\u0000 `\u0000\u0000 8\u0000\u0000 \u000e\u0000\u0000 \u0003\u0000\u0000 \u0000À\u0000 \u0000p\u0000 \u0000\u0018\u00000\u0000\u000e\u00000\u0000\u0003...", "RSRC\r\n\u0000\u0003LVCCLBVW\u0000\u00004T\u0000\u0000\u0003å\u0000\u0000\u0000 \u0000\u000044\u0000\u0000\u0000x\t\u0000\u0000\u0000\u0000\u0000\u0000 \u0000\u0000\u0000\u0000\u0000\u0000\u0004\u0000\u0003\u0000<\u0000¼\u0000\u001f@\u0000\u0002\u0000\u0000\u0000\u0000\u0001\u0000\u0001\u0000\u0006ÿÿÿÿ\u0000\u0000\u0000\u0000\u0000\u0000\u0000\u0000\u0000\u0000\u0000\u0000ÑÑ¼ÏÏGKù\u0005¥Á4Æ\u0000\u0000\u0000\n\u0000\u0000\u0000\u0010\u0000\u0000\u0000\u0000ô ÁJï@hÈä¸(½ÅÔ\u001dÙ\u0000²\u0004é\tìøB~\u0000\u0000@\u0000\u0000\u0000\u0000\u0000\u0000\u0000\u0000\u0010\u0000\u0000\u0000\u0000\u0000\u0000\u0000\u0000\u0000\u0000\u0000\u0000\u0000\u0000\u0000\u0000\u0000\u0000\u0000(\u0000\u0001LVCC\u0018Vertical Stop Button.ctl\u0000\u0000\u0000\u0000\u0000\u0000\u0000\u0000\u0003\u0000\u0000\u0000\u0002\u0000\u0001\u0000\u0000\u0000\u0000\u0000\u0014\u0000\b\u0000\u0002\u0010\u0000\u0010\u0001\u0010\u0000\u0010\u0004\u0010\u00000\u0000\u0010\b\u0010\u0000\u0000\u0000\u0000A\u0000\u0000\u0001\u0011xc`À\u0004ÿ\u0000H12007\u0000iVtñÿPE+Å\u0000Ù\\lv\u0010i/#P\u0011Ó\u0007 \u0001ì\u0011\u0010fú\u0003ÄÿPTaÑ\t\u0000´Ò e\u0000\u0000\u0000\u0000\u0000\u0000(\u0000\u0001VIDS\u0018Vertical Stop Button.ctl\u0000\u0000\u0000\u0000\u0000\u0000\u0000\u0000\u0003\u0000\u0000\u0000\u0000\u0000\u0000Ôxg``È4¶0Æ\u0000Éù)© ú\u0000\u0010¿f=<!´;G#80(,¼»DE¥»FE\u001f\u001bÿ>y\u001b;\u0018\nKXwô²yX42ìÐ\u0002ÊtºiìP\u0002Ó\u000e;âÁ´Kè\u000bÎÞ\u0014\u0015\u0016¶6 ÿ Ð\u001cQÿ\u0000$ÏÈÀÌËPÊPË\fý]\\ù 7\u0003\u0000Â\u000308\u0000\u0000\u0000\u0000\u0000\u0000\r\t\u0001\u0011\u0000\u0000\u00059.0.1\u0000\u0000\u0000\u0000\u0000\u0000\u0000\u0000À\u0010\u0000\u0001\u0000\b\u0000\u0002\u0000\u0004\u0000\u0004\u0000\u0002\u0000\b\u0000\u0001\u0000\u0010\u0000\u00010\u0000\u0000À`\u0000\u0000`@\u0000\u0000 @\u0000\u0000 @\u0000\u0000 @\u0000\u0000 @\u0000\u0001à|@\u000fà...", "RSRC\r\n\u0000\u0003LVCCLBVW\u0000\u0000=\u0004\u0000\u0000\u00047\u0000\u0000\u0000 \u0000\u0000<ä\u0000\u0000\u0000x\t\u0000\u0000\u0000\u0000\u0000\u0000 \u0000\u0000\u0000\u0000\u0000\u0000\u0004\u0000\u0003\u0000<\u0000¼\u0000\u001f@\u0000\u0002\u0000\u0000\u0000\u0000\u0001\u0000\u0001\u0000\u0006ÿÿÿÿ\u0000\u0000\u0000\u0000\u0000\u0000\u0000\u0000\u0000\u0000\u0000\u0000>$óäFuA¶ø}Ó¾ÙH\u0001\u0000\u0000\u0000\n\u0000\u0000\u0000\u0010\u0000\u0000\u0000\u0000`HÑÕÆ\u0004Cª\u001f\\ÂCÂ\\Ô\u001dÙ\u0000²\u0004é\tìøB~\u0000\u0000@\u0000\u0000\u0000\u0000\u0000\u0000\u0000\u0000\u0010\u0000\u0000\u0000\u0000\u0000\u0000\u0000\u0000\u0000\u0000\u0000\u0000\u0000\u0000\u0000\u0000\u0000\u0000\u0000*\u0000\u0001LVCC\u001aSystem Intensity Chart.ctl\u0000\u0000\u0000\u0000\u0000\u0000\u0000\u0000\u0003\u0000\u0000\u0000\u0000\u0000\u0002\u0000\u0001\u0000\u0000\u0000\u0000\u00002\u0000\u0017\u0000\u0002\u0010\u0000\u0010\u0001 \u0000 \u0000\u0010\u0010 \u0000 \u0000 \u0000 \u0000\u0010\u0000\u0000\u0004\u0010\u00000\u0000\u0000\b\u0010\u0000\u0010\b\u0010\u0000\u0010\u0000\u0010\u0000\u0010\u0000\u0010\u0000\u0010\u0000\u0010\u0000\u0000\u0000\u0000\u0000\u0003N\u0000\u0000\u0007nx¥Ô\u0001(äY\u001c\u0007ðïÌÎjH$I$9Y9ëäæ$YIrÎYI²ÈÊÊÉÊI$I$IV$I$I$I$YÉI$I}÷;7³ËÍÎm§ûÕ§ß{óþÿ÷~ó^ÿ\u0007|\u001dT(\u0019çÊî¿Ó\u001eN^ýßñx^gk<u]-\u0019þããÏÄõö]±­ë\\Uüûûâ7Øû?¿«,[ý¾¨øóã^\u000fóYã#~1¸\u001a^ýÝþÎÉø\u000bDà/üª\u0011INøÞð\u001a\u001a>8©Üh-O\\Ä,n°\u001dxµ\u001aoñ\u0011_ñ\u0013\t@\t`\tP\tpHhXxIm'\u0013ÅZq²¤Hª¤IºdH¦dI¶äH®äI¾\u0014H¡\u0014IJKTJTKÔJÔK4J4K´J´K...", "RSRC\r\n\u0000\u0003LVCCLBVW\u0000\u00003P\u0000\u0000\u0004\u000e\u0000\u0000\u0000 \u0000\u000030\u0000\u0000\u0000x\t\u0000\u0000\u0000\u0000\u0000\u0000 \u0000\u0000\u0000\u0000\u0000\u0000\u0004\u0000\u0003\u0000<\u0000¼\u0000\u001f@\u0000\u0002\u0000\u0000\u0000\u0000\u0001\u0000\u0001\u0000\u0006ÿÿÿÿ\u0000\u0000\u0000\u0000\u0000\u0000\u0000\u0000\u0000\u0000\u0000\u0000Ö\u0002\u0011÷Ì½M¦ÍzeNÁ½Ï\u0000\u0000\u0000\n\u0000\u0000\u0000\u0010\u0000\u0000\u0000\u0000Stn7õû7C¬G\u0016:`\u000eÔ\u001dÙ\u0000²\u0004é\tìøB~\u0000\u0000@\u0000\u0000\u0000\u0000\u0000\u0000\u0000\u0000\u0010\u0000\u0000\u0000\u0000\u0000\u0000\u0000\u0000\u0000\u0000\u0000\u0000\u0000\u0000\u0000\u0000\u0000\u0000\u0000(\u0000\u0001LVCC\u0019System Waveform Chart.ctl\u0000\u0000\u0000\u0000\u0000\u0000\u0000\u0003\u0000\u0000\u0000\u0002\u0000\u0001\u0000\u0000\u0000\u0000\u0000\"\u0000\u000f\u0000\u0002\u0010\u0000\u0010\u0001 \u0000\u0010\u0010 \u0000 \u0000 \u0000 \u0000\u0010\u0000\u0010\u0004\u0010\u00000\u0000\u0010\u0000\u0010\b\u0010\u0000\u0000\u0000\u0000\u0000\u0000Õ\u0000\u0000\u0002þxc`À\u0004ÿ\u0000H120°¸Üèâÿ¡\u0000V\u0001²¹Øì Â^F Ã9\u0018Àl\u0007\u0006\bÍ\u0016_¢`\u0000WÂÀ ÐÀ³\u0000ÓT\u0007¸BÜö \u000bS\n²%$37\u0015ÂåtÌ-ÈÉ,)MIedH\u000bA\u0015>|ø\u0010nüK$F~Æ\b0[\u0018L2£È[2X0¼gH\u001aÏ\u0001´\u0005ÉJt\u001a« 6¯8D¢ñM 4\u000b¶ÿÝëh Ñ\u0017Uà\nÔ\u001c\u00154¾\bª¹DÿÁ\u00114ãP\u0003\u0019\f °\u0001'\u0000\u0004 .@VÅÄÖÒ\u0000\u000bq? \u0000\u0000\u0000\u0000\u0000\u0000(\u0000\u0001VIDS\u0019System Waveform Chart.ctl\u0000\u0000\u0000\u0000\u0000\u0000\u0000\u0003\u0000\u0000\u00011\u0000\u0000\u0002\u0004x\u000bcd`È4¶0\u000b¤a 9?%\u0015D\u0000½f=<!´;G#80(,¼»DEa\u0007HAçV\u0007V\u0006æc\f...", "RSRC\r\n\u0000\u0003LVCCLBVW\u0000\u0000C\u0000\u0000\u0004\u000e\u0000\u0000\u0000 \u0000\u0000C`\u0000\u0000\u0000x\t\u0000\u0000\u0000\u0000\u0000\u0000 \u0000\u0000\u0000\u0000\u0000\u0000\u0004\u0000\u0003\u0000<\u0000¼\u0000\u001f@\u0000\u0002\u0000\u0000\u0000\u0000\u0001\u0000\u0001\u0000\u0006ÿÿÿÿ\u0000\u0000\u0000\u0000\u0000\u0000\u0000\u0000\u0000\u0000\u0000\u0000 ¿FE\u001bÎN¯\u0019ÁêÜ¯¾\u0000\u0000\u0000\n\u0000\u0000\u0000\u0010\u0000\u0000\u0000\u0000íBÉzÆE=I¸awg\u001d8(¦Ô\u001dÙ\u0000²\u0004é\tìøB~\u0000\u0000@\u0000\u0000\u0000\u0000\u0000\u0000\u0000\u0000\u0010\u0000\u0000\u0000\u0000\u0000\u0000\u0000\u0000\u0000\u0000\u0000\u0000\u0000\u0000\u0000\u0000\u0000\u0000\u0000(\u0000\u0001LVCC\u0019System Waveform Graph.ctl\u0000\u0000\u0000\u0000\u0000\u0000\u0000\u0003\u0000\u0000\u0000\u0002\u0000\u0001\u0000\u0000\u0000\u0000\u0000*\u0000\u0013\u0000\u0002\u0010\u0000\u0010\u0001 \u0000 \u0000 \u0000 \u0000 \u0000\u0010\u0000\u0000\u0004\u0010\u00000\u0000\u0000\b\u0010\u0000\u0010\b\u0010\u0000\u0010\u0000\u0010\u0000\u0010\u0000\u0010\u0000\u0000\u0000\u0000\u0000\u0000Ô\u0000\u0000\u0002òxc`À\u0004ÿ\u0000H120°¸\\èâÿ¡\u0000V\u0001²¹Øì Â^F Ã9\u0018Àl\u0007\u0006\bÍ\u0016_¢`\u0000WÂÀ ÐÀ³\u0000ÓT\u0007¸BÜö \u000bS\n²%$37\u0011,Âé[YR\u0002å31\b13<|øáË/`ÞK$F~Æ\b0[\u0018¼%\u0005Ã{\u0014¨ñ0«Ði¬Ø¼à\u0010Æ7Ò,\u0010Úþ\u0003\u001e#@\u001a£/ªÀ\u0001\u0015¨9*h|\u0011Ts4ÿ\u0019#N9`|±Â\u0003Y ¾d)\u0000â\n¨<P\u0013F\u0000]DÖ\u0000\u0000\u0000(\u0000\u0001VIDS\u0019System Waveform Graph.ctl\u0000\u0000\u0000\u0000\u0000\u0000\u0000\u0003\u0000\u0000\u0001\u000b\u0000\u0000\u0001Ìx\u000bcd`È4¶0ë\u0005Ò0\n¢w\u0000Å^3ÄÇEEFÇ\u001e\u0010Ú£Â\u0011\u001c\u0018\u0014\u0016Þ]¢¢Ò]£¢ÑÍf\u000bR...", "RSRC\r\n\u0000\u0003LVCCLBVW\u0000\u0000Ch\u0000\u0000\u0004\b\u0000\u0000\u0000 \u0000\u0000CH\u0000\u0000\u0000x\t\u0000\u0000\u0000\u0000\u0000\u0000 \u0000\u0000\u0000\u0000\u0000\u0000\u0004\u0000\u0003\u0000<\u0000¼\u0000\u001f@\u0000\u0002\u0000\u0000\u0000\u0000\u0001\u0000\u0001\u0000\u0006ÿÿÿÿ\u0000\u0000\u0000\u0000\u0000\u0000\u0000\u0000\u0000\u0000\u0000\u0000\\/sgÖ©ãEÞØ&\u001b·2\u0000\u0000\u0000\n\u0000\u0000\u0000\u0010\u0000\u0000\u0000\u0000ÄûG\\y\u0011N°\u000bW§ænÔ\u001dÙ\u0000²\u0004é\tìøB~\u0000\u0000@\u0000\u0000\u0000\u0000\u0000\u0000\u0000\u0000\u0010\u0000\u0000\u0000\u0000\u0000\u0000\u0000\u0000\u0000\u0000\u0000\u0000\u0000\u0000\u0000\u0000\u0000\u0000\u0000\"\u0000\u0001LVCC\u0013System XY Graph.ctl\u0000\u0000\u0000\u0000\u0000\u0000\u0000\u0003\u0000\u0000\u0000\u0000\u0000\u0002\u0000\u0001\u0000\u0000\u0000\u0000\u00000\u0000\u0016\u0000\u0002\u0010\u0000\u0010\u0001 \u0000 \u0000 \u0000 \u0000 \u0000\u0010\u0000\u0000\u0004\u0010\u00000\u0000\u0000\b\u0010\u0000\u0010\b\u0010\u0000\u0010\u0000\u0010\u0000\u0010\u0000\u0010\u0000\u0010\b\u0010\u0000\u0010\u0000\u0000\u0000\u0000É\u0000\u0000\u0002òxc`À\u0004ÿ\u0000H120°¸\\èâÿ¡\u0000V\u0001²¹Øì Â^F Ã9\u0018 <\bÍ\u0016_¢`\u0000W\u0002TÐÀ³\u0000ÓT\u0007¸BÜö \u000bS\n²%$37\u0011,Âé[YR\u0002å31\b13ÌÉÀðåË\u0017°^k\u0004ÆDÆd°0¦<%5£#C\u0012ÔxUè4VAl^pPAåÛÒ'gÀ,\u0018\u0000HaÆ.A\u001dó\u0019-\u0018\u001cqJ\u0002ã%\u0001\u0012,\u0010_²\u0014\u0000q\u0005T^\u0000ÈfäÄ¢\u0011\u0000kGs\u0000\u0000\u0000\u0000\u0000\u0000\"\u0000\u0001VIDS\u0013System XY Graph.ctl\u0000\u0000\u0000\u0000\u0000\u0000\u0000\u0003\u0000\u0000\u0000\u0000\u00014\u0000\u0000\u00024x;ÈÈÀilaö\u0003HÃ@r~J*V`b`xÍ\u0010\u001f\u0017\u0015\u0019\u001d{xBhw\nGp`PXxwJwF7-HY©ôñV\u000fVÖ} ...", "RSRC\r\n\u0000\u0003LVCCLBVW\u0000\u0000¤\u0000\u0000\u0004$\u0000\u0000\u0000 \u0000\u0000\u0000\u0000\u0000x\t\u0000\u0000\u0000\u0000\u0000\u0000 \u0000\u0000\u0000\u0000\u0000\u0000\u0004\u0000\u0003\u0000<\u0000¼\u0000\u001f@\u0000\u0002\u0000\u0000\u0000\u0000\u0001\u0000\u0001\u0000\u0006ÿÿÿÿ\u0000\u0000\u0000\u0000\u0000\u0000\u0000\u0000\u0000\u0000\u0000\u0000'¹4ÙJ$Dq2>¥ \u0000\u0000\u0000\n\u0000\u0000\u0000\u0010\u0000\u0000\u0000\u0000v2kw\u0004|M°i7ûmºª\u0011Ô\u001dÙ\u0000²\u0004é\tìøB~\u0000\u0000@\u0000\u0000\u0000\u0000\u0000\u0000\u0000\u0000\u0010\u0000\u0000\u0000\u0000\u0000\u0000\u0000\u0000\u0000\u0000\u0000\u0000\u0000\u0000\u0000\u0000\u0000\u0000\u0000\u001e\u0000\u0001LVCC\u000fSystem Dial.ctl\u0000\u0000\u0000\u0000\u0000\u0000\u0000\u0003\u0000\u0000\u0000\u0000\u0000\u0002\u0000\u0001\u0000\u0000\u0000\u0000\u0000\u0016\u0000\t\u0000\u0002\u0010\u0000\u0010\u0001 \u0000\u0010\u0000\u0010\u0004\u0010\u00000\u0000\u0010\b\u0010\u0000\u0000\u0000\u0000\u0000\u0000f\u0000\u0000\u0001xxc`À\u0004ÿ\u0000H120°¸lèâÿ¡\u0000V\u0001²¹Øì Ö^\u0007\u0015T¾ý\u0007(}\u0001\u000fWÏU÷ó¶ÒE\u0007¡5çÿMdØÈpÁ-@·00@\u0002\u0001\u001cfÌ\t@\\¬\u0005N\u0000GÜ,\u0017\u0000\u0000\u0000\u0000\u0000\u001e\u0000\u0001VIDS\u000fSystem Dial.ctl\u0000\u0000\u0000\u0000\u0000\u0000\u0000\u0003\u0000\u0000\u0000\u0000\u0000 \u0000\u0000\u0000àxËb``È4¶0[È\u0000Éù)© ú\f\u0010¿f=<!´;G#80(,¼»DE¥»FEã.Û]ö'ïÝ\f¸ÿ`^D5á·¯9vtòO9PÅ^Êº\u0011ÈÆ¢¿a\u0016P¦ÓMc\u0012vØ\u0005¦]B_´÷¦¨°À´M\u0004ò\u000f\u0002Í\u0001\u0019õ\u001f\b@ò\fÌ\f\u0015\f\r\f\u001d\f(ÀÙßÅ\u0015\u000fr?\u0000¨ô:{\u0000\u0000\u0000\r\t\u0001\u0011\u0000\u0000\u00059.0.1\u0000\u0000\u0000\u0000\u0000\u0000\u0000\u0000\u0000\u0000\u0000\u0000\u0000\u0000\u0000\u0000\u0000\u0000\u0000\u0000\u0000\u0000\u0000\u0000\u0000\u0000\u0000...", "RSRC\r\n\u0000\u0003LVCCLBVW\u0000\u0000°\b\u0000\u0000\u00049\u0000\u0000\u0000 \u0000\u0000¯è\u0000\u0000\u0000x\t\u0000\u0000\u0000\u0000\u0000\u0000 \u0000\u0000\u0000\u0000\u0000\u0000\u0004\u0000\u0003\u0000<\u0000¼\u0000\u001f@\u0000\u0002\u0000\u0000\u0000\u0000\u0001\u0000\u0001\u0000\u0006ÿÿÿÿ\u0000\u0000\u0000\u0000\u0000\u0000\u0000\u0000\u0000\u0000\u0000\u0000Öª>Ú\t\u0003ÏImû²T\u0015[\u0000\u0000\u0000\n\u0000\u0000\u0000\u0010\u0000\u0000\u0000\u0000¤\u0001¤øjC­\u0010\u001bÅè\u0005µåÔ\u001dÙ\u0000²\u0004é\tìøB~\u0000\u0000@\u0000\u0000\u0000\u0000\u0000\u0000\u0000\u0000\u0010\u0000\u0000\u0000\u0000\u0000\u0000\u0000\u0000\u0000\u0000\u0000\u0000\u0000\u0000\u0000\u0000\u0000\u0000\u0000 \u0000\u0001LVCC\u0010System Gauge.ctl\u0000\u0000\u0000\u0000\u0000\u0000\u0000\u0000\u0003\u0000\u0000\u0000\u0002\u0000\u0001\u0000\u0000\u0000\u0000\u0000\u0016\u0000\t\u0000\u0002\u0010\u0000\u0010\u0001 \u0000\u0010\u0000\u0010\u0004\u0010\u00000\u0000\u0010\b\u0010\u0000\u0000\u0000\u0000\u0000\u0000g\u0000\u0000\u0001xxc`À\u0004ÿ\u0000H120°¸lèâÿ¡\u0000V\u0001²¹Øì Ö^\u0007\u0015T¾ý\u0007(ý\u0000\u000fW/è\u001esawÞ5\u0007Ñ¿{VfJ1ä2D1\u0013²\u0011è\u0016æ\u0010\u0006H@q\u0000ùÀ0cN\u0000â\u0002dU,Xt\u0002\u0000¯x*\u0000\u0000\u0000\u0000 \u0000\u0001VIDS\u0010System Gauge.ctl\u0000\u0000\u0000\u0000\u0000\u0000\u0000\u0000\u0003\u0000\u0000\u0000 \u0000\u0000\u0000àxËb``È4¶0[È\u0000Éù)© ú\f\u0010¿f=<!´;G#80(,¼»DE¥»FEã.Û]ö'ïÝ\f¸ÿ`^D5á·¯9vtòO9PÅ^Êº\u0011ÈÆ¢¿a\u0016P¦ÓMc\u0012vØ\u0005¦]B_´÷¦¨°À´M\u0004ò\u000f\u0002Í\u0001\u0019õ\u001f\b@ò\fÌ\f\u0015\f\r\f\u001d\f(ÀÙßÅ\u0015\u000fr?\u0000¨ô:{\u0000\u0000\u0000\r\t\u0001\u0011\u0000\u0000\u00059.0.1\u0000\u0000\u0000\u0000\u0000\u0000\u0000\u0000\u0000\u0000\u0000\u0000\u0000\u0000\u0000\u0000\u0000\u0000\u0000\u0000\u0000\u0000\u0004\u0000\u0000\u0000\u0010...", "RSRC\r\n\u0000\u0003LVCCLBVW\u0000\u0000-,\u0000\u0000\u0004\u0019\u0000\u0000\u0000 \u0000\u0000-\f\u0000\u0000\u0000x\t\u0000\u0000\u0000\u0000\u0000\u0000 \u0000\u0000\u0000\u0000\u0000\u0000\u0004\u0000\u0003\u0000<\u0000¼\u0000\u001f@\u0000\u0002\u0000\u0000\u0000\u0000\u0001\u0000\u0001\u0000\u0006ÿÿÿÿ\u0000\u0000\u0000\u0000\u0000\u0000\u0000\u0000\u0000\u0000\u0000\u0000Nîäþb«K«³|R©\u0000\u0000\u0000\n\u0000\u0000\u0000\u0010\u0000\u0000\u0000\u0000\u0002ø*,~>N²(Å«þt3Ô\u001dÙ\u0000²\u0004é\tìøB~\u0000\u0000@\u0000\u0000\u0000\u0000\u0000\u0000\u0000\u0000\u0010\u0000\u0000\u0000\u0000\u0000\u0000\u0000\u0000\u0000\u0000\u0000\u0000\u0000\u0000\u0000\u0000\u0000\u0000\u0000 \u0000\u0001LVCC\u0010System Meter.ctl\u0000\u0000\u0000\u0000\u0000\u0000\u0000\u0000\u0003\u0000\u0000\u0000\u0002\u0000\u0001\u0000\u0000\u0000\u0000\u0000\u0016\u0000\t\u0000\u0002\u0010\u0000\u0010\u0001 \u0000\u0010\u0000\u0010\u0004\u0010\u00000\u0000\u0010\b\u0010\u0000\u0000\u0000\u0000\u0000\u0000t\u0000\u0000\u0001¨xc`À\u0004ÿ\u0000H120°¸lèâÿ¡\u0000V\u0001²¹Øì Ö^\u0007\u0015ì|\u0007\u0016\bmÿ\u0001MIíÈÑé~iößÂEvÎðdØÆÐÄa,\u000buþüy\u0007\u0011$¶\u0002ÌHvc¸\u0011(Â\u001c\u00025\u0003È\u00071s\u0002\u0010\u0017`·\u0004\u0001\u0000-z1\u0015\u0000\u0000\u0000 \u0000\u0001VIDS\u0010System Meter.ctl\u0000\u0000\u0000\u0000\u0000\u0000\u0000\u0000\u0003\u0000\u0000\u0000 \u0000\u0000\u0000àxËb``È4¶0[È\u0000Éù)© ú\f\u0010¿f=<!´;G#80(,¼»DE¥»FEã.Û]ö'ïÝ\f¸ÿ`^D5á·¯9vtòO9PÅ^Êº\u0011ÈÆ¢¿a\u0016P¦ÓMc\u0012vØ\u0005¦]B_´÷¦¨°À´M\u0004ò\u000f\u0002Í\u0001\u0019õ\u001f\b@ò\fÌ\f\u0015\f\r\f\u001d\f(ÀÙßÅ\u0015\u000fr?\u0000¨ô:{\u0000\u0000\u0000\r\t\u0001\u0011\u0000\u0000\u00059.0.1\u0000\u0000\u0000\u0000\u0000\u0000\u0000\u0000\u0000\u0000\u0000\u0000\u0000\u0000\u0000...", "RSRC\r\n\u0000\u0003LVCCLBVW\u0000\u0000/Ô\u0000\u0000\u0003¸\u0000\u0000\u0000 \u0000\u0000/´\u0000\u0000\u0000x\t\u0000\u0000\u0000\u0000\u0000\u0000 \u0000\u0000\u0000\u0000\u0000\u0000\u0004\u0000\u0003\u0000<\u0000¼\u0000\u001f@\u0000\u0002\u0000\u0000\u0000\u0000\u0001\u0000\u0001\u0000\u0006ÿÿÿÿ\u0000\u0000\u0000\u0000\u0000\u0000\u0000\u0000\u0000\u0000\u0000\u0000\u0017*\u0016é[\u0001A´ÇÞZ¯\u000f\u0000\u0000\u0000\n\u0000\u0000\u0000\u0010\u0000\u0000\u0000\u0000¸¶+_EDiMm3Tx\rÌ'Ô\u001dÙ\u0000²\u0004é\tìøB~\u0000\u0000@\u0000\u0000\u0000\u0000\u0000\u0000\u0000\u0000\u0010\u0000\u0000\u0000\u0000\u0000\u0000\u0000\u0000\u0000\u0000\u0000\u0000\u0000\u0000\u0000\u0000\u0000\u0000\u0000.\u0000\u0001LVCC\u001fSystem String (Transparent).ctl\u0000\u0000\u0000\u0000\u0000\u0000\u0000\u0003\u0000\u0000\u0000\u0000\u0000\u0002\u0000\u0001\u0000\u0000\u0000\u0000\u0000\u0014\u0000\b\u0000\u0002\u0010\u0000\u0010\u0001\u0010\u0000\u0000\u0004\u0010\u00000\u0000\u0000\b\u0010\u0000\u0000\u0000\u0000E\u0000\u0000\u0001\u0014xc`À\u0004ÿ\u0000H12007\u0000iVtñÿPE+Å\u0000Ù\\lv`/P\u001dÓ\u0013 Í\fÄ,\f`ÿ0}\u0000â\u001fPy \u001dF\u0000\u0006{ U\u0000\u0000\u0000\u0000\u0000\u0000.\u0000\u0001VIDS\u001fSystem String (Transparent).ctl\u0000\u0000\u0000\u0000\u0000\u0000\u0000\u0003\u0000\u0000\u0000\u0000\u0000\u0000\u0000\u0000äxËd``È4¶0[À\u0000Éù)© ú\u0002\u0010¿f=<!´;G#80(,¼»DE¥»FEã¿ù³\u0017 ½)*\u001c¶ Æ\u000eF QÂº\u0003Ä.e\u0005ó°h/eØ¡\u0005étÓØ¡\u0004¦\u001dvdiPq,0m@¾\t\u0013\u0003Ã\u0004 }\u0010h\u001eÈÈÿ@\u0000RÇÈÀÌPÎPÏÐävg\u0017W$.Ø\u000f\u0000Çá2ó\u0000\u0000\u0000\u000b\t\u0000$\u0000\u0000\u00039.0\u0000\u0000\u0000\u0000\u0000\u0000\u0000\u0000\u0000\u0000\u0000\u0000\u0000\u0000\u0000\u0000\u0000\u0000\u0000\u0000\u0000\u0000\u0000\u0000\u0000\u0000\u0000\u0000\u0000\u0000\u0000\u0000\u0000\u0000\u0000\u0000\u0000\u0000\u0000\u0000\u0000..."], ["RSRC\r\n\u0000\u0003LMNULBVW\u0000\u0000\u0006¬\u0000\u0000\u0002$\u0000\u0000\u0000 \u0000\u0000\u0006\u0000\u0000\u0000\u0000\u0000\u0000\u0000\u0000\u0000\u0000\u0000\u000fÿÿÿ \u0000\u0000\u0000 \u0000\u0000\u0000 \u0000\u0000\u0000 \u0000\u0000\u0000 \u0000\u0000\u0000 \u0000\u000e\u0000 \u0000\u000e\u0000 \u0000\u001c\u0000 \u00008\u0000 @0\u0000  `\u0000 \u0010@\u0000 \u0000\u0000\u0000 \u0000\u0000\u0000 \u0000\u0000\u0000 \u0000\u0000\u0000 \u0000\u0000\u0000 \u0000\u0000\u0000 \u0000\u0000\u0000\u001fÿÿÿ\u0000\u0000\u0000\u0000\u0000\u0000\u0000\u0000\u0000\u0000\u0000\u0000\u0000\u0000\u0000\u0000\u0000\u0000\u0000\u0000\u0000\u0000\u0000\u0000\u0000\u0000\u0000\u0000\u0000\u0000\u0000\u0000\u0000\u0000\u0000\u0000\u0000\u0000\u0004\u0000öööööööööööööööööööööööööööööööööööööööööööööööööööööööööööööööööööVúööúVöøøøøøøøøøøøøøøøøøøøøøøøøøøøööúöøøøøøøøøøøøøøøøøøøøøøøøøøøøøööøøøøøøøøøøøøøøøøøööøøøøøøøøøøööøööööööööööööööööPPööööööööööööøöööööööööööööööPPPPöööööööööööøööööööööööööööPQ{ {øööööööööööøöööööö++öööööPQu¡Å{+ööööööööööøööööö+PPPöööPQu¡{+öööööööööööøöööö+P,+PPöPPu {+ööööööööööööøööööø{uPPPPPuv{+öööööööööööööøöööö+P uPJPK...", "RSRC\r\n\u0000\u0003LMNULBVW\u0000\u0000\u00060\u0000\u0000\u0001Ü\u0000\u0000\u0000 \u0000\u0000\u0006\u0010\u0000\u0000\u0000€ÿÿþ\u0000‚\u0002\u0002\u0000’\"b\u0000‚b\u0012\u0000’\"\"\u0000’\"B\u0000’\"r\u0000‚\u0002\u0002\u0000ÿÿþ\u0000\u0002\u0002\u0002\u0000\u0002bR\u0000\u0002\u0012R\u0000\u0002\"r\u0000\u0002\u0012\u0012\u0000\u0002b\u0012\u0000\u0002\u0002\u0002\u0000\u0003ÿþ\u0000\u0000\u0000\u0000\u0000\u0000\u0000\u0000\u0000\u0000\u0000ÿþpp€\u0002`0€\u0002e0¾zb0¾ze0¾z`0€ze0Ÿzb0Ÿze0Ÿ\u0002`0Ÿ\u0002pp€\u0002\u0000\u0000ÿþ\u0000\u0000\u0004\u0000¬¬¬¬¬¬¬¬¬¬¬¬¬¬¬¬¬¬¬¬¬¬¬öööööööö\u0000¬\u0000\u0000\u0000\u0000\u0000¬\u0000\u0000\u0000\u0000\u0000\u0000\u0000¬\u0000\u0000\u0000\u0000\u0000\u0000\u0000¬öööööööö\u0000¬\u0000\u0000ÿ\u0000\u0000¬\u0000\u0000\u0000ÿ\u0000\u0000\u0000¬\u0000\u0000ÿÿ\u0000\u0000\u0000¬öööööööö\u0000¬\u0000\u0000\u0000\u0000\u0000¬\u0000\u0000ÿÿ\u0000\u0000\u0000¬\u0000\u0000\u0000\u0000ÿ\u0000\u0000¬öööööööö\u0000¬\u0000\u0000ÿ\u0000\u0000¬\u0000\u0000\u0000ÿ\u0000\u0000\u0000¬\u0000\u0000\u0000ÿ\u0000\u0000\u0000¬öööööööö\u0000¬\u0000\u0000ÿ\u0000\u0000ÿ\u0000\u0000\u0000ÿ\u0000\u0000\u0000ÿ\u0000\u0000ÿ\u0000\u0000\u0000\u0000ÿöööööööö\u0000¬\u0000\u0000ÿ\u0000\u0000¬\u0000\u0000\u0000ÿ\u0000\u0000\u0000¬\u0000\u0000ÿÿÿ\u0000\u0000¬öööööööö\u0000¬\u0000\u0000\u0000\u0000\u0000¬\u0000\u0000\u0000\u0000\u0000\u0000\u0000¬\u0000\u0000\u0000\u0000\u0000\u0000\u0000¬öööööööö\u0000¬¬¬¬¬¬¬¬¬¬¬¬¬¬¬¬¬¬¬¬¬¬¬öööööööö\u0000öööööö¬\u0000\u0000\u0000\u0000\u0000\u0000\u0000¬\u0000\u0000\u0000\u0000\u0000\u0000\u0000¬öööööööö\u0000öööööö¬\u0000\u0000ÿÿ\u0000\u0000\u0000¬\u0000\u0000ÿ\u0000ÿ\u0000\u0000¬öööööööö\u0000öööööö¬\u0000\u0000\u0000\u0000ÿ\u0000\u0000¬\u0000\u0000ÿ\u0000ÿ\u0000\u0000¬öööööööö\u0000öööööö¬\u0000\u0000\u0000ÿ\u0000\u0000\u0000¬\u0000\u0000ÿÿÿ\u0000\u0000¬öööööööö\u0000öööööö¬\u0000\u0000\u0000\u0000ÿ\u0000\u0000¬\u0000...", "RSRC\r\n\u0000\u0003LMNULBVW\u0000\u0000\u0006,\u0000\u0000\u0001”\u0000\u0000\u0000 \u0000\u0000\u0006\f\u0000\u0000\u0000€\u0000\u0000\u0000\u0000\u0000\u0000\u0000\u0000\u0000\u0007\u0000\u0000\u0000\u001fÀ\u0000\u00000@\u0000\u0000'\u0000\u0000\u0000o€\u0000\u0000o€\u0000\u0000o€\u0000\u0000'\u0000\u0000\u00000\u0000\u0000\u0000\u0000\u0000\u0000\u0000\u0000\u0000\u0000\u0000\u0000\u0000\u0000\u0000\u0000\u0000\u0000\u0000\u0000\u0000\u0000\u0000\u0000\u0000\u0000\u0000ø\u0000\u0000ð\u0000\u0000`\u0000\u0000\u0000`@\u0000\u0000`À\u0000\u0000i€\u0000\u0000o\u0000\u0000\u0000f\u0000\u0000\u0000`\u0000\u0000\u0000`\u0000\u0000\u0000`\u0000\u0000\u0000@\u0000\u0000\u0000\u0000\u0000\u0000\u0000\u0000\u0000\u0000\u0000\u0000\u0000\u0000\u0000\u0000\u0004\u0000öööööööööööööööööööööööööööööööööööööööööööööööööööööööööööööööööööööööööøøøøüüüöööööööööööööööööööööööööøøüüüüüüüöööööööööööööööööööööööøüüöööööüöööööööööööööööööööööööøüööÿÿÿöööööööööööööööööööööööööüüöÿÿÿÿÿöøööööööööööööööööööööööüüöÿÿÿÿÿöøööööööööööööööööööööööüüöÿÿÿÿÿöøöööööööööööööööööööööööüööÿÿÿööööööööööööööööööööööööööüüöööööøöööööööööööööööööööööööööööøøøöööööööööööööööööööööööööööööööööööööööööööööööööööööööööööööööö...", "RSRC\r\n\u0000\u0003LMNULBVW\u0000\u0000\u0007ì\u0000\u0000\u0001Ó\u0000\u0000\u0000 \u0000\u0000\u0007Ì\u0000\u0000\u0000\u0000\u0000\u0000\u0000\u0000\u0000\u0000\u0000\u000fÿÿÿ \u0000\u0000\u0000 \u0000\u0000\u0000 \u0000\u0000\u0000 \u0000\u0000\u0000 \u0000\u0000\u0000 \u0000\u0000\u0000 \u0000\u0000\u0000 \u0000\u0000\u0000 \u0000\u0000\u0000 \u0000\u0000\u0000 \u0000\u0001\u0000 \u0000\u0000\u0000 \u0000\u0001\u0000 \u0000\u0001\u0000 \u0002\u0001\u0000 \u0000\u0001\u0000 \u0000\u0003\u0000 \u0000\u0000\u0000 \u0000\u0000\u0000\u001fÿÿÿ\u0000\u0000\u0000\u0000\u0000\u0000\u0000\u0000\u0000\u0000\u0000\u0000\u0000\u0000\u0000\u0000\u0000\u0000\u0000\u0000\u0000\u0000\u0000\u0000\u0000\u0000\u0000\u0000\u0000\u0000\u0000\u0000\u0000\u0000\u0000\u0000\u0000\u0000\u0004\u0000öööööööööööööööööööööööööööööööööööööööööööööööööööööööööööööööööööVúööúVöøøøøøøøøøøøøøøøøøøøøøøøøøøøööúöøøøø*NNNNNNNUUUUyOøøøøøøøøøøööøøøøøN\u0000\u0000\u0000\u0000\u0000\u0000\u0000\u0000\u0000\u0000\u0000\u0000yøøøøøøøøøøööøööööN\u0000PPPPPPPQQu\u0000yööööööööööööøööööN\u0000öööööööööö\u0000yööööööööööööøööööN\u0000NNNNNNNNNN\u0000yööööööööööööøööööN\u0000NöNöööNööööyööööööööööööøööööO\u0000NNNNyyyUyyyyy+ööööööööööøööööU\u0000NöNöyNö+ööööNyööööööööööøööööU\u0000N***yNöyöö\u0000\u0000UyööööööööööøööööU\u0000*ö*öyN...", "RSRC\r\n\u0000\u0003LMNULBVW\u0000\u0000\bÀ\u0000\u0000\u0001å\u0000\u0000\u0000 \u0000\u0000\b \u0000\u0000\u0000\u0000\u0000\u000f\u0000\u0000\u0000 \u0000\u0000\u0018\u0000\u0001\u0000\f\u0000\u0000\u0000\u0004\u0000\u0002\u0000\u0006\u0000\u0000þ\u0000\u0005ðÿ\u0000\u0007øÿ@\u0007øÿD\u0007øÿ$\u0007øÿ\u0000\u0003øÿ\u0000\u0003øÿ\u0000\u000bøÿ\u0000\u0001øý\u0000\u0000ðy\u0000\u0000ñ\u0000\u0006\u001fÁ\u0000\u0000\u0000\u0001\u0000\u0000\u0000\u0011\u0000\u00001\u0000\u0000\u00001\u0000\u0000\b\u0001\u0000\u0000\b\u0001\u0000\u0000\u0000\u0001\u0000\u0000\u001fÿ\u0000\u0000\u0010\u0000\u0007ÿð\u0000\u0000\u0000\u0000\u0000\u0000\u0000\u0000\u0000\u0000\u0000\u0000\u0000\u0000\u0000\u0004\u0000öööööööööööööööööö*yy*ööööööööööööööööööööööyyyUUyUyy£yööööööööööööööööööööyNUyUNUyUU£ööööööööööööööööööUOyyyöööyyyU££ööööööööööööööööyyUyyyy\u0000ö\u0000yyyyy£yöööööööööööööö*UyyyyyO*UyyyyyÇ+öööööööööööööyyyyyyy££Èyöööööööööööööy£££££Oöö*££££££¤£öøøøøöööööööö£ÇÇ££££\u0000öö££¤¤¤ÎÎÇöú++øøöööööö*££ÇÇÇÇÇÇöööÇÎÎÎÎÎÎÇöúV\u0000+úVVVVVVz££ÇÇÇÇÇÇöööÈÎÎÎÎÎÎÇööúö+úW\u0002\b\b\b\b,££ÇÇÇÇÇÇöööÈÎÎÎÎÎÎÇööøö+øV\u0001\u0001\u0001\u0001\u0001\u0001y£ÍÇÇÇÍÇöööÎÎÎÎÎÎÎ£ööøö+øV\u0001\u0001\u0001\u0001\u0001,z£È...", "RSRC\r\n\u0000\u0003LMNULBVW\u0000\u0000\u0005ô\u0000\u0000\u0001Ü\u0000\u0000\u0000 \u0000\u0000\u0005Ô\u0000\u0000\u0000\u0000\u0000\u0000\u0000\u0000\u0000\u0000\u0000\u0000\u0000\u0000\u0000\u0000\u0000\u0000\u0003\fÿÿó\u0002D!\u0003\u0004D!\u0003\u000eD!\u0003\u0000ÿã\u0000E!\u0003\u0000E!\u0003\u0000E¡\u0003\u0000E¡\u0003\u0004ÿÿã\fDc\u0003\u0004|%c\u0004D)\u0000D1\u0003\u0000ÿã\u0000D!\u0003\u0004D!\u0003\nD!\u0003\nÀ\u0000\u0003\u0004\u0010\u0010C\u0000D\u0001\u0013\u0000ª\u0003+\u0000ª\u0001+\u0000T\u0001S\u0000\u0000\u0000\u0003?ÿÿÿ\u0000\u0000\u0000\u0000\u0000\u0000\u0000\u0000\u0000\u0000\u0004\u0000öööööööööööööööööööööööööööööööööööööööööööööööööööööööööööööööööööööööööööööööööööööööööööööööööö+öööööööööööööööööööööööööööúüöö+öÿÿööÿüüüüüüüüüüüüüüüüüüüööúüöö+öööÿööü\u0000\u0000\u0000¥\u0000\u0000\u0000\u0000¥\u0000\u0000\u0000\u0000¥\u0000\u0000\u0000öööúüöö+ööÿöööü\u0000\u0000\u0000¥\u0000\u0000\u0000\u0000¥\u0000\u0000\u0000\u0000¥\u0000\u0000\u0000öööúüöö+öÿÿÿööü\u0000\u0000\u0000¥\u0000\u0000\u0000\u0000¥\u0000\u0000\u0000\u0000¥\u0000\u0000\u0000öööúüöö+ööööööü¥¥¥¥¥¥¥¥¥¥¥¥¥¥¥¥öööúüöö+ööööööü\u0000\u0000\u0000¥\u0000\u0000\u0000¥\u0000\u0000\u0000\u0000¥\u0000\u0000\u0000öööúüöö+ööööööü\u0000\u0000\u0000¥\u0000\u0000\u0000¥\u0000\u0000\u0000\u0000¥\u0000\u0000\u0000öööúüöö+ööööööü\u0000\u0000\u0000¥\u0000\u0000¥\u0000\u0000\u0000\u0000¥\u0000\u0000\u0000öööúüöö+ööööööü\u0000\u0000\u0000¥\u0000\u0000¥\u0000\u0000\u0000\u0000¥\u0000\u0000\u0000öööúüöö+ööÿööÿü¥¥¥¥¥...", "RSRC\r\n\u0000\u0003LMNULBVW\u0000\u0000\u0005¤\u0000\u0000\u0001”\u0000\u0000\u0000 \u0000\u0000\u0005„\u0000\u0000\u0000€\u0000\u0002\u0000\u0000\u0000\u0006\u0000\u0000\u0000\u0006\u0000\u0000\u001f\u0007ÿ€\u001f\u0007ÿ\u0000\u0010\u0006\u0000\u0000\u0000\u0006\u0000\u0000\u0000\f\u0000\u0000\u0000\b\u0000\u0000\u0000\u0018\u0000\u0000\u0000\u0010\u0000\u0000\bB\u0010€\bB\u0010€\b\u0000\u0000€\b\u0000\u0000€\u0000\u0000\u0000\u0000\u0000\u0000\u0000\u0000\u0000\u0000\u0000\u0000\u0000\u0000\u0000\u0000ÿÿøÿÿð`\u0000\u0000\u0000b\u0006\u0018\u0000f\t$\u0000b\u0001\u0004\u0000b\u0002\b\u0000b\u0004\u0004\u0000b\b$\u0000bO\u0018\u0000`\u0000\u0000\u0000@\u0000\u0000\u0000\u0000\u0000\u0000\u0000\u0000\u0000\u0004\u0000ööööööööööööööÿööööööööööööööööööööööööööøøøøúÿööööööööööööööööööööööööööøøøøúÿööööööööööööööööööööúúúúúöøøøøúÿúúúúúúúúúúööööööööööúÿÿÿÿöøøøøúÿÿÿÿÿÿÿÿÿÿøööööööööööúøøøøöøøøøúÿøøøøøøøøøøööööööööööööööööøøøøúÿöööööööööööööööööööööööööööøøúÿööööööööööööööööööööööööööööøøÿööööööööööööööööööööööööööööööúÿööööööööööööööööööööööööööööööÿööööööööööööööööööööööööÿööööÿööööÿööööÿööööÿöööööööööööÿööööÿööööÿööööÿööööÿöööööööööööÿööööööööööö...", "RSRC\r\n\u0000\u0003LMNULBVW\u0000\u0000\u0005|\u0000\u0000\u0001Ê\u0000\u0000\u0000 \u0000\u0000\u0005\\\u0000\u0000\u0000€ÿÿÿàÿÿÿÀ€\u0000\u0000\u0000€€\u0000\u0000€€\u0000\u0000Žã€\u0000’”\u0000\u0000’”\u0000\u0000Žã€\u0000€\u0000\u0000\u0000€\u0000\u0000\u0000\u0000\u0000\u0000\u0000\u0000\u0000\u0000\u0000\u0000\u0000\u0000\u0000\u0000\u0000\u0000\u0000\u0000\u0000\u0000\u0000?ÿÿþ?ÿÿü0\u0000\u0000\u00007€\u0000\u00004Ž\u0000\u00004‰\u0002@7É\u0002@0Nwp1è’H1(’H1(rH1à\u0000\u00000\u0000\u0000\u0000 \u0000\u0000\u0000\u0000\u0000\u0000\u0000\u0000\u0000\u0000\u0000\u0000\u0000\u0004\u0000¬¬¬¬¬¬¬¬¬¬¬¬¬¬¬¬¬¬¬¬¬¬¬¬¬¬¬ööööö¬¬¬¬¬¬¬¬¬¬¬¬¬¬¬¬¬¬¬¬¬¬¬¬¬¬øööööö¬öööööööööööööööööööööööööøööööö¬öööööööÿöööööööööööööööööøööööö¬öööööööÿöööööööööööööööööøööööö¬öööÿÿÿöÿÿÿöööÿÿÿöööööööööøööööö¬ööÿööÿöÿööÿöÿööööööööööööøööööö¬ööÿööÿöÿööÿöÿööööööööööööøööööö¬öööÿÿÿöÿÿÿöööÿÿÿöööööööööøööööö¬öööööööööööööööööööööööööøööööö¬öööööööööööööööööööööööööøöööööøøøøøøøøøøøøøøøøøøøøøøøøøøøööööööööööööööööööööööööööööööööööööööööööööööööööööö...", "", "", "", "", "", "", "", "", "", "", "", "", "", "", "", "", "", "", "", "", "", "", "", "", "", "", "", "", "", "", "", "", "", "", "", "", "", "", "", "", "", "", "", ""]]  # File Data
    w63 = path[][] [[path "C:/Program Files/National Instruments/LabVIEW 2009/menus/Controls/System 2.0", path "C:/Program Files/National Instruments/LabVIEW 2009/menus/Controls/System 2.0/Array & Cluster", path "C:/Program Files/National Instruments/LabVIEW 2009/menus/Controls/System 2.0/Boolean", path "C:/Program Files/National Instruments/LabVIEW 2009/menus/Controls/System 2.0/Boolean/System Buttons", path "C:/Program Files/National Instruments/LabVIEW 2009/menus/Controls/System 2.0/Boolean/Vertical Buttons", path "C:/Program Files/National Instruments/LabVIEW 2009/menus/Controls/System 2.0/Graphs & Charts", path "C:/Program Files/National Instruments/LabVIEW 2009/menus/Controls/System 2.0/Numeric", path "C:/Program Files/National Instruments/LabVIEW 2009/menus/Controls/System 2.0/String & Path", path "", path "", path ""], [path "C:/Users/shogg.AMER/Documents/LabVIEW Data/2009(32-bit)/Palettes/menus", path "C:/Users/shogg.AMER/Documents/LabVIEW Data/2009(32-bit)/Palettes/menus/Controls", path "C:/Users/shogg.AMER/Documents/LabVIEW Data/2009(32-bit)/Palettes/menus/Controls/System 2.0", path "C:/Users/shogg.AMER/Documents/LabVIEW Data/2009(32-bit)/Palettes/menus/Controls/System 2.0/Array & Cluster", path "C:/Users/shogg.AMER/Documents/LabVIEW Data/2009(32-bit)/Palettes/menus/Controls/System 2.0/Boolean", path "C:/Users/shogg.AMER/Documents/LabVIEW Data/2009(32-bit)/Palettes/menus/Controls/System 2.0/Boolean/System Buttons", path "C:/Users/shogg.AMER/Documents/LabVIEW Data/2009(32-bit)/Palettes/menus/Controls/System 2.0/Boolean/Vertical Buttons", path "C:/Users/shogg.AMER/Documents/LabVIEW Data/2009(32-bit)/Palettes/menus/Controls/System 2.0/Graphs & Charts", path "C:/Users/shogg.AMER/Documents/LabVIEW Data/2009(32-bit)/Palettes/menus/Controls/System 2.0/Numeric", path "C:/Users/shogg.AMER/Documents/LabVIEW Data/2009(32-bit)/Palettes/menus/Controls/System 2.0/String & Path", path "C:/Users/shogg.AMER/Documents/LabVIEW Data/2009(32-bit)/Palettes/menus/default"]]  # Folders
    w62 = i32[] [76, 70]  # Old Base Path Length
    # ">> Installed Versions of LabVIEW >>"
    # ">> Selected Version Path >>"
    n19 = for "Create new base paths" {
      tunnel: w57 -> [w164]
      tunnel: w60 -> [w163] mode=indexing
      tunnel: [w162] -> w61 mode=indexing
      n20 = Concatenate Strings ("Create New Base Path")(w164, w163) -> (w162:string)
    }
    n21 = for "Loop through all of the top level source folders" {
      tunnel: w65 -> [w135] mode=indexing
      tunnel: w64 -> [w141] mode=indexing
      tunnel: w63 -> [w140] mode=indexing
      tunnel: w62 -> [w139] mode=indexing
      tunnel: w61 -> [w138] mode=indexing
      tunnel: [w136] -> w59 mode=indexing
      n22 = for "Create necessary folder structure" {
        tunnel: w140 -> [w149] mode=indexing
        tunnel: w139 -> [w147]
        tunnel: w138 -> [w145]
        tunnel: [w143] -> w137
        n23 = Path To String(path=w149) -> (string=w148:string)
        n24 = String Subset(string=w148, offset (0)=w147) -> (substring=w144:string)  [unwired: 1 in]
        n25 = Concatenate Strings(w145, w144) -> (w146:string)
        n26 = String To Path(string=w146) -> (path=w142:path)
        n27 = Create Folder(path (use dialog)=w142) -> (error out=w143:errorcluster)  [unwired: 2 in, 2 out]
      }
      n28 = for "Write files" {
        tunnel: w135 -> [w153] mode=indexing
        tunnel: w141 -> [w154] mode=indexing
        tunnel: w138 -> [w151]
        tunnel: w137 -> [_]
        tunnel: [w150] -> w136 mode=indexing
        n29 = String Length(string=w153) -> (length=w152:i32)
        n30 = case shown="4.." w152 {
          tunnel: w153 -> [w158 _]
          tunnel: w154 -> [w159 _]
          tunnel: w151 -> [w157 _]
          tunnel: [w155 path ""] -> w150
          frame #0 {
            n31 = Concatenate Strings(w157, w158) -> (w156:string)
            n32 = String To Path(string=w156) -> (path=w155:path)
            n33 = Write to Binary File(file (use dialog)=w155, data=w159, 5:FALSE ("prepend array or string size? (T)")) -> ()  [unwired: 3 in, 3 out]
          }
          frame #1 {
            # "Don't write empty files,\nthat'd just be silly."
          }
        }
      }
    }
    n34 = for "Try to open an app reference to LabVIEW on the usual ports" {
      tunnel: w59 -> [w78]
      tunnel: [w76] -> w58
      tunnel: w57 -> [w75]
      tunnel: w56 -> [_] mode=indexing
      tunnel: w55 -> [w70]
      tunnel: w54 -> [w69]
      shift-right: [w67] -> w53
      shift-left: w52 -> [w66]
      i -> [w71]
      # ">> New Files >>"
      # "Start with the default\nport and cycle up for\nas many tries as there\nare installations of \nLabVIEW."
      n35 = Add(x=u16 3363 ("port number or service name (3363)"), y=w71) -> (x+y=w72:i32)
      n36 = Open Application Reference(10:w72, 11:"localhost" ("machine name (\"\":  open local reference)")) -> (0:w77:errorcluster, 3:w79:refnum<vi>)  [unwired: 2 in]
      n37 = String To Path(string=w75) -> (path=w74:path)
      n38 = case "Try to open up a VI server reference" shown="No Error" w77 {
        selector: w77 -> [w88 w134]
        tunnel: w79 -> [w96 _]
        tunnel: w74 -> [w95 _]
        tunnel: w78 -> [w90 _]
        tunnel: [w86 w134] -> w76
        tunnel: w70 -> [w85 _]
        tunnel: w69 -> [w82 _]
        tunnel: [w81 w133] -> w67
        tunnel: w66 -> [w80 w133]
        frame #0 {
          n39 = Array Size(array=w90) -> (size(s)=w92:i32[])
          n40 = property class="App"(reference=w96, error in=w88) -> (reference out=w93:refnum<vi>, error out=w87:errorcluster, "App.Dir"=w83:path, "App.Version"=w84:string)
          n41 = Multiply Array Elements(1:w92) -> (0:w91:i32)
          n42 = Reshape Array(w90, w91) -> (w89:path[])
          n43 = Equal?(x=w95, y=w83) -> (x = y?=w94:bool)
          n44 = case "If we lucked out and connected to the right version, mass compile and update palettes" shown="True" w94 {
            tunnel: w93 -> [_ w125]
            tunnel: w89 -> [_ w124]
            tunnel: w87 -> [w98 w102]
            tunnel: [w98 w122] -> w86
            tunnel: w85 -> [_ w120]
            tunnel: w84 -> [_ w119]
            tunnel: w83 -> [_ w111]
            tunnel: w82 -> [_ w108]
            tunnel: [w97 FALSE ("Restart needed?")] -> w81
            tunnel: w80 -> [w97 _]
            frame #0 {
            }
            frame #1 {
              w104 = T6 -2 items=["Functions"=-1, "Controls"=-2] ("palette type")
              # "Add the subpalette to the controls palette and refresh"
              n45 = call <vilib>:"Set Busy.vi"("error in (no error)"=w102) -> ("error out"=w101:errorcluster)  [unwired: 9 in, 1 out]
              n46 = for "Save all new files in this version (mass compile)" {
                tunnel: w124 -> [w127] mode=indexing
                shift-right: [w128] -> w123
                shift-left: w125 -> [w128]
                tunnel: w101 -> [w130]
                tunnel: [w129] -> _
                w126 = FALSE ("Save a Copy")
                n47 = Open VI Reference(application reference (local)=w128, vi path=w127, error in (no error)=w130) -> (vi reference=w131:refnum<vi>, error out=w132:errorcluster)  [unwired: 3 in]
                n48 = invoke class="VI" method="Save.Instrument"(reference=w131, error in=w132, "Path to saved file"=w127, "Save a Copy"=w126, "Without Diagram"=w126) -> (error out=w129:errorcluster)  [unwired: 1 in, 5 out]
              }
              n49 = Build Path(base path=w111, name or relative path="menus\\default\\root.mnu" ("String")) -> (appended path=w116:path)
              n50 = call <vilib>:"Read Palette.vi"("palette type"=w104, "palette path"=w116) -> ("palette data"=w106:T7, "duplicate palette path"=w118:path)  [unwired: 7 in, 1 out]
              n51 = Unbundle By Name(w106) -> ("items"=w110:T9)
              n52 = Build Path(base path=w111, name or relative path="\\Controls\\System 2.0\\dir.mnu") -> (appended path=w114:path)
              n53 = Bundle By Name(cluster=w108, "item path"=w114, "library path (.lvlib)"=path "", "short name"="Missing System Controls" ("String")) -> (w109:T1)
              n54 = Build Array (concatenate)(w110, w109) -> (w107:T9)
              n55 = Bundle By Name(cluster=w106, "items"=w107) -> (w105:T7)
              n56 = call <vilib>:"Write Palette.vi"("palette data"=w105, "palette type"=w104, "palette path"=w118) -> ("error out"=w100:errorcluster)  [unwired: 8 in]
              n57 = invoke class="App" method="Refresh Palettes"(reference=w123, error in=w100) -> (error out=w122:errorcluster)  [unwired: 1 in, 2 out]
              n58 = call <vilib>:"Unset Busy.vi"("error in (no error)"=w100) -> ("error out"=w99:errorcluster)  [unwired: 10 in]
              n59 = Concatenate Strings(w120, w119) -> (w121:string)
              n60 = call "Display Message to User"("error in (no error)"=w99, "Message"=w121) -> ()  [unwired: 8 in, 2 out]
            }
          }
        }
        frame #1 {
        }
      }
    }
    n61 = call <vilib>:"Clear Errors.vi"("error in (no error)"=w58) -> ()  [unwired: 6 in, 1 out]
  }
  n62 = call "Display Message to User2"("Enable"=w1) -> ()  [unwired: 9 in, 2 out]
